vi "Condition _string_4_prod_count_month_2.vi"(0 "Form Date":timestamp format="%<%Y-%m-%d>T", 1 "To Date":timestamp format="%<%Y-%m-%d>T", 3 "Shift":string(combo)="ALL", 4 "Select Station":string(combo)="ST 1", 5 "STACKHOLDER_ID":i32, 6 "Select Stakeholder":string(combo), 7 "Refnum out 2":T1, 9 "error in (no error)":errorcluster, 10 "Select Month":string(combo), 12 "Select Year":string(combo)) -> (11 "error out":errorcluster, 13 "Refnum out":T1, 14 "sum":i32[](array[numeric]), 15 "all table":string[][](array[string]), 16 "PROD COUNT_TEST":string[](array[string]), 17 "Table":string[][](array[string]), 18 "Elements Found out":string[](array[string]), 19 "Array 3":string[][](array[string]))   [LabVIEW 2017]
uses:
  <vilib>/addons/database/Connection.llb/Conn ObjectReference.ctl
  <vilib>/addons/database/NI_Database_API.lvlib
panel:
  out "data out":string[][](array[string])
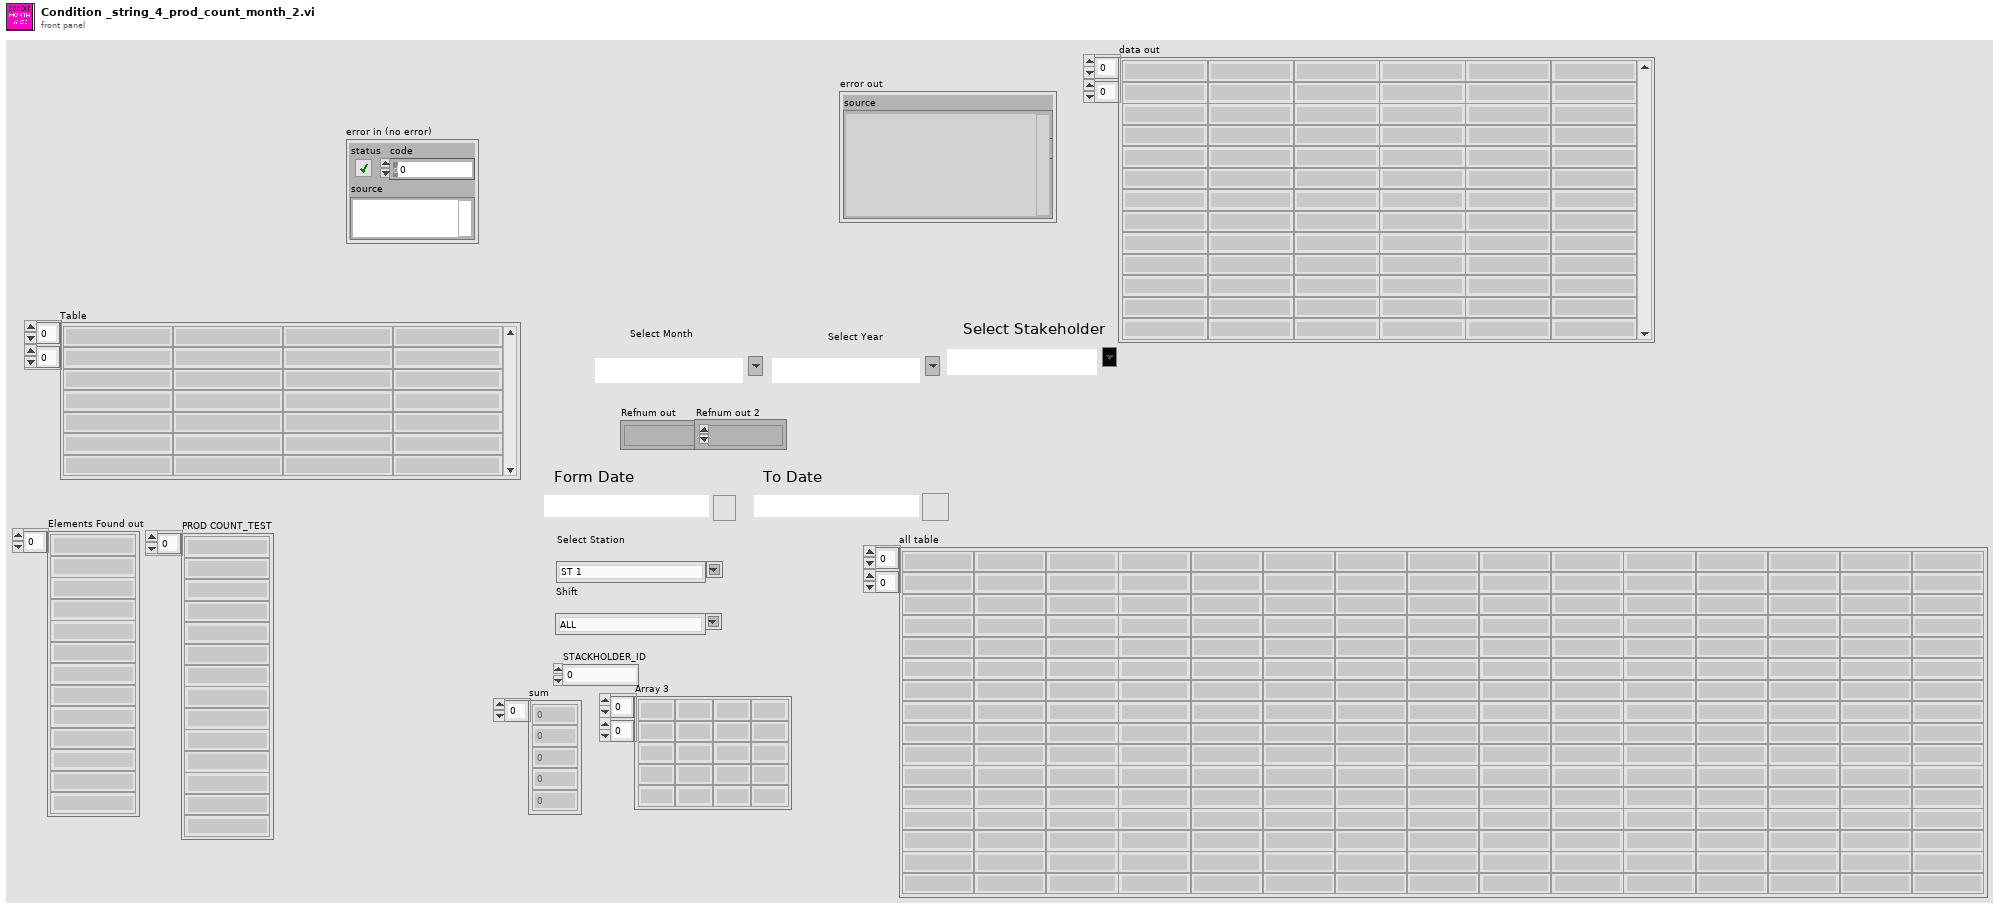
[diagram p1: front panel]
types:
  T1 = typedef "NI_Database_API.lvlib/Conn ObjectReference.ctl" = refnum<k1>
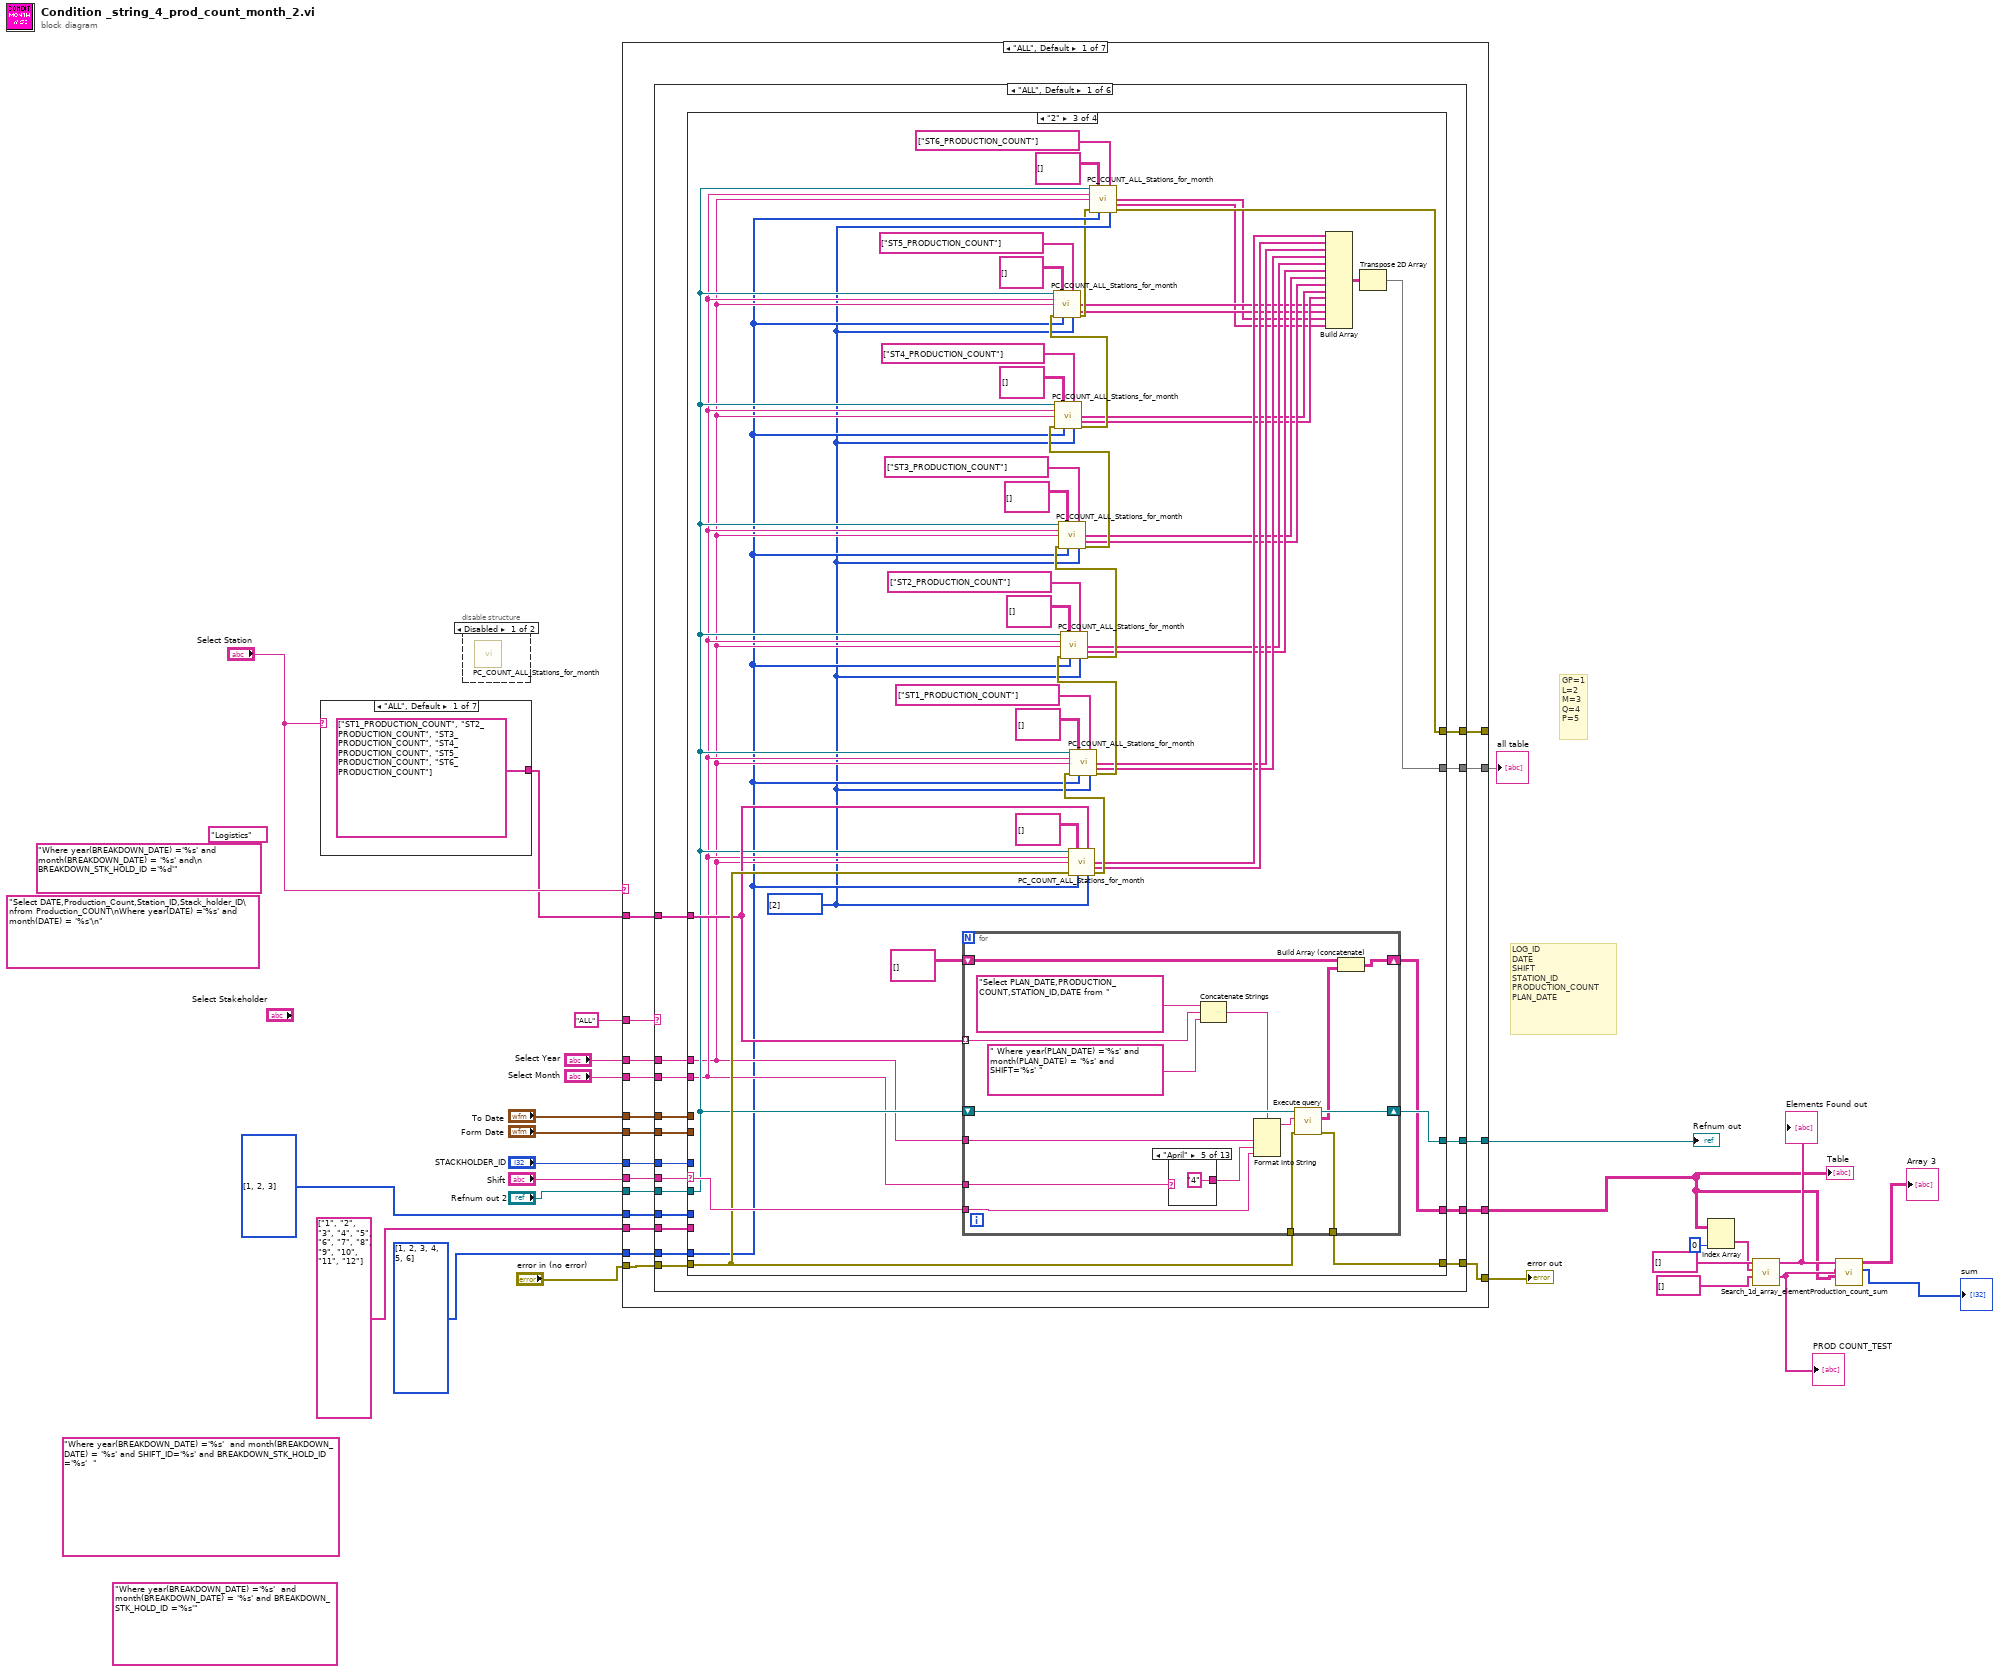
[diagram p0: block diagram]
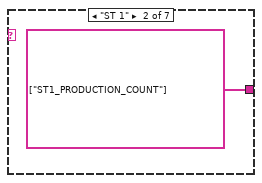
[diagram p3: hidden frame]
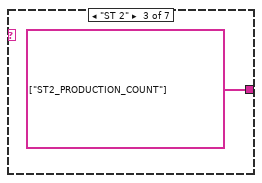
[diagram p4: hidden frame]
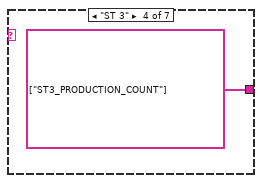
[diagram p5: hidden frame]
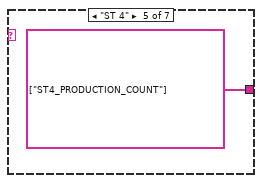
[diagram p6: hidden frame]
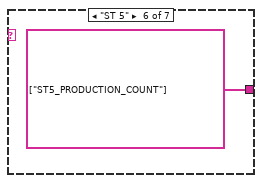
[diagram p7: hidden frame]
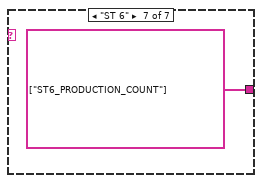
[diagram p8: hidden frame]
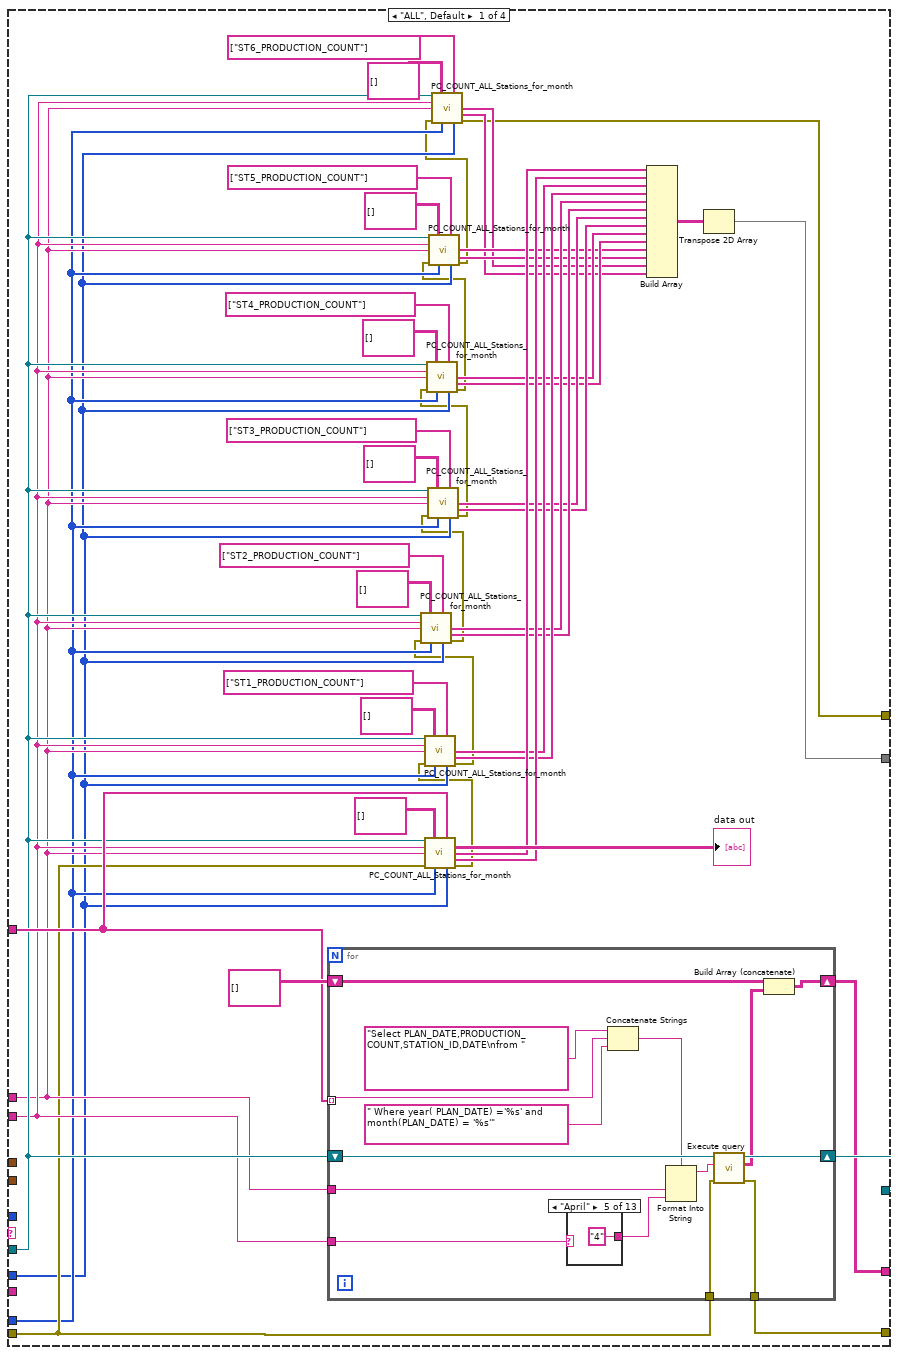
[diagram p9: hidden frame]
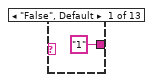
[diagram p10: hidden frame]
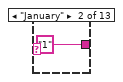
[diagram p11: hidden frame]
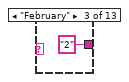
[diagram p12: hidden frame]
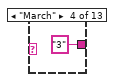
[diagram p13: hidden frame]
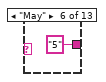
[diagram p14: hidden frame]
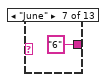
[diagram p15: hidden frame]
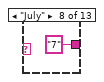
[diagram p16: hidden frame]
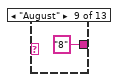
[diagram p17: hidden frame]
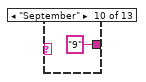
[diagram p18: hidden frame]
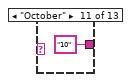
[diagram p19: hidden frame]
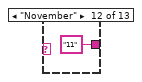
[diagram p20: hidden frame]
diagram:
  (unwired) "Select DATE,Production_Count,Station_ID,Stack_holder_ID\nfrom Production_COUNT\nWhere year(DATE) ='%s' and month(DATE) = '%s'\n" ("string")
  (unwired) "Where year(BREAKDOWN_DATE) ='%s' and month(BREAKDOWN_DATE) = '%s' and\n BREAKDOWN_STK_HOLD_ID ='%d'" ("condition")
  (unwired) "Logistics" ("Select Stakeholder")
  (unwired) "Where year(BREAKDOWN_DATE) ='%s'  and month(BREAKDOWN_DATE) = '%s' and BREAKDOWN_STK_HOLD_ID ='%s'" ("condition")
  (unwired) "Where year(BREAKDOWN_DATE) ='%s'  and month(BREAKDOWN_DATE) = '%s' and SHIFT_ID='%s' and BREAKDOWN_STK_HOLD_ID ='%s'  " ("condition")
  # "LOG_ID\nDATE\nSHIFT\nSTATION_ID\nPRODUCTION_COUNT\nPLAN_DATE"
  # "GP=1\nL=2\nM=3\nQ=4\nP=5"
  n1 = case shown="\"ALL\", Default" "Select Station" {
    tunnel: [string[] ["ST1_PRODUCTION_COUNT", "ST2_PRODUCTION_COUNT", "ST3_PRODUCTION_COUNT", "ST4_PRODUCTION_COUNT", "ST5_PRODUCTION_COUNT", "ST6_PRODUCTION_COUNT"] string[] ["ST1_PRODUCTION_COUNT"] string[] ["ST2_PRODUCTION_COUNT"] string[] ["ST3_PRODUCTION_COUNT"] string[] ["ST4_PRODUCTION_COUNT"] string[] ["ST5_PRODUCTION_COUNT"] string[] ["ST6_PRODUCTION_COUNT"]] -> w5
    frame "ALL", Default {
    }
    frame "ST 1" {
    }
    frame "ST 2" {
    }
    frame "ST 3" {
    }
    frame "ST 4" {
    }
    frame "ST 5" {
    }
    frame "ST 6" {
    }
  }
  n2 = disable-structure shown="Disabled" {
    frame Disabled {
      n3 = call "PC_COUNT_ALL_Stations_for_month.vi"() -> ()  [unwired: 11 in, 5 out]
    }
    frame Enabled {
    }
  }
  n4 = case shown="\"ALL\", Default" "Select Station" {
    tunnel: "Shift" -> [w51 w663 w1138 w1613 w2088 w2563 w3038]
    tunnel: "To Date" -> [w50 w662 w1137 w1612 w2087 w2562 w3037]
    tunnel: "Form Date" -> [w49 w661 w1136 w1611 w2086 w2561 w3036]
    tunnel: "STACKHOLDER_ID" -> [w48 w660 w1135 w1610 w2085 w2560 w3035]
    tunnel: "Refnum out 2" -> [w47 w659 w1134 w1609 w2084 w2559 w3034]
    tunnel: [w46 w658 w1133 w1608 w2083 w2558 w3033] -> w21
    tunnel: "ALL" -> [w45 w657 w1132 w1607 w2082 w2557 w3032]
    tunnel: i32[] [1, 2, 3, 4, 5, 6] -> [w44 _ _ _ _ _ _]
    tunnel: string[] ["1", "2", "3", "4", "5", "6", "7", "8", "9", "10", "11", "12"] -> [w43 _ _ _ _ _ _]
    tunnel: "Select Year" -> [w42 w656 w1131 w1606 w2081 w2556 w3031]
    tunnel: "Select Month" -> [w41 w655 w1130 w1605 w2080 w2555 w3030]
    tunnel: [w40 w654 w1129 w1604 w2079 w2554 w3029] -> w8
    tunnel: w5 -> [w39 w653 w1128 w1603 w2078 w2553 w3028]
    tunnel: "error in (no error)" -> [w38 w652 w1127 w1602 w2077 w2552 w3027]
    tunnel: [w37 w651 w1126 w1601 w2076 w2551 w3026] -> w3
    tunnel: i32[] [1, 2, 3] -> [w36 _ _ _ _ _ _]
    tunnel: [w35 _ _ _ _ _ _] -> w1
    tunnel: [w34 _ _ _ _ _ _] -> _
    frame "ALL", Default {
      n5 = case shown="\"ALL\", Default" w45 {
        tunnel: w51 -> [w68 w382 w437 w492 w547 w602]
        tunnel: w50 -> [w67 w381 w436 w491 w546 w601]
        tunnel: w49 -> [w66 w380 w435 w490 w545 w600]
        tunnel: w48 -> [w65 w379 w434 w489 w544 w599]
        tunnel: w47 -> [w64 w378 w433 w488 w543 w598]
        tunnel: [w63 w377 w432 w487 w542 w597] -> w46
        tunnel: w44 -> [w62 _ _ _ _ _]
        tunnel: w43 -> [w61 _ _ _ _ _]
        tunnel: w42 -> [w60 _ _ _ _ _]
        tunnel: w41 -> [w59 _ _ _ _ _]
        tunnel: [w58 _ _ _ _ _] -> w40
        tunnel: w39 -> [w57 _ _ _ _ _]
        tunnel: w38 -> [w56 w376 w431 w486 w541 w596]
        tunnel: [w55 w376 w431 w486 w541 w596] -> w37
        tunnel: w36 -> [w54 _ _ _ _ _]
        tunnel: [w53 _ _ _ _ _] -> w35
        tunnel: [w52 _ _ _ _ _] -> w34
        frame "ALL", Default {
          n6 = case shown="\"2\"" w68 {
            selector: w68 -> [_ w189 w266 w343]
            tunnel: w67 -> [_ _ _ _]
            tunnel: w66 -> [_ _ _ _]
            tunnel: w65 -> [_ _ _ _]
            tunnel: w64 -> [w83 w167 w244 w321]
            tunnel: [w116 w192 w269 w346] -> w63
            tunnel: w62 -> [w79 w164 w241 w318]
            tunnel: w61 -> [_ _ _ _]
            tunnel: w60 -> [w81 w165 w242 w319]
            tunnel: w59 -> [w82 w166 w243 w320]
            tunnel: [w114 w190 w267 w344] -> w58
            tunnel: w57 -> [w111 w185 w262 w339]
            tunnel: w56 -> [w80 w186 w263 w340]
            tunnel: [w113 w188 w265 w342] -> w55
            tunnel: w54 -> [w78 _ _ _]
            tunnel: [w106 w145 w222 w299] -> w53
            tunnel: [w69 w161 w238 w315] -> w52
            frame "ALL", Default {
              n7 = for {
                tunnel: w81 -> [w129]
                tunnel: w82 -> [w128]
                shift-right: [w130] -> w116
                shift-left: w83 -> [w131]
                tunnel: w111 -> [w124] mode=indexing
                shift-right: [w119] -> w114
                shift-left: string[][] [] -> [w121]
                tunnel: w80 -> [w118]
                tunnel: [w117] -> w113
                n8 = case shown="\"April\"" w128 {
                  tunnel: ["1" "1" "2" "3" "4" "5" "6" "7" "8" "9" "10" "11" "12"] -> w127
                  frame "False", Default {
                  }
                  frame "January" {
                  }
                  frame "February" {
                  }
                  frame "March" {
                  }
                  frame "April" {
                  }
                  frame "May" {
                  }
                  frame "June" {
                  }
                  frame "July" {
                  }
                  frame "August" {
                  }
                  frame "September" {
                  }
                  frame "October" {
                  }
                  frame "November" {
                  }
                  frame "December" {
                  }
                }
                n9 = Concatenate Strings("Select PLAN_DATE,PRODUCTION_COUNT,STATION_ID,DATE\nfrom ", w124, " Where year( PLAN_DATE) ='%s' and month(PLAN_DATE) = '%s'") -> (w122:string)
                n10 = Format Into String(format string=w122, w129, w127) -> (resulting string=w126:string)  [unwired: 2 in, 1 out]
                n11 = call "Execute query.vi"("error in (no error)"=w118, "String"=w126, "connection reference"=w131) -> ("error out"=w117:errorcluster, "Table"=w120:string[][], "connection reference 2"=w130:T1)  [unwired: 5 in, 1 out]
                n12 = Build Array (concatenate)(w121, w120) -> (w119:string[][])
              }
              n13 = call "PC_COUNT_ALL_Stations_for_month.vi"("Refnum in"=w83, "data in"=string[][] [] ("data"), "Array 3"=w111, "Select Month"=w82, "Select Year"=w81, "error in (no error)"=w80, "STATION"=w79, "SHIFT"=w78) -> ("data out"=→"data out":string[][], "DATE"=w109:string[], "COUNT"=w108:string[], "error out"=w75:errorcluster)  [unwired: 3 in, 1 out]
              n14 = call "PC_COUNT_ALL_Stations_for_month.vi"("Refnum in"=w83, "data in"=string[][] [] ("data"), "Array 3"=string[] ["ST1_PRODUCTION_COUNT"], "Select Month"=w82, "Select Year"=w81, "error in (no error)"=w75, "STATION"=w79, "SHIFT"=w78) -> ("DATE"=w103:string[], "COUNT"=w102:string[], "error out"=w74:errorcluster)  [unwired: 3 in, 2 out]
              n15 = call "PC_COUNT_ALL_Stations_for_month.vi"("Refnum in"=w83, "data in"=string[][] [] ("data"), "Array 3"=string[] ["ST2_PRODUCTION_COUNT"], "Select Month"=w82, "Select Year"=w81, "error in (no error)"=w74, "STATION"=w79, "SHIFT"=w78) -> ("DATE"=w99:string[], "COUNT"=w98:string[], "error out"=w73:errorcluster)  [unwired: 3 in, 2 out]
              n16 = call "PC_COUNT_ALL_Stations_for_month.vi"("Refnum in"=w83, "data in"=string[][] [] ("data"), "Array 3"=string[] ["ST3_PRODUCTION_COUNT"], "Select Month"=w82, "Select Year"=w81, "error in (no error)"=w73, "STATION"=w79, "SHIFT"=w78) -> ("DATE"=w95:string[], "COUNT"=w94:string[], "error out"=w72:errorcluster)  [unwired: 3 in, 2 out]
              n17 = call "PC_COUNT_ALL_Stations_for_month.vi"("Refnum in"=w83, "data in"=string[][] [] ("data"), "Array 3"=string[] ["ST4_PRODUCTION_COUNT"], "Select Month"=w82, "Select Year"=w81, "error in (no error)"=w72, "STATION"=w79, "SHIFT"=w78) -> ("DATE"=w91:string[], "COUNT"=w90:string[], "error out"=w71:errorcluster)  [unwired: 3 in, 2 out]
              n18 = call "PC_COUNT_ALL_Stations_for_month.vi"("Refnum in"=w83, "data in"=string[][] [] ("data"), "Array 3"=string[] ["ST5_PRODUCTION_COUNT"], "Select Month"=w82, "Select Year"=w81, "error in (no error)"=w71, "STATION"=w79, "SHIFT"=w78) -> ("DATE"=w87:string[], "COUNT"=w86:string[], "error out"=w70:errorcluster)  [unwired: 3 in, 2 out]
              n19 = call "PC_COUNT_ALL_Stations_for_month.vi"("Refnum in"=w83, "data in"=string[][] [] ("data"), "Array 3"=string[] ["ST6_PRODUCTION_COUNT"], "Select Month"=w82, "Select Year"=w81, "error in (no error)"=w70, "STATION"=w79, "SHIFT"=w78) -> ("DATE"=w77:string[], "COUNT"=w76:string[], "error out"=w69:errorcluster)  [unwired: 3 in, 2 out]
              n20 = Build Array(w109, w108, w103, w102, w99, w98, w95, w94, w91, w90, w87, w86, w77, w76) -> (w107:string[][])
              n21 = Transpose 2D Array(2D array=w107) -> (transposed array=w106:string[][])
            }
            frame "1" {
              w163 = i32[] [1]
              n22 = for {
                tunnel: w165 -> [w206]
                tunnel: w166 -> [w205]
                shift-right: [w207] -> w192
                shift-left: w167 -> [w208]
                tunnel: w185 -> [w201] mode=indexing
                shift-right: [w196] -> w190
                shift-left: string[][] [] -> [w198]
                tunnel: w189 -> [w195]
                tunnel: w186 -> [w194]
                tunnel: [w193] -> w188
                n23 = case shown="\"April\"" w205 {
                  tunnel: ["1" "1" "2" "3" "4" "5" "6" "7" "8" "9" "10" "11" "12"] -> w204
                  frame "False", Default {
                  }
                  frame "January" {
                  }
                  frame "February" {
                  }
                  frame "March" {
                  }
                  frame "April" {
                  }
                  frame "May" {
                  }
                  frame "June" {
                  }
                  frame "July" {
                  }
                  frame "August" {
                  }
                  frame "September" {
                  }
                  frame "October" {
                  }
                  frame "November" {
                  }
                  frame "December" {
                  }
                }
                n24 = Concatenate Strings("Select PLAN_DATE,PRODUCTION_COUNT,STATION_ID,DATE from ", w201, " Where year(PLAN_DATE) ='%s' and month(PLAN_DATE) = '%s' and SHIFT='%s' ") -> (w199:string)
                n25 = Format Into String(format string=w199, w206, w204, w195) -> (resulting string=w203:string)  [unwired: 2 in, 1 out]
                n26 = call "Execute query.vi"("error in (no error)"=w194, "String"=w203, "connection reference"=w208) -> ("error out"=w193:errorcluster, "Table"=w197:string[][], "connection reference 2"=w207:T1)  [unwired: 5 in, 1 out]
                n27 = Build Array (concatenate)(w198, w197) -> (w196:string[][])
              }
              n28 = call "PC_COUNT_ALL_Stations_for_month.vi"("Refnum in"=w167, "data in"=string[][] [], "Array 3"=w185, "Select Month"=w166, "Select Year"=w165, "error in (no error)"=w186, "STATION"=w164, "SHIFT"=w163) -> ("DATE"=w160:string[], "COUNT"=w159:string[], "error out"=w184:errorcluster)  [unwired: 3 in, 2 out]
              n29 = call "PC_COUNT_ALL_Stations_for_month.vi"("Refnum in"=w167, "data in"=string[][] [], "Array 3"=string[] ["ST1_PRODUCTION_COUNT"], "Select Month"=w166, "Select Year"=w165, "error in (no error)"=w184, "STATION"=w164, "SHIFT"=w163) -> ("DATE"=w158:string[], "COUNT"=w157:string[], "error out"=w179:errorcluster)  [unwired: 3 in, 2 out]
              n30 = call "PC_COUNT_ALL_Stations_for_month.vi"("Refnum in"=w167, "data in"=string[][] [], "Array 3"=string[] ["ST2_PRODUCTION_COUNT"], "Select Month"=w166, "Select Year"=w165, "error in (no error)"=w179, "STATION"=w164, "SHIFT"=w163) -> ("DATE"=w156:string[], "COUNT"=w155:string[], "error out"=w178:errorcluster)  [unwired: 3 in, 2 out]
              n31 = call "PC_COUNT_ALL_Stations_for_month.vi"("Refnum in"=w167, "data in"=string[][] [], "Array 3"=string[] ["ST3_PRODUCTION_COUNT"], "Select Month"=w166, "Select Year"=w165, "error in (no error)"=w178, "STATION"=w164, "SHIFT"=w163) -> ("DATE"=w154:string[], "COUNT"=w153:string[], "error out"=w175:errorcluster)  [unwired: 3 in, 2 out]
              n32 = call "PC_COUNT_ALL_Stations_for_month.vi"("Refnum in"=w167, "data in"=string[][] [], "Array 3"=string[] ["ST4_PRODUCTION_COUNT"], "Select Month"=w166, "Select Year"=w165, "error in (no error)"=w175, "STATION"=w164, "SHIFT"=w163) -> ("DATE"=w152:string[], "COUNT"=w151:string[], "error out"=w170:errorcluster)  [unwired: 3 in, 2 out]
              n33 = call "PC_COUNT_ALL_Stations_for_month.vi"("Refnum in"=w167, "data in"=string[][] [], "Array 3"=string[] ["ST5_PRODUCTION_COUNT"], "Select Month"=w166, "Select Year"=w165, "error in (no error)"=w170, "STATION"=w164, "SHIFT"=w163) -> ("DATE"=w150:string[], "COUNT"=w149:string[], "error out"=w162:errorcluster)  [unwired: 3 in, 2 out]
              n34 = call "PC_COUNT_ALL_Stations_for_month.vi"("Refnum in"=w167, "data in"=string[][] [], "Array 3"=string[] ["ST6_PRODUCTION_COUNT"], "Select Month"=w166, "Select Year"=w165, "error in (no error)"=w162, "STATION"=w164, "SHIFT"=w163) -> ("DATE"=w148:string[], "COUNT"=w147:string[], "error out"=w161:errorcluster)  [unwired: 3 in, 2 out]
              n35 = Build Array(w160, w159, w158, w157, w156, w155, w154, w153, w152, w151, w150, w149, w148, w147) -> (w146:string[][])
              n36 = Transpose 2D Array(2D array=w146) -> (transposed array=w145:string[][])
            }
            frame "2" {
              w240 = i32[] [2]
              n37 = for {
                tunnel: w242 -> [w283]
                tunnel: w243 -> [w282]
                shift-right: [w284] -> w269
                shift-left: w244 -> [w285]
                tunnel: w262 -> [w278] mode=indexing
                shift-right: [w273] -> w267
                shift-left: string[][] [] -> [w275]
                tunnel: w266 -> [w272]
                tunnel: w263 -> [w271]
                tunnel: [w270] -> w265
                n38 = case shown="\"April\"" w282 {
                  tunnel: ["1" "1" "2" "3" "4" "5" "6" "7" "8" "9" "10" "11" "12"] -> w281
                  frame "False", Default {
                  }
                  frame "January" {
                  }
                  frame "February" {
                  }
                  frame "March" {
                  }
                  frame "April" {
                  }
                  frame "May" {
                  }
                  frame "June" {
                  }
                  frame "July" {
                  }
                  frame "August" {
                  }
                  frame "September" {
                  }
                  frame "October" {
                  }
                  frame "November" {
                  }
                  frame "December" {
                  }
                }
                n39 = Concatenate Strings("Select PLAN_DATE,PRODUCTION_COUNT,STATION_ID,DATE from ", w278, " Where year(PLAN_DATE) ='%s' and month(PLAN_DATE) = '%s' and SHIFT='%s' ") -> (w276:string)
                n40 = Format Into String(format string=w276, w283, w281, w272) -> (resulting string=w280:string)  [unwired: 2 in, 1 out]
                n41 = call "Execute query.vi"("error in (no error)"=w271, "String"=w280, "connection reference"=w285) -> ("error out"=w270:errorcluster, "Table"=w274:string[][], "connection reference 2"=w284:T1)  [unwired: 5 in, 1 out]
                n42 = Build Array (concatenate)(w275, w274) -> (w273:string[][])
              }
              n43 = call "PC_COUNT_ALL_Stations_for_month.vi"("Refnum in"=w244, "data in"=string[][] [], "Array 3"=w262, "Select Month"=w243, "Select Year"=w242, "error in (no error)"=w263, "STATION"=w241, "SHIFT"=w240) -> ("DATE"=w237:string[], "COUNT"=w236:string[], "error out"=w261:errorcluster)  [unwired: 3 in, 2 out]
              n44 = call "PC_COUNT_ALL_Stations_for_month.vi"("Refnum in"=w244, "data in"=string[][] [], "Array 3"=string[] ["ST1_PRODUCTION_COUNT"], "Select Month"=w243, "Select Year"=w242, "error in (no error)"=w261, "STATION"=w241, "SHIFT"=w240) -> ("DATE"=w235:string[], "COUNT"=w234:string[], "error out"=w256:errorcluster)  [unwired: 3 in, 2 out]
              n45 = call "PC_COUNT_ALL_Stations_for_month.vi"("Refnum in"=w244, "data in"=string[][] [], "Array 3"=string[] ["ST2_PRODUCTION_COUNT"], "Select Month"=w243, "Select Year"=w242, "error in (no error)"=w256, "STATION"=w241, "SHIFT"=w240) -> ("DATE"=w233:string[], "COUNT"=w232:string[], "error out"=w255:errorcluster)  [unwired: 3 in, 2 out]
              n46 = call "PC_COUNT_ALL_Stations_for_month.vi"("Refnum in"=w244, "data in"=string[][] [], "Array 3"=string[] ["ST3_PRODUCTION_COUNT"], "Select Month"=w243, "Select Year"=w242, "error in (no error)"=w255, "STATION"=w241, "SHIFT"=w240) -> ("DATE"=w231:string[], "COUNT"=w230:string[], "error out"=w252:errorcluster)  [unwired: 3 in, 2 out]
              n47 = call "PC_COUNT_ALL_Stations_for_month.vi"("Refnum in"=w244, "data in"=string[][] [], "Array 3"=string[] ["ST4_PRODUCTION_COUNT"], "Select Month"=w243, "Select Year"=w242, "error in (no error)"=w252, "STATION"=w241, "SHIFT"=w240) -> ("DATE"=w229:string[], "COUNT"=w228:string[], "error out"=w247:errorcluster)  [unwired: 3 in, 2 out]
              n48 = call "PC_COUNT_ALL_Stations_for_month.vi"("Refnum in"=w244, "data in"=string[][] [], "Array 3"=string[] ["ST5_PRODUCTION_COUNT"], "Select Month"=w243, "Select Year"=w242, "error in (no error)"=w247, "STATION"=w241, "SHIFT"=w240) -> ("DATE"=w227:string[], "COUNT"=w226:string[], "error out"=w239:errorcluster)  [unwired: 3 in, 2 out]
              n49 = call "PC_COUNT_ALL_Stations_for_month.vi"("Refnum in"=w244, "data in"=string[][] [], "Array 3"=string[] ["ST6_PRODUCTION_COUNT"], "Select Month"=w243, "Select Year"=w242, "error in (no error)"=w239, "STATION"=w241, "SHIFT"=w240) -> ("DATE"=w225:string[], "COUNT"=w224:string[], "error out"=w238:errorcluster)  [unwired: 3 in, 2 out]
              n50 = Build Array(w237, w236, w235, w234, w233, w232, w231, w230, w229, w228, w227, w226, w225, w224) -> (w223:string[][])
              n51 = Transpose 2D Array(2D array=w223) -> (transposed array=w222:string[][])
            }
            frame "3" {
              w317 = i32[] [3]
              n52 = for {
                tunnel: w319 -> [w360]
                tunnel: w320 -> [w359]
                shift-right: [w361] -> w346
                shift-left: w321 -> [w362]
                tunnel: w339 -> [w355] mode=indexing
                shift-right: [w350] -> w344
                shift-left: string[][] [] -> [w352]
                tunnel: w343 -> [w349]
                tunnel: w340 -> [w348]
                tunnel: [w347] -> w342
                n53 = case shown="\"April\"" w359 {
                  tunnel: ["1" "1" "2" "3" "4" "5" "6" "7" "8" "9" "10" "11" "12"] -> w358
                  frame "False", Default {
                  }
                  frame "January" {
                  }
                  frame "February" {
                  }
                  frame "March" {
                  }
                  frame "April" {
                  }
                  frame "May" {
                  }
                  frame "June" {
                  }
                  frame "July" {
                  }
                  frame "August" {
                  }
                  frame "September" {
                  }
                  frame "October" {
                  }
                  frame "November" {
                  }
                  frame "December" {
                  }
                }
                n54 = Concatenate Strings("Select PLAN_DATE,PRODUCTION_COUNT,STATION_ID,DATE from ", w355, " Where year(PLAN_DATE) ='%s' and month(PLAN_DATE) = '%s' and SHIFT='%s' ") -> (w353:string)
                n55 = Format Into String(format string=w353, w360, w358, w349) -> (resulting string=w357:string)  [unwired: 2 in, 1 out]
                n56 = call "Execute query.vi"("error in (no error)"=w348, "String"=w357, "connection reference"=w362) -> ("error out"=w347:errorcluster, "Table"=w351:string[][], "connection reference 2"=w361:T1)  [unwired: 5 in, 1 out]
                n57 = Build Array (concatenate)(w352, w351) -> (w350:string[][])
              }
              n58 = call "PC_COUNT_ALL_Stations_for_month.vi"("Refnum in"=w321, "data in"=string[][] [], "Array 3"=w339, "Select Month"=w320, "Select Year"=w319, "error in (no error)"=w340, "STATION"=w318, "SHIFT"=w317) -> ("DATE"=w314:string[], "COUNT"=w313:string[], "error out"=w338:errorcluster)  [unwired: 3 in, 2 out]
              n59 = call "PC_COUNT_ALL_Stations_for_month.vi"("Refnum in"=w321, "data in"=string[][] [], "Array 3"=string[] ["ST1_PRODUCTION_COUNT"], "Select Month"=w320, "Select Year"=w319, "error in (no error)"=w338, "STATION"=w318, "SHIFT"=w317) -> ("DATE"=w312:string[], "COUNT"=w311:string[], "error out"=w333:errorcluster)  [unwired: 3 in, 2 out]
              n60 = call "PC_COUNT_ALL_Stations_for_month.vi"("Refnum in"=w321, "data in"=string[][] [], "Array 3"=string[] ["ST2_PRODUCTION_COUNT"], "Select Month"=w320, "Select Year"=w319, "error in (no error)"=w333, "STATION"=w318, "SHIFT"=w317) -> ("DATE"=w310:string[], "COUNT"=w309:string[], "error out"=w332:errorcluster)  [unwired: 3 in, 2 out]
              n61 = call "PC_COUNT_ALL_Stations_for_month.vi"("Refnum in"=w321, "data in"=string[][] [], "Array 3"=string[] ["ST3_PRODUCTION_COUNT"], "Select Month"=w320, "Select Year"=w319, "error in (no error)"=w332, "STATION"=w318, "SHIFT"=w317) -> ("DATE"=w308:string[], "COUNT"=w307:string[], "error out"=w329:errorcluster)  [unwired: 3 in, 2 out]
              n62 = call "PC_COUNT_ALL_Stations_for_month.vi"("Refnum in"=w321, "data in"=string[][] [], "Array 3"=string[] ["ST4_PRODUCTION_COUNT"], "Select Month"=w320, "Select Year"=w319, "error in (no error)"=w329, "STATION"=w318, "SHIFT"=w317) -> ("DATE"=w306:string[], "COUNT"=w305:string[], "error out"=w324:errorcluster)  [unwired: 3 in, 2 out]
              n63 = call "PC_COUNT_ALL_Stations_for_month.vi"("Refnum in"=w321, "data in"=string[][] [], "Array 3"=string[] ["ST5_PRODUCTION_COUNT"], "Select Month"=w320, "Select Year"=w319, "error in (no error)"=w324, "STATION"=w318, "SHIFT"=w317) -> ("DATE"=w304:string[], "COUNT"=w303:string[], "error out"=w316:errorcluster)  [unwired: 3 in, 2 out]
              n64 = call "PC_COUNT_ALL_Stations_for_month.vi"("Refnum in"=w321, "data in"=string[][] [], "Array 3"=string[] ["ST6_PRODUCTION_COUNT"], "Select Month"=w320, "Select Year"=w319, "error in (no error)"=w316, "STATION"=w318, "SHIFT"=w317) -> ("DATE"=w302:string[], "COUNT"=w301:string[], "error out"=w315:errorcluster)  [unwired: 3 in, 2 out]
              n65 = Build Array(w314, w313, w312, w311, w310, w309, w308, w307, w306, w305, w304, w303, w302, w301) -> (w300:string[][])
              n66 = Transpose 2D Array(2D array=w300) -> (transposed array=w299:string[][])
            }
          }
        }
        frame "Logistics" {
          n67 = case shown="\"3\"" w382 {
            selector: w382 -> [_ _ w396 w408 w420]
            tunnel: w381 -> [_ w393 w405 w417 w429]
            tunnel: w380 -> [_ w392 w404 w416 w428]
            tunnel: w379 -> [_ _ _ _ _]
            tunnel: [_ w386 w398 w410 w422] -> _
            tunnel: w378 -> [w383 w389 w401 w413 w425]
            tunnel: [w383 w385 w397 w409 w421] -> w377
            frame "False", Default {
            }
            frame "ALL" {
              w394 = "%Y-%m-%d " ("time format string (%c)")
              n68 = Format Date/Time String(time format string (%c)=w394, seconds (now)=w392) -> (date/time string=w391:string)  [unwired: 1 in]
              n69 = Format Date/Time String(time format string (%c)=w394, seconds (now)=w393) -> (date/time string=w390:string)  [unwired: 1 in]
              n70 = Format Into String(format string="Select DATE,Production_Count,Station_ID,Stack_holder_ID\nfrom Production_COUNT\nWhere DATE between '%s' and '%s' and Stack_holder_ID='%d'" ("string"), w391, w390, 2 ("input 3")) -> (resulting string=w387:string)  [unwired: 2 in, 1 out]
              n71 = call "Execute query.vi"("String"=w387, "connection reference"=w389) -> ("Table"=w386:string[][], "connection reference 2"=w385:T1)  [unwired: 6 in, 2 out]
            }
            frame "1" {
              w406 = "%Y-%m-%d " ("time format string (%c)")
              n72 = Format Date/Time String(time format string (%c)=w406, seconds (now)=w405) -> (date/time string=w402:string)  [unwired: 1 in]
              n73 = Format Date/Time String(time format string (%c)=w406, seconds (now)=w404) -> (date/time string=w403:string)  [unwired: 1 in]
              n74 = Format Into String(format string="Select DATE,Production_Count,Station_ID,Stack_holder_ID\nfrom Production_COUNT\nWhere DATE between '%s' and '%s' and Shift_ID='%s'and Stack_holder_ID='%d'" ("string"), w403, w402, w396, 2 ("input 4")) -> (resulting string=w399:string)  [unwired: 2 in, 1 out]
              n75 = call "Execute query.vi"("String"=w399, "connection reference"=w401) -> ("Table"=w398:string[][], "connection reference 2"=w397:T1)  [unwired: 6 in, 2 out]
            }
            frame "2" {
              w418 = "%Y-%m-%d " ("time format string (%c)")
              n76 = Format Date/Time String(time format string (%c)=w418, seconds (now)=w417) -> (date/time string=w414:string)  [unwired: 1 in]
              n77 = Format Date/Time String(time format string (%c)=w418, seconds (now)=w416) -> (date/time string=w415:string)  [unwired: 1 in]
              n78 = Format Into String(format string="Select DATE,Production_Count,Station_ID,Stack_holder_ID\nfrom Production_COUNT\nWhere DATE between '%s' and '%s' and Shift_ID='%s'and Stack_holder_ID='%d'" ("string"), w415, w414, w408, 2 ("input 4")) -> (resulting string=w411:string)  [unwired: 2 in, 1 out]
              n79 = call "Execute query.vi"("String"=w411, "connection reference"=w413) -> ("Table"=w410:string[][], "connection reference 2"=w409:T1)  [unwired: 6 in, 2 out]
            }
            frame "3" {
              w430 = "%Y-%m-%d " ("time format string (%c)")
              n80 = Format Date/Time String(time format string (%c)=w430, seconds (now)=w429) -> (date/time string=w426:string)  [unwired: 1 in]
              n81 = Format Date/Time String(time format string (%c)=w430, seconds (now)=w428) -> (date/time string=w427:string)  [unwired: 1 in]
              n82 = Format Into String(format string="Select DATE,Production_Count,Station_ID,Stack_holder_ID\nfrom Production_COUNT\nWhere DATE between '%s' and '%s' and Shift_ID='%s'and Stack_holder_ID='%d'" ("string"), w427, w426, w420, 2 ("input 4")) -> (resulting string=w423:string)  [unwired: 2 in, 1 out]
              n83 = call "Execute query.vi"("String"=w423, "connection reference"=w425) -> ("Table"=w422:string[][], "connection reference 2"=w421:T1)  [unwired: 6 in, 2 out]
            }
          }
        }
        frame "Gap Leader" {
          n84 = case shown="\"3\"" w437 {
            selector: w437 -> [_ _ w451 w463 w475]
            tunnel: w436 -> [_ w448 w460 w472 w484]
            tunnel: w435 -> [_ w447 w459 w471 w483]
            tunnel: w434 -> [_ _ _ _ _]
            tunnel: [_ w441 w453 w465 w477] -> _
            tunnel: w433 -> [w438 w444 w456 w468 w480]
            tunnel: [w438 w440 w452 w464 w476] -> w432
            frame "False", Default {
            }
            frame "ALL" {
              w449 = "%Y-%m-%d " ("time format string (%c)")
              n85 = Format Date/Time String(time format string (%c)=w449, seconds (now)=w447) -> (date/time string=w446:string)  [unwired: 1 in]
              n86 = Format Date/Time String(time format string (%c)=w449, seconds (now)=w448) -> (date/time string=w445:string)  [unwired: 1 in]
              n87 = Format Into String(format string="Select DATE,Production_Count,Station_ID,Stack_holder_ID\nfrom Production_COUNT\nWhere DATE between '%s' and '%s' and Stack_holder_ID='%d'" ("string"), w446, w445, 1 ("input 3")) -> (resulting string=w442:string)  [unwired: 2 in, 1 out]
              n88 = call "Execute query.vi"("String"=w442, "connection reference"=w444) -> ("Table"=w441:string[][], "connection reference 2"=w440:T1)  [unwired: 6 in, 2 out]
            }
            frame "1" {
              w461 = "%Y-%m-%d " ("time format string (%c)")
              n89 = Format Date/Time String(time format string (%c)=w461, seconds (now)=w460) -> (date/time string=w457:string)  [unwired: 1 in]
              n90 = Format Date/Time String(time format string (%c)=w461, seconds (now)=w459) -> (date/time string=w458:string)  [unwired: 1 in]
              n91 = Format Into String(format string="Select DATE,Production_Count,Station_ID,Stack_holder_ID\nfrom Production_COUNT\nWhere DATE between '%s' and '%s' and Shift_ID='%s'and Stack_holder_ID='%d'" ("string"), w458, w457, w451, 1 ("input 4")) -> (resulting string=w454:string)  [unwired: 2 in, 1 out]
              n92 = call "Execute query.vi"("String"=w454, "connection reference"=w456) -> ("Table"=w453:string[][], "connection reference 2"=w452:T1)  [unwired: 6 in, 2 out]
            }
            frame "2" {
              w473 = "%Y-%m-%d " ("time format string (%c)")
              n93 = Format Date/Time String(time format string (%c)=w473, seconds (now)=w472) -> (date/time string=w469:string)  [unwired: 1 in]
              n94 = Format Date/Time String(time format string (%c)=w473, seconds (now)=w471) -> (date/time string=w470:string)  [unwired: 1 in]
              n95 = Format Into String(format string="Select DATE,Production_Count,Station_ID,Stack_holder_ID\nfrom Production_COUNT\nWhere DATE between '%s' and '%s' and Shift_ID='%s'and Stack_holder_ID='%d'" ("string"), w470, w469, w463, 1 ("input 4")) -> (resulting string=w466:string)  [unwired: 2 in, 1 out]
              n96 = call "Execute query.vi"("String"=w466, "connection reference"=w468) -> ("Table"=w465:string[][], "connection reference 2"=w464:T1)  [unwired: 6 in, 2 out]
            }
            frame "3" {
              w485 = "%Y-%m-%d " ("time format string (%c)")
              n97 = Format Date/Time String(time format string (%c)=w485, seconds (now)=w484) -> (date/time string=w481:string)  [unwired: 1 in]
              n98 = Format Date/Time String(time format string (%c)=w485, seconds (now)=w483) -> (date/time string=w482:string)  [unwired: 1 in]
              n99 = Format Into String(format string="Select DATE,Production_Count,Station_ID,Stack_holder_ID\nfrom Production_COUNT\nWhere DATE between '%s' and '%s' and Shift_ID='%s'and Stack_holder_ID='%d'" ("string"), w482, w481, w475, 1 ("input 4")) -> (resulting string=w478:string)  [unwired: 2 in, 1 out]
              n100 = call "Execute query.vi"("String"=w478, "connection reference"=w480) -> ("Table"=w477:string[][], "connection reference 2"=w476:T1)  [unwired: 6 in, 2 out]
            }
          }
        }
        frame "Maintenance" {
          n101 = case shown="\"ALL\"" w492 {
            selector: w492 -> [_ _ w506 w518 w530]
            tunnel: w491 -> [_ w503 w515 w527 w539]
            tunnel: w490 -> [_ w502 w514 w526 w538]
            tunnel: w489 -> [_ _ _ _ _]
            tunnel: [_ w496 w508 w520 w532] -> _
            tunnel: w488 -> [w493 w499 w511 w523 w535]
            tunnel: [w493 w495 w507 w519 w531] -> w487
            frame "False", Default {
            }
            frame "ALL" {
              w504 = "%Y-%m-%d " ("time format string (%c)")
              n102 = Format Date/Time String(time format string (%c)=w504, seconds (now)=w502) -> (date/time string=w501:string)  [unwired: 1 in]
              n103 = Format Date/Time String(time format string (%c)=w504, seconds (now)=w503) -> (date/time string=w500:string)  [unwired: 1 in]
              n104 = Format Into String(format string="Select DATE,Production_Count,Station_ID,Stack_holder_ID\nfrom Production_COUNT\nWhere DATE between '%s' and '%s' and Stack_holder_ID='%d'" ("string"), w501, w500, 3 ("input 3")) -> (resulting string=w497:string)  [unwired: 2 in, 1 out]
              n105 = call "Execute query.vi"("String"=w497, "connection reference"=w499) -> ("Table"=w496:string[][], "connection reference 2"=w495:T1)  [unwired: 6 in, 2 out]
            }
            frame "1" {
              w516 = "%Y-%m-%d " ("time format string (%c)")
              n106 = Format Date/Time String(time format string (%c)=w516, seconds (now)=w515) -> (date/time string=w512:string)  [unwired: 1 in]
              n107 = Format Date/Time String(time format string (%c)=w516, seconds (now)=w514) -> (date/time string=w513:string)  [unwired: 1 in]
              n108 = Format Into String(format string="Select DATE,Production_Count,Station_ID,Stack_holder_ID\nfrom Production_COUNT\nWhere DATE between '%s' and '%s' and Shift_ID='%s'and Stack_holder_ID='%d'" ("string"), w513, w512, w506, 3 ("input 4")) -> (resulting string=w509:string)  [unwired: 2 in, 1 out]
              n109 = call "Execute query.vi"("String"=w509, "connection reference"=w511) -> ("Table"=w508:string[][], "connection reference 2"=w507:T1)  [unwired: 6 in, 2 out]
            }
            frame "2" {
              w528 = "%Y-%m-%d " ("time format string (%c)")
              n110 = Format Date/Time String(time format string (%c)=w528, seconds (now)=w527) -> (date/time string=w524:string)  [unwired: 1 in]
              n111 = Format Date/Time String(time format string (%c)=w528, seconds (now)=w526) -> (date/time string=w525:string)  [unwired: 1 in]
              n112 = Format Into String(format string="Select DATE,Production_Count,Station_ID,Stack_holder_ID\nfrom Production_COUNT\nWhere DATE between '%s' and '%s' and Shift_ID='%s'and Stack_holder_ID='%d'" ("string"), w525, w524, w518, 3 ("input 4")) -> (resulting string=w521:string)  [unwired: 2 in, 1 out]
              n113 = call "Execute query.vi"("String"=w521, "connection reference"=w523) -> ("Table"=w520:string[][], "connection reference 2"=w519:T1)  [unwired: 6 in, 2 out]
            }
            frame "3" {
              w540 = "%Y-%m-%d " ("time format string (%c)")
              n114 = Format Date/Time String(time format string (%c)=w540, seconds (now)=w539) -> (date/time string=w536:string)  [unwired: 1 in]
              n115 = Format Date/Time String(time format string (%c)=w540, seconds (now)=w538) -> (date/time string=w537:string)  [unwired: 1 in]
              n116 = Format Into String(format string="Select DATE,Production_Count,Station_ID,Stack_holder_ID\nfrom Production_COUNT\nWhere DATE between '%s' and '%s' and Shift_ID='%s'and Stack_holder_ID='%d'" ("string"), w537, w536, w530, 3 ("input 4")) -> (resulting string=w533:string)  [unwired: 2 in, 1 out]
              n117 = call "Execute query.vi"("String"=w533, "connection reference"=w535) -> ("Table"=w532:string[][], "connection reference 2"=w531:T1)  [unwired: 6 in, 2 out]
            }
          }
        }
        frame "Quality" {
          n118 = case shown="\"3\"" w547 {
            selector: w547 -> [_ _ w561 w573 w585]
            tunnel: w546 -> [_ w558 w570 w582 w594]
            tunnel: w545 -> [_ w557 w569 w581 w593]
            tunnel: w544 -> [_ _ _ _ _]
            tunnel: [_ w551 w563 w575 w587] -> _
            tunnel: w543 -> [w548 w554 w566 w578 w590]
            tunnel: [w548 w550 w562 w574 w586] -> w542
            frame "False", Default {
            }
            frame "ALL" {
              w559 = "%Y-%m-%d " ("time format string (%c)")
              n119 = Format Date/Time String(time format string (%c)=w559, seconds (now)=w557) -> (date/time string=w556:string)  [unwired: 1 in]
              n120 = Format Date/Time String(time format string (%c)=w559, seconds (now)=w558) -> (date/time string=w555:string)  [unwired: 1 in]
              n121 = Format Into String(format string="Select DATE,Production_Count,Station_ID,Stack_holder_ID\nfrom Production_COUNT\nWhere DATE between '%s' and '%s' and Stack_holder_ID='%d'" ("string"), w556, w555, 4 ("input 3")) -> (resulting string=w552:string)  [unwired: 2 in, 1 out]
              n122 = call "Execute query.vi"("String"=w552, "connection reference"=w554) -> ("Table"=w551:string[][], "connection reference 2"=w550:T1)  [unwired: 6 in, 2 out]
            }
            frame "1" {
              w571 = "%Y-%m-%d " ("time format string (%c)")
              n123 = Format Date/Time String(time format string (%c)=w571, seconds (now)=w570) -> (date/time string=w567:string)  [unwired: 1 in]
              n124 = Format Date/Time String(time format string (%c)=w571, seconds (now)=w569) -> (date/time string=w568:string)  [unwired: 1 in]
              n125 = Format Into String(format string="Select DATE,Production_Count,Station_ID,Stack_holder_ID\nfrom Production_COUNT\nWhere DATE between '%s' and '%s' and Shift_ID='%s'and Stack_holder_ID='%d'" ("string"), w568, w567, w561, 4 ("input 4")) -> (resulting string=w564:string)  [unwired: 2 in, 1 out]
              n126 = call "Execute query.vi"("String"=w564, "connection reference"=w566) -> ("Table"=w563:string[][], "connection reference 2"=w562:T1)  [unwired: 6 in, 2 out]
            }
            frame "2" {
              w583 = "%Y-%m-%d " ("time format string (%c)")
              n127 = Format Date/Time String(time format string (%c)=w583, seconds (now)=w582) -> (date/time string=w579:string)  [unwired: 1 in]
              n128 = Format Date/Time String(time format string (%c)=w583, seconds (now)=w581) -> (date/time string=w580:string)  [unwired: 1 in]
              n129 = Format Into String(format string="Select DATE,Production_Count,Station_ID,Stack_holder_ID\nfrom Production_COUNT\nWhere DATE between '%s' and '%s' and Shift_ID='%s'and Stack_holder_ID='%d'" ("string"), w580, w579, w573, 4 ("input 4")) -> (resulting string=w576:string)  [unwired: 2 in, 1 out]
              n130 = call "Execute query.vi"("String"=w576, "connection reference"=w578) -> ("Table"=w575:string[][], "connection reference 2"=w574:T1)  [unwired: 6 in, 2 out]
            }
            frame "3" {
              w595 = "%Y-%m-%d " ("time format string (%c)")
              n131 = Format Date/Time String(time format string (%c)=w595, seconds (now)=w594) -> (date/time string=w591:string)  [unwired: 1 in]
              n132 = Format Date/Time String(time format string (%c)=w595, seconds (now)=w593) -> (date/time string=w592:string)  [unwired: 1 in]
              n133 = Format Into String(format string="Select DATE,Production_Count,Station_ID,Stack_holder_ID\nfrom Production_COUNT\nWhere DATE between '%s' and '%s' and Shift_ID='%s'and Stack_holder_ID='%d'" ("string"), w592, w591, w585, 4 ("input 4")) -> (resulting string=w588:string)  [unwired: 2 in, 1 out]
              n134 = call "Execute query.vi"("String"=w588, "connection reference"=w590) -> ("Table"=w587:string[][], "connection reference 2"=w586:T1)  [unwired: 6 in, 2 out]
            }
          }
        }
        frame "Production" {
          n135 = case shown="\"3\"" w602 {
            selector: w602 -> [_ _ w616 w628 w640]
            tunnel: w601 -> [_ w613 w625 w637 w649]
            tunnel: w600 -> [_ w612 w624 w636 w648]
            tunnel: w599 -> [_ _ _ _ _]
            tunnel: [_ w606 w618 w630 w642] -> _
            tunnel: w598 -> [w603 w609 w621 w633 w645]
            tunnel: [w603 w605 w617 w629 w641] -> w597
            frame "False", Default {
            }
            frame "ALL" {
              w614 = "%Y-%m-%d " ("time format string (%c)")
              n136 = Format Date/Time String(time format string (%c)=w614, seconds (now)=w612) -> (date/time string=w611:string)  [unwired: 1 in]
              n137 = Format Date/Time String(time format string (%c)=w614, seconds (now)=w613) -> (date/time string=w610:string)  [unwired: 1 in]
              n138 = Format Into String(format string="Select DATE,Production_Count,Station_ID,Stack_holder_ID\nfrom Production_COUNT\nWhere DATE between '%s' and '%s' and Stack_holder_ID='%d'" ("string"), w611, w610, 5 ("input 3")) -> (resulting string=w607:string)  [unwired: 2 in, 1 out]
              n139 = call "Execute query.vi"("String"=w607, "connection reference"=w609) -> ("Table"=w606:string[][], "connection reference 2"=w605:T1)  [unwired: 6 in, 2 out]
            }
            frame "1" {
              w626 = "%Y-%m-%d " ("time format string (%c)")
              n140 = Format Date/Time String(time format string (%c)=w626, seconds (now)=w625) -> (date/time string=w622:string)  [unwired: 1 in]
              n141 = Format Date/Time String(time format string (%c)=w626, seconds (now)=w624) -> (date/time string=w623:string)  [unwired: 1 in]
              n142 = Format Into String(format string="Select DATE,Production_Count,Station_ID,Stack_holder_ID\nfrom Production_COUNT\nWhere DATE between '%s' and '%s' and Shift_ID='%s'and Stack_holder_ID='%d'" ("string"), w623, w622, w616, 5 ("input 4")) -> (resulting string=w619:string)  [unwired: 2 in, 1 out]
              n143 = call "Execute query.vi"("String"=w619, "connection reference"=w621) -> ("Table"=w618:string[][], "connection reference 2"=w617:T1)  [unwired: 6 in, 2 out]
            }
            frame "2" {
              w638 = "%Y-%m-%d " ("time format string (%c)")
              n144 = Format Date/Time String(time format string (%c)=w638, seconds (now)=w637) -> (date/time string=w634:string)  [unwired: 1 in]
              n145 = Format Date/Time String(time format string (%c)=w638, seconds (now)=w636) -> (date/time string=w635:string)  [unwired: 1 in]
              n146 = Format Into String(format string="Select DATE,Production_Count,Station_ID,Stack_holder_ID\nfrom Production_COUNT\nWhere DATE between '%s' and '%s' and Shift_ID='%s'and Stack_holder_ID='%d'" ("string"), w635, w634, w628, 5 ("input 4")) -> (resulting string=w631:string)  [unwired: 2 in, 1 out]
              n147 = call "Execute query.vi"("String"=w631, "connection reference"=w633) -> ("Table"=w630:string[][], "connection reference 2"=w629:T1)  [unwired: 6 in, 2 out]
            }
            frame "3" {
              w650 = "%Y-%m-%d " ("time format string (%c)")
              n148 = Format Date/Time String(time format string (%c)=w650, seconds (now)=w649) -> (date/time string=w646:string)  [unwired: 1 in]
              n149 = Format Date/Time String(time format string (%c)=w650, seconds (now)=w648) -> (date/time string=w647:string)  [unwired: 1 in]
              n150 = Format Into String(format string="Select DATE,Production_Count,Station_ID,Stack_holder_ID\nfrom Production_COUNT\nWhere DATE between '%s' and '%s' and Shift_ID='%s'and Stack_holder_ID='%d'" ("string"), w647, w646, w640, 5 ("input 4")) -> (resulting string=w643:string)  [unwired: 2 in, 1 out]
              n151 = call "Execute query.vi"("String"=w643, "connection reference"=w645) -> ("Table"=w642:string[][], "connection reference 2"=w641:T1)  [unwired: 6 in, 2 out]
            }
          }
        }
      }
    }
    frame "ST 1" {
      n152 = case shown="\"ALL\", Default" w657 {
        tunnel: w663 -> [w675 w840 w899 w955 w1014 w1073]
        tunnel: w662 -> [w674 w839 w898 w954 w1013 w1072]
        tunnel: w661 -> [w673 w838 w897 w953 w1012 w1071]
        tunnel: w660 -> [w672 w837 w896 w952 w1011 w1070]
        tunnel: [w671 w836 w895 w951 w1010 w1069] -> w654
        tunnel: w659 -> [w670 w835 w894 w950 w1009 w1068]
        tunnel: [w669 w834 w893 w949 w1008 w1067] -> w658
        tunnel: w656 -> [w668 _ _ _ _ _]
        tunnel: w655 -> [w667 _ _ _ _ _]
        tunnel: w653 -> [w666 _ _ _ _ _]
        tunnel: w652 -> [w665 _ _ _ _ _]
        tunnel: [w664 _ _ _ _ _] -> w651
        frame "ALL", Default {
          n153 = case shown="\"3\"" w675 {
            selector: w675 -> [_ w714 w754 w794]
            tunnel: w674 -> [_ _ _ _]
            tunnel: w673 -> [_ _ _ _]
            tunnel: w672 -> [_ _ _ _]
            tunnel: [w678 w717 w757 w797] -> w671
            tunnel: w670 -> [w684 w723 w763 w803]
            tunnel: [w683 w722 w762 w802] -> w669
            tunnel: w668 -> [w682 w721 w761 w801]
            tunnel: w667 -> [w681 w720 w760 w800]
            tunnel: w666 -> [w679 w718 w758 w798]
            tunnel: w665 -> [w677 w716 w756 w796]
            tunnel: [w676 w715 w755 w795] -> w664
            frame "ALL", Default {
              n154 = for {
                tunnel: w682 -> [w696]
                tunnel: w681 -> [w695]
                shift-right: [w698] -> w683
                shift-left: w684 -> [w700]
                shift-right: [w687] -> w678
                shift-left: string[][] [] -> [w689]
                tunnel: w679 -> [w690] mode=indexing
                tunnel: w677 -> [w686]
                tunnel: [w685] -> w676
                n155 = case shown="\"April\"" w695 {
                  tunnel: ["1" "1" "2" "3" "4" "5" "6" "7" "8" "9" "10" "11" "12"] -> w694
                  frame "False", Default {
                  }
                  frame "January" {
                  }
                  frame "February" {
                  }
                  frame "March" {
                  }
                  frame "April" {
                  }
                  frame "May" {
                  }
                  frame "June" {
                  }
                  frame "July" {
                  }
                  frame "August" {
                  }
                  frame "September" {
                  }
                  frame "October" {
                  }
                  frame "November" {
                  }
                  frame "December" {
                  }
                }
                n156 = Concatenate Strings("Select DISTINCT PLAN_DATE,PRODUCTION_COUNT,STATION_ID,DATE\nfrom ", w690, " Where year( PLAN_DATE) ='%s' and month(PLAN_DATE) = '%s' and STATION_ID='%d'") -> (w691:string)
                n157 = Format Into String(format string=w691, w696, w694, 1 ("input 3")) -> (resulting string=w699:string)  [unwired: 2 in, 1 out]
                n158 = call "Execute query.vi"("error in (no error)"=w686, "String"=w699, "connection reference"=w700) -> ("error out"=w685:errorcluster, "Table"=w688:string[][], "connection reference 2"=w698:T1)  [unwired: 5 in, 1 out]
                n159 = Build Array (concatenate)(w689, w688) -> (w687:string[][])
              }
            }
            frame "1" {
              n160 = for {
                tunnel: w721 -> [w736]
                tunnel: w720 -> [w735]
                shift-right: [w738] -> w722
                shift-left: w723 -> [w740]
                shift-right: [w727] -> w717
                shift-left: string[][] [] -> [w729]
                tunnel: w718 -> [w730] mode=indexing
                tunnel: w716 -> [w726]
                tunnel: [w725] -> w715
                tunnel: w714 -> [w724]
                n161 = case shown="\"April\"" w735 {
                  tunnel: ["1" "1" "2" "3" "4" "5" "6" "7" "8" "9" "10" "11" "12"] -> w734
                  frame "False", Default {
                  }
                  frame "January" {
                  }
                  frame "February" {
                  }
                  frame "March" {
                  }
                  frame "April" {
                  }
                  frame "May" {
                  }
                  frame "June" {
                  }
                  frame "July" {
                  }
                  frame "August" {
                  }
                  frame "September" {
                  }
                  frame "October" {
                  }
                  frame "November" {
                  }
                  frame "December" {
                  }
                }
                n162 = Concatenate Strings("Select  DISTINCT PLAN_DATE,PRODUCTION_COUNT,STATION_ID,DATE\nfrom ", w730, " Where year( PLAN_DATE) ='%s' and month(PLAN_DATE) = '%s' and STATION_ID='%d' and SHIFT='%s'") -> (w731:string)
                n163 = Format Into String(format string=w731, w736, w734, 1 ("input 3"), w724) -> (resulting string=w739:string)  [unwired: 2 in, 1 out]
                n164 = call "Execute query.vi"("error in (no error)"=w726, "String"=w739, "connection reference"=w740) -> ("error out"=w725:errorcluster, "Table"=w728:string[][], "connection reference 2"=w738:T1)  [unwired: 5 in, 1 out]
                n165 = Build Array (concatenate)(w729, w728) -> (w727:string[][])
              }
            }
            frame "2" {
              n166 = for {
                tunnel: w761 -> [w776]
                tunnel: w760 -> [w775]
                shift-right: [w778] -> w762
                shift-left: w763 -> [w780]
                shift-right: [w767] -> w757
                shift-left: string[][] [] -> [w769]
                tunnel: w758 -> [w770] mode=indexing
                tunnel: w756 -> [w766]
                tunnel: [w765] -> w755
                tunnel: w754 -> [w764]
                n167 = case shown="\"April\"" w775 {
                  tunnel: ["1" "1" "2" "3" "4" "5" "6" "7" "8" "9" "10" "11" "12"] -> w774
                  frame "False", Default {
                  }
                  frame "January" {
                  }
                  frame "February" {
                  }
                  frame "March" {
                  }
                  frame "April" {
                  }
                  frame "May" {
                  }
                  frame "June" {
                  }
                  frame "July" {
                  }
                  frame "August" {
                  }
                  frame "September" {
                  }
                  frame "October" {
                  }
                  frame "November" {
                  }
                  frame "December" {
                  }
                }
                n168 = Concatenate Strings("Select DISTINCT PLAN_DATE,PRODUCTION_COUNT,STATION_ID,DATE\nfrom ", w770, " Where year( PLAN_DATE) ='%s' and month(PLAN_DATE) = '%s' and STATION_ID='%d' and SHIFT='%s'") -> (w771:string)
                n169 = Format Into String(format string=w771, w776, w774, 1 ("input 3"), w764) -> (resulting string=w779:string)  [unwired: 2 in, 1 out]
                n170 = call "Execute query.vi"("error in (no error)"=w766, "String"=w779, "connection reference"=w780) -> ("error out"=w765:errorcluster, "Table"=w768:string[][], "connection reference 2"=w778:T1)  [unwired: 5 in, 1 out]
                n171 = Build Array (concatenate)(w769, w768) -> (w767:string[][])
              }
            }
            frame "3" {
              n172 = for {
                tunnel: w801 -> [w816]
                tunnel: w800 -> [w815]
                shift-right: [w818] -> w802
                shift-left: w803 -> [w820]
                shift-right: [w807] -> w797
                shift-left: string[][] [] -> [w809]
                tunnel: w798 -> [w810] mode=indexing
                tunnel: w796 -> [w806]
                tunnel: [w805] -> w795
                tunnel: w794 -> [w804]
                n173 = case shown="\"April\"" w815 {
                  tunnel: ["1" "1" "2" "3" "4" "5" "6" "7" "8" "9" "10" "11" "12"] -> w814
                  frame "False", Default {
                  }
                  frame "January" {
                  }
                  frame "February" {
                  }
                  frame "March" {
                  }
                  frame "April" {
                  }
                  frame "May" {
                  }
                  frame "June" {
                  }
                  frame "July" {
                  }
                  frame "August" {
                  }
                  frame "September" {
                  }
                  frame "October" {
                  }
                  frame "November" {
                  }
                  frame "December" {
                  }
                }
                n174 = Concatenate Strings("Select DISTINCT PLAN_DATE,PRODUCTION_COUNT,STATION_ID,DATE\nfrom ", w810, " Where year( PLAN_DATE) ='%s' and month(PLAN_DATE) = '%s' and STATION_ID='%d' and SHIFT='%s'") -> (w811:string)
                n175 = Format Into String(format string=w811, w816, w814, 1 ("input 3"), w804) -> (resulting string=w819:string)  [unwired: 2 in, 1 out]
                n176 = call "Execute query.vi"("error in (no error)"=w806, "String"=w819, "connection reference"=w820) -> ("error out"=w805:errorcluster, "Table"=w808:string[][], "connection reference 2"=w818:T1)  [unwired: 5 in, 1 out]
                n177 = Build Array (concatenate)(w809, w808) -> (w807:string[][])
              }
            }
          }
        }
        frame "Logistics" {
          n178 = case shown="\"ALL\"" w840 {
            selector: w840 -> [_ _ w856 w869 w882]
            tunnel: w839 -> [_ w852 w865 w878 w891]
            tunnel: w838 -> [_ w851 w864 w877 w890]
            tunnel: w837 -> [_ _ _ _ _]
            tunnel: [_ w845 w858 w871 w884] -> w836
            tunnel: w835 -> [w841 w848 w861 w874 w887]
            tunnel: [w841 w844 w857 w870 w883] -> w834
            frame "False", Default {
            }
            frame "ALL" {
              w853 = "%Y-%m-%d " ("time format string (%c)")
              n179 = Format Date/Time String(time format string (%c)=w853, seconds (now)=w851) -> (date/time string=w850:string)  [unwired: 1 in]
              n180 = Format Date/Time String(time format string (%c)=w853, seconds (now)=w852) -> (date/time string=w849:string)  [unwired: 1 in]
              n181 = Format Into String(format string="Select DATE,Production_Count,Station_ID,Stack_holder_ID\nfrom Production_COUNT\nWhere DATE between '%s' and '%s' and Stack_holder_ID='%d'\nand Station_ID='%d'" ("string"), w850, w849, 2 ("input 3"), 1 ("input 4")) -> (resulting string=w846:string)  [unwired: 2 in, 1 out]
              n182 = call "Execute query.vi"("String"=w846, "connection reference"=w848) -> ("Table"=w845:string[][], "connection reference 2"=w844:T1)  [unwired: 6 in, 2 out]
            }
            frame "1" {
              w866 = "%Y-%m-%d " ("time format string (%c)")
              n183 = Format Date/Time String(time format string (%c)=w866, seconds (now)=w865) -> (date/time string=w862:string)  [unwired: 1 in]
              n184 = Format Date/Time String(time format string (%c)=w866, seconds (now)=w864) -> (date/time string=w863:string)  [unwired: 1 in]
              n185 = Format Into String(format string="Select DATE,Production_Count,Station_ID,Stack_holder_ID\nfrom Production_COUNT\nWhere DATE between '%s' and '%s' and Shift_ID='%s'and Stack_holder_ID='%d'\nand Station_ID='%d'" ("string"), w863, w862, w856, 2 ("input 4"), 1 ("input 4")) -> (resulting string=w859:string)  [unwired: 2 in, 1 out]
              n186 = call "Execute query.vi"("String"=w859, "connection reference"=w861) -> ("Table"=w858:string[][], "connection reference 2"=w857:T1)  [unwired: 6 in, 2 out]
            }
            frame "2" {
              w879 = "%Y-%m-%d " ("time format string (%c)")
              n187 = Format Date/Time String(time format string (%c)=w879, seconds (now)=w878) -> (date/time string=w875:string)  [unwired: 1 in]
              n188 = Format Date/Time String(time format string (%c)=w879, seconds (now)=w877) -> (date/time string=w876:string)  [unwired: 1 in]
              n189 = Format Into String(format string="Select DATE,Production_Count,Station_ID,Stack_holder_ID\nfrom Production_COUNT\nWhere DATE between '%s' and '%s' and Shift_ID='%s'and Stack_holder_ID='%d'\nand Station_ID='%d'" ("string"), w876, w875, w869, 2 ("input 4"), 1 ("input 4")) -> (resulting string=w872:string)  [unwired: 2 in, 1 out]
              n190 = call "Execute query.vi"("String"=w872, "connection reference"=w874) -> ("Table"=w871:string[][], "connection reference 2"=w870:T1)  [unwired: 6 in, 2 out]
            }
            frame "3" {
              w892 = "%Y-%m-%d " ("time format string (%c)")
              n191 = Format Date/Time String(time format string (%c)=w892, seconds (now)=w891) -> (date/time string=w888:string)  [unwired: 1 in]
              n192 = Format Date/Time String(time format string (%c)=w892, seconds (now)=w890) -> (date/time string=w889:string)  [unwired: 1 in]
              n193 = Format Into String(format string="Select DATE,Production_Count,Station_ID,Stack_holder_ID\nfrom Production_COUNT\nWhere DATE between '%s' and '%s' and Shift_ID='%s'and Stack_holder_ID='%d'\nand Station_ID='%d'" ("string"), w889, w888, w882, 2 ("input 4"), 1 ("input 4")) -> (resulting string=w885:string)  [unwired: 2 in, 1 out]
              n194 = call "Execute query.vi"("String"=w885, "connection reference"=w887) -> ("Table"=w884:string[][], "connection reference 2"=w883:T1)  [unwired: 6 in, 2 out]
            }
          }
        }
        frame "Gap Leader" {
          n195 = case shown="\"3\"" w899 {
            selector: w899 -> [_ _ w914 w926 w938]
            tunnel: w898 -> [_ w911 w923 w935 w947]
            tunnel: w897 -> [_ w910 w922 w934 w946]
            tunnel: w896 -> [_ _ _ _ _]
            tunnel: [_ w904 w916 w928 w940] -> w895
            tunnel: w894 -> [w900 w907 w919 w931 w943]
            tunnel: [w900 w903 w915 w927 w939] -> w893
            frame "False", Default {
            }
            frame "ALL" {
              w912 = "%Y-%m-%d " ("time format string (%c)")
              n196 = Format Date/Time String(time format string (%c)=w912, seconds (now)=w910) -> (date/time string=w909:string)  [unwired: 1 in]
              n197 = Format Date/Time String(time format string (%c)=w912, seconds (now)=w911) -> (date/time string=w908:string)  [unwired: 1 in]
              n198 = Format Into String(format string="Select DATE,Production_Count,Station_ID,Stack_holder_ID\nfrom Production_COUNT\nWhere DATE between '%s' and '%s' and Stack_holder_ID='%d'\nand Station_ID='%d'" ("string"), w909, w908, 1 ("input 3"), 1 ("input 3")) -> (resulting string=w905:string)  [unwired: 2 in, 1 out]
              n199 = call "Execute query.vi"("String"=w905, "connection reference"=w907) -> ("Table"=w904:string[][], "connection reference 2"=w903:T1)  [unwired: 6 in, 2 out]
            }
            frame "1" {
              w913 = 1 ("input 4")
              w924 = "%Y-%m-%d " ("time format string (%c)")
              n200 = Format Date/Time String(time format string (%c)=w924, seconds (now)=w923) -> (date/time string=w920:string)  [unwired: 1 in]
              n201 = Format Date/Time String(time format string (%c)=w924, seconds (now)=w922) -> (date/time string=w921:string)  [unwired: 1 in]
              n202 = Format Into String(format string="Select DATE,Production_Count,Station_ID,Stack_holder_ID\nfrom Production_COUNT\nWhere DATE between '%s' and '%s' and Shift_ID='%s'and Stack_holder_ID='%d'\nand Station_ID='%d'" ("string"), w921, w920, w914, w913, w913) -> (resulting string=w917:string)  [unwired: 2 in, 1 out]
              n203 = call "Execute query.vi"("String"=w917, "connection reference"=w919) -> ("Table"=w916:string[][], "connection reference 2"=w915:T1)  [unwired: 6 in, 2 out]
            }
            frame "2" {
              w925 = 1 ("input 4")
              w936 = "%Y-%m-%d " ("time format string (%c)")
              n204 = Format Date/Time String(time format string (%c)=w936, seconds (now)=w935) -> (date/time string=w932:string)  [unwired: 1 in]
              n205 = Format Date/Time String(time format string (%c)=w936, seconds (now)=w934) -> (date/time string=w933:string)  [unwired: 1 in]
              n206 = Format Into String(format string="Select DATE,Production_Count,Station_ID,Stack_holder_ID\nfrom Production_COUNT\nWhere DATE between '%s' and '%s' and Shift_ID='%s'and Stack_holder_ID='%d'\nand Station_ID='%d'" ("string"), w933, w932, w926, w925, w925) -> (resulting string=w929:string)  [unwired: 2 in, 1 out]
              n207 = call "Execute query.vi"("String"=w929, "connection reference"=w931) -> ("Table"=w928:string[][], "connection reference 2"=w927:T1)  [unwired: 6 in, 2 out]
            }
            frame "3" {
              w937 = 1 ("input 4")
              w948 = "%Y-%m-%d " ("time format string (%c)")
              n208 = Format Date/Time String(time format string (%c)=w948, seconds (now)=w947) -> (date/time string=w944:string)  [unwired: 1 in]
              n209 = Format Date/Time String(time format string (%c)=w948, seconds (now)=w946) -> (date/time string=w945:string)  [unwired: 1 in]
              n210 = Format Into String(format string="Select DATE,Production_Count,Station_ID,Stack_holder_ID\nfrom Production_COUNT\nWhere DATE between '%s' and '%s' and Shift_ID='%s'and Stack_holder_ID='%d'\nand Station_ID='%d'" ("string"), w945, w944, w938, w937, w937) -> (resulting string=w941:string)  [unwired: 2 in, 1 out]
              n211 = call "Execute query.vi"("String"=w941, "connection reference"=w943) -> ("Table"=w940:string[][], "connection reference 2"=w939:T1)  [unwired: 6 in, 2 out]
            }
          }
        }
        frame "Maintenance" {
          n212 = case shown="\"ALL\"" w955 {
            selector: w955 -> [_ _ w971 w984 w997]
            tunnel: w954 -> [_ w967 w980 w993 w1006]
            tunnel: w953 -> [_ w966 w979 w992 w1005]
            tunnel: w952 -> [_ _ _ _ _]
            tunnel: [_ w960 w973 w986 w999] -> w951
            tunnel: w950 -> [w956 w963 w976 w989 w1002]
            tunnel: [w956 w959 w972 w985 w998] -> w949
            frame "False", Default {
            }
            frame "ALL" {
              w968 = "%Y-%m-%d " ("time format string (%c)")
              n213 = Format Date/Time String(time format string (%c)=w968, seconds (now)=w966) -> (date/time string=w965:string)  [unwired: 1 in]
              n214 = Format Date/Time String(time format string (%c)=w968, seconds (now)=w967) -> (date/time string=w964:string)  [unwired: 1 in]
              n215 = Format Into String(format string="Select DATE,Production_Count,Station_ID,Stack_holder_ID\nfrom Production_COUNT\nWhere DATE between '%s' and '%s' and Stack_holder_ID='%d'\nand Station_ID='%d'" ("string"), w965, w964, 3 ("input 3"), 1 ("input 4")) -> (resulting string=w961:string)  [unwired: 2 in, 1 out]
              n216 = call "Execute query.vi"("String"=w961, "connection reference"=w963) -> ("Table"=w960:string[][], "connection reference 2"=w959:T1)  [unwired: 6 in, 2 out]
            }
            frame "1" {
              w981 = "%Y-%m-%d " ("time format string (%c)")
              n217 = Format Date/Time String(time format string (%c)=w981, seconds (now)=w980) -> (date/time string=w977:string)  [unwired: 1 in]
              n218 = Format Date/Time String(time format string (%c)=w981, seconds (now)=w979) -> (date/time string=w978:string)  [unwired: 1 in]
              n219 = Format Into String(format string="Select DATE,Production_Count,Station_ID,Stack_holder_ID\nfrom Production_COUNT\nWhere DATE between '%s' and '%s' and Shift_ID='%s'and Stack_holder_ID='%d'\nand Station_ID='%d'" ("string"), w978, w977, w971, 3 ("input 4"), 1 ("input 5")) -> (resulting string=w974:string)  [unwired: 2 in, 1 out]
              n220 = call "Execute query.vi"("String"=w974, "connection reference"=w976) -> ("Table"=w973:string[][], "connection reference 2"=w972:T1)  [unwired: 6 in, 2 out]
            }
            frame "2" {
              w994 = "%Y-%m-%d " ("time format string (%c)")
              n221 = Format Date/Time String(time format string (%c)=w994, seconds (now)=w993) -> (date/time string=w990:string)  [unwired: 1 in]
              n222 = Format Date/Time String(time format string (%c)=w994, seconds (now)=w992) -> (date/time string=w991:string)  [unwired: 1 in]
              n223 = Format Into String(format string="Select DATE,Production_Count,Station_ID,Stack_holder_ID\nfrom Production_COUNT\nWhere DATE between '%s' and '%s' and Shift_ID='%s'and Stack_holder_ID='%d'\nand Station_ID='%d'" ("string"), w991, w990, w984, 3 ("input 4"), 1 ("input 5")) -> (resulting string=w987:string)  [unwired: 2 in, 1 out]
              n224 = call "Execute query.vi"("String"=w987, "connection reference"=w989) -> ("Table"=w986:string[][], "connection reference 2"=w985:T1)  [unwired: 6 in, 2 out]
            }
            frame "3" {
              w1007 = "%Y-%m-%d " ("time format string (%c)")
              n225 = Format Date/Time String(time format string (%c)=w1007, seconds (now)=w1006) -> (date/time string=w1003:string)  [unwired: 1 in]
              n226 = Format Date/Time String(time format string (%c)=w1007, seconds (now)=w1005) -> (date/time string=w1004:string)  [unwired: 1 in]
              n227 = Format Into String(format string="Select DATE,Production_Count,Station_ID,Stack_holder_ID\nfrom Production_COUNT\nWhere DATE between '%s' and '%s' and Shift_ID='%s'and Stack_holder_ID='%d'\nand Station_ID='%d'" ("string"), w1004, w1003, w997, 3 ("input 4"), 1 ("input 5")) -> (resulting string=w1000:string)  [unwired: 2 in, 1 out]
              n228 = call "Execute query.vi"("String"=w1000, "connection reference"=w1002) -> ("Table"=w999:string[][], "connection reference 2"=w998:T1)  [unwired: 6 in, 2 out]
            }
          }
        }
        frame "Quality" {
          n229 = case shown="\"ALL\"" w1014 {
            selector: w1014 -> [_ _ w1030 w1043 w1056]
            tunnel: w1013 -> [_ w1026 w1039 w1052 w1065]
            tunnel: w1012 -> [_ w1025 w1038 w1051 w1064]
            tunnel: w1011 -> [_ _ _ _ _]
            tunnel: [_ w1019 w1032 w1045 w1058] -> w1010
            tunnel: w1009 -> [w1015 w1022 w1035 w1048 w1061]
            tunnel: [w1015 w1018 w1031 w1044 w1057] -> w1008
            frame "False", Default {
            }
            frame "ALL" {
              w1027 = "%Y-%m-%d " ("time format string (%c)")
              n230 = Format Date/Time String(time format string (%c)=w1027, seconds (now)=w1025) -> (date/time string=w1024:string)  [unwired: 1 in]
              n231 = Format Date/Time String(time format string (%c)=w1027, seconds (now)=w1026) -> (date/time string=w1023:string)  [unwired: 1 in]
              n232 = Format Into String(format string="Select DATE,Production_Count,Station_ID,Stack_holder_ID\nfrom Production_COUNT\nWhere DATE between '%s' and '%s' and Stack_holder_ID='%d'\nand Station_ID='%d'" ("string"), w1024, w1023, 4 ("input 3"), 1 ("input 3")) -> (resulting string=w1020:string)  [unwired: 2 in, 1 out]
              n233 = call "Execute query.vi"("String"=w1020, "connection reference"=w1022) -> ("Table"=w1019:string[][], "connection reference 2"=w1018:T1)  [unwired: 6 in, 2 out]
            }
            frame "1" {
              w1040 = "%Y-%m-%d " ("time format string (%c)")
              n234 = Format Date/Time String(time format string (%c)=w1040, seconds (now)=w1039) -> (date/time string=w1036:string)  [unwired: 1 in]
              n235 = Format Date/Time String(time format string (%c)=w1040, seconds (now)=w1038) -> (date/time string=w1037:string)  [unwired: 1 in]
              n236 = Format Into String(format string="Select DATE,Production_Count,Station_ID,Stack_holder_ID\nfrom Production_COUNT\nWhere DATE between '%s' and '%s' and Shift_ID='%s'and Stack_holder_ID='%d'\nand Station_ID='%d'" ("string"), w1037, w1036, w1030, 4 ("input 4"), 1 ("input 4")) -> (resulting string=w1033:string)  [unwired: 2 in, 1 out]
              n237 = call "Execute query.vi"("String"=w1033, "connection reference"=w1035) -> ("Table"=w1032:string[][], "connection reference 2"=w1031:T1)  [unwired: 6 in, 2 out]
            }
            frame "2" {
              w1053 = "%Y-%m-%d " ("time format string (%c)")
              n238 = Format Date/Time String(time format string (%c)=w1053, seconds (now)=w1052) -> (date/time string=w1049:string)  [unwired: 1 in]
              n239 = Format Date/Time String(time format string (%c)=w1053, seconds (now)=w1051) -> (date/time string=w1050:string)  [unwired: 1 in]
              n240 = Format Into String(format string="Select DATE,Production_Count,Station_ID,Stack_holder_ID\nfrom Production_COUNT\nWhere DATE between '%s' and '%s' and Shift_ID='%s'and Stack_holder_ID='%d'\nand Station_ID='%d'" ("string"), w1050, w1049, w1043, 4 ("input 4"), 1 ("input 4")) -> (resulting string=w1046:string)  [unwired: 2 in, 1 out]
              n241 = call "Execute query.vi"("String"=w1046, "connection reference"=w1048) -> ("Table"=w1045:string[][], "connection reference 2"=w1044:T1)  [unwired: 6 in, 2 out]
            }
            frame "3" {
              w1066 = "%Y-%m-%d " ("time format string (%c)")
              n242 = Format Date/Time String(time format string (%c)=w1066, seconds (now)=w1065) -> (date/time string=w1062:string)  [unwired: 1 in]
              n243 = Format Date/Time String(time format string (%c)=w1066, seconds (now)=w1064) -> (date/time string=w1063:string)  [unwired: 1 in]
              n244 = Format Into String(format string="Select DATE,Production_Count,Station_ID,Stack_holder_ID\nfrom Production_COUNT\nWhere DATE between '%s' and '%s' and Shift_ID='%s'and Stack_holder_ID='%d'\nand Station_ID='%d'" ("string"), w1063, w1062, w1056, 4 ("input 4"), 1 ("input 4")) -> (resulting string=w1059:string)  [unwired: 2 in, 1 out]
              n245 = call "Execute query.vi"("String"=w1059, "connection reference"=w1061) -> ("Table"=w1058:string[][], "connection reference 2"=w1057:T1)  [unwired: 6 in, 2 out]
            }
          }
        }
        frame "Production" {
          n246 = case shown="\"False\", Default" w1073 {
            selector: w1073 -> [_ _ w1089 w1102 w1115]
            tunnel: w1072 -> [_ w1085 w1098 w1111 w1124]
            tunnel: w1071 -> [_ w1084 w1097 w1110 w1123]
            tunnel: w1070 -> [_ _ _ _ _]
            tunnel: [_ w1078 w1091 w1104 w1117] -> w1069
            tunnel: w1068 -> [w1074 w1081 w1094 w1107 w1120]
            tunnel: [w1074 w1077 w1090 w1103 w1116] -> w1067
            frame "False", Default {
            }
            frame "ALL" {
              w1086 = "%Y-%m-%d " ("time format string (%c)")
              n247 = Format Date/Time String(time format string (%c)=w1086, seconds (now)=w1084) -> (date/time string=w1083:string)  [unwired: 1 in]
              n248 = Format Date/Time String(time format string (%c)=w1086, seconds (now)=w1085) -> (date/time string=w1082:string)  [unwired: 1 in]
              n249 = Format Into String(format string="Select DATE,Production_Count,Station_ID,Stack_holder_ID\nfrom Production_COUNT\nWhere DATE between '%s' and '%s' and Stack_holder_ID='%d'\nand Station_ID='%d'" ("string"), w1083, w1082, 5 ("input 3"), 1 ("input 3")) -> (resulting string=w1079:string)  [unwired: 2 in, 1 out]
              n250 = call "Execute query.vi"("String"=w1079, "connection reference"=w1081) -> ("Table"=w1078:string[][], "connection reference 2"=w1077:T1)  [unwired: 6 in, 2 out]
            }
            frame "1" {
              w1099 = "%Y-%m-%d " ("time format string (%c)")
              n251 = Format Date/Time String(time format string (%c)=w1099, seconds (now)=w1098) -> (date/time string=w1095:string)  [unwired: 1 in]
              n252 = Format Date/Time String(time format string (%c)=w1099, seconds (now)=w1097) -> (date/time string=w1096:string)  [unwired: 1 in]
              n253 = Format Into String(format string="Select DATE,Production_Count,Station_ID,Stack_holder_ID\nfrom Production_COUNT\nWhere DATE between '%s' and '%s' and Shift_ID='%s'and Stack_holder_ID='%d'\nand Station_ID='%d'" ("string"), w1096, w1095, w1089, 5 ("input 4"), 1 ("input 4")) -> (resulting string=w1092:string)  [unwired: 2 in, 1 out]
              n254 = call "Execute query.vi"("String"=w1092, "connection reference"=w1094) -> ("Table"=w1091:string[][], "connection reference 2"=w1090:T1)  [unwired: 6 in, 2 out]
            }
            frame "2" {
              w1112 = "%Y-%m-%d " ("time format string (%c)")
              n255 = Format Date/Time String(time format string (%c)=w1112, seconds (now)=w1111) -> (date/time string=w1108:string)  [unwired: 1 in]
              n256 = Format Date/Time String(time format string (%c)=w1112, seconds (now)=w1110) -> (date/time string=w1109:string)  [unwired: 1 in]
              n257 = Format Into String(format string="Select DATE,Production_Count,Station_ID,Stack_holder_ID\nfrom Production_COUNT\nWhere DATE between '%s' and '%s' and Shift_ID='%s'and Stack_holder_ID='%d'\nand Station_ID='%d'" ("string"), w1109, w1108, w1102, 5 ("input 4"), 1 ("input 4")) -> (resulting string=w1105:string)  [unwired: 2 in, 1 out]
              n258 = call "Execute query.vi"("String"=w1105, "connection reference"=w1107) -> ("Table"=w1104:string[][], "connection reference 2"=w1103:T1)  [unwired: 6 in, 2 out]
            }
            frame "3" {
              w1125 = "%Y-%m-%d " ("time format string (%c)")
              n259 = Format Date/Time String(time format string (%c)=w1125, seconds (now)=w1124) -> (date/time string=w1121:string)  [unwired: 1 in]
              n260 = Format Date/Time String(time format string (%c)=w1125, seconds (now)=w1123) -> (date/time string=w1122:string)  [unwired: 1 in]
              n261 = Format Into String(format string="Select DATE,Production_Count,Station_ID,Stack_holder_ID\nfrom Production_COUNT\nWhere DATE between '%s' and '%s' and Shift_ID='%s'and Stack_holder_ID='%d'\nand Station_ID='%d'" ("string"), w1122, w1121, w1115, 5 ("input 4"), 1 ("input 4")) -> (resulting string=w1118:string)  [unwired: 2 in, 1 out]
              n262 = call "Execute query.vi"("String"=w1118, "connection reference"=w1120) -> ("Table"=w1117:string[][], "connection reference 2"=w1116:T1)  [unwired: 6 in, 2 out]
            }
          }
        }
      }
    }
    frame "ST 2" {
      n263 = case shown="\"ALL\", Default" w1132 {
        tunnel: w1138 -> [w1150 w1315 w1374 w1430 w1489 w1548]
        tunnel: w1137 -> [w1149 w1314 w1373 w1429 w1488 w1547]
        tunnel: w1136 -> [w1148 w1313 w1372 w1428 w1487 w1546]
        tunnel: w1135 -> [w1147 w1312 w1371 w1427 w1486 w1545]
        tunnel: [w1146 w1311 w1370 w1426 w1485 w1544] -> w1129
        tunnel: w1134 -> [w1145 w1310 w1369 w1425 w1484 w1543]
        tunnel: [w1144 w1309 w1368 w1424 w1483 w1542] -> w1133
        tunnel: w1131 -> [w1143 _ _ _ _ _]
        tunnel: w1130 -> [w1142 _ _ _ _ _]
        tunnel: w1128 -> [w1141 _ _ _ _ _]
        tunnel: w1127 -> [w1140 _ _ _ _ _]
        tunnel: [w1139 _ _ _ _ _] -> w1126
        frame "ALL", Default {
          n264 = case shown="\"3\"" w1150 {
            selector: w1150 -> [_ w1189 w1229 w1269]
            tunnel: w1149 -> [_ _ _ _]
            tunnel: w1148 -> [_ _ _ _]
            tunnel: w1147 -> [_ _ _ _]
            tunnel: [w1153 w1192 w1232 w1272] -> w1146
            tunnel: w1145 -> [w1159 w1198 w1238 w1278]
            tunnel: [w1158 w1197 w1237 w1277] -> w1144
            tunnel: w1143 -> [w1157 w1196 w1236 w1276]
            tunnel: w1142 -> [w1156 w1195 w1235 w1275]
            tunnel: w1141 -> [w1154 w1193 w1233 w1273]
            tunnel: w1140 -> [w1152 w1191 w1231 w1271]
            tunnel: [w1151 w1190 w1230 w1270] -> w1139
            frame "ALL", Default {
              n265 = for {
                tunnel: w1157 -> [w1171]
                tunnel: w1156 -> [w1170]
                shift-right: [w1173] -> w1158
                shift-left: w1159 -> [w1175]
                shift-right: [w1162] -> w1153
                shift-left: string[][] [] -> [w1164]
                tunnel: w1154 -> [w1165] mode=indexing
                tunnel: w1152 -> [w1161]
                tunnel: [w1160] -> w1151
                n266 = case shown="\"April\"" w1170 {
                  tunnel: ["1" "1" "2" "3" "4" "5" "6" "7" "8" "9" "10" "11" "12"] -> w1169
                  frame "False", Default {
                  }
                  frame "January" {
                  }
                  frame "February" {
                  }
                  frame "March" {
                  }
                  frame "April" {
                  }
                  frame "May" {
                  }
                  frame "June" {
                  }
                  frame "July" {
                  }
                  frame "August" {
                  }
                  frame "September" {
                  }
                  frame "October" {
                  }
                  frame "November" {
                  }
                  frame "December" {
                  }
                }
                n267 = Concatenate Strings("Select DISTINCT PLAN_DATE,PRODUCTION_COUNT,STATION_ID,DATE\nfrom ", w1165, " Where year( PLAN_DATE) ='%s' and month(PLAN_DATE) = '%s' and STATION_ID='%d'") -> (w1166:string)
                n268 = Format Into String(format string=w1166, w1171, w1169, 2 ("input 3")) -> (resulting string=w1174:string)  [unwired: 2 in, 1 out]
                n269 = call "Execute query.vi"("error in (no error)"=w1161, "String"=w1174, "connection reference"=w1175) -> ("error out"=w1160:errorcluster, "Table"=w1163:string[][], "connection reference 2"=w1173:T1)  [unwired: 5 in, 1 out]
                n270 = Build Array (concatenate)(w1164, w1163) -> (w1162:string[][])
              }
            }
            frame "1" {
              n271 = for {
                tunnel: w1196 -> [w1211]
                tunnel: w1195 -> [w1210]
                shift-right: [w1213] -> w1197
                shift-left: w1198 -> [w1215]
                shift-right: [w1202] -> w1192
                shift-left: string[][] [] -> [w1204]
                tunnel: w1193 -> [w1205] mode=indexing
                tunnel: w1191 -> [w1201]
                tunnel: [w1200] -> w1190
                tunnel: w1189 -> [w1199]
                n272 = case shown="\"April\"" w1210 {
                  tunnel: ["1" "1" "2" "3" "4" "5" "6" "7" "8" "9" "10" "11" "12"] -> w1209
                  frame "False", Default {
                  }
                  frame "January" {
                  }
                  frame "February" {
                  }
                  frame "March" {
                  }
                  frame "April" {
                  }
                  frame "May" {
                  }
                  frame "June" {
                  }
                  frame "July" {
                  }
                  frame "August" {
                  }
                  frame "September" {
                  }
                  frame "October" {
                  }
                  frame "November" {
                  }
                  frame "December" {
                  }
                }
                n273 = Concatenate Strings("Select DISTINCT PLAN_DATE,PRODUCTION_COUNT,STATION_ID,DATE\nfrom ", w1205, " Where year( PLAN_DATE) ='%s' and month(PLAN_DATE) = '%s' and STATION_ID='%d' and SHIFT='%s'") -> (w1206:string)
                n274 = Format Into String(format string=w1206, w1211, w1209, 2 ("input 3"), w1199) -> (resulting string=w1214:string)  [unwired: 2 in, 1 out]
                n275 = call "Execute query.vi"("error in (no error)"=w1201, "String"=w1214, "connection reference"=w1215) -> ("error out"=w1200:errorcluster, "Table"=w1203:string[][], "connection reference 2"=w1213:T1)  [unwired: 5 in, 1 out]
                n276 = Build Array (concatenate)(w1204, w1203) -> (w1202:string[][])
              }
            }
            frame "2" {
              n277 = for {
                tunnel: w1236 -> [w1251]
                tunnel: w1235 -> [w1250]
                shift-right: [w1253] -> w1237
                shift-left: w1238 -> [w1255]
                shift-right: [w1242] -> w1232
                shift-left: string[][] [] -> [w1244]
                tunnel: w1233 -> [w1245] mode=indexing
                tunnel: w1231 -> [w1241]
                tunnel: [w1240] -> w1230
                tunnel: w1229 -> [w1239]
                n278 = case shown="\"April\"" w1250 {
                  tunnel: ["1" "1" "2" "3" "4" "5" "6" "7" "8" "9" "10" "11" "12"] -> w1249
                  frame "False", Default {
                  }
                  frame "January" {
                  }
                  frame "February" {
                  }
                  frame "March" {
                  }
                  frame "April" {
                  }
                  frame "May" {
                  }
                  frame "June" {
                  }
                  frame "July" {
                  }
                  frame "August" {
                  }
                  frame "September" {
                  }
                  frame "October" {
                  }
                  frame "November" {
                  }
                  frame "December" {
                  }
                }
                n279 = Concatenate Strings("Select DISTINCT PLAN_DATE,PRODUCTION_COUNT,STATION_ID,DATE\nfrom ", w1245, " Where year( PLAN_DATE) ='%s' and month(PLAN_DATE) = '%s' and STATION_ID='%d' and SHIFT='%s'") -> (w1246:string)
                n280 = Format Into String(format string=w1246, w1251, w1249, 2 ("input 3"), w1239) -> (resulting string=w1254:string)  [unwired: 2 in, 1 out]
                n281 = call "Execute query.vi"("error in (no error)"=w1241, "String"=w1254, "connection reference"=w1255) -> ("error out"=w1240:errorcluster, "Table"=w1243:string[][], "connection reference 2"=w1253:T1)  [unwired: 5 in, 1 out]
                n282 = Build Array (concatenate)(w1244, w1243) -> (w1242:string[][])
              }
            }
            frame "3" {
              n283 = for {
                tunnel: w1276 -> [w1291]
                tunnel: w1275 -> [w1290]
                shift-right: [w1293] -> w1277
                shift-left: w1278 -> [w1295]
                shift-right: [w1282] -> w1272
                shift-left: string[][] [] -> [w1284]
                tunnel: w1273 -> [w1285] mode=indexing
                tunnel: w1271 -> [w1281]
                tunnel: [w1280] -> w1270
                tunnel: w1269 -> [w1279]
                n284 = case shown="\"April\"" w1290 {
                  tunnel: ["1" "1" "2" "3" "4" "5" "6" "7" "8" "9" "10" "11" "12"] -> w1289
                  frame "False", Default {
                  }
                  frame "January" {
                  }
                  frame "February" {
                  }
                  frame "March" {
                  }
                  frame "April" {
                  }
                  frame "May" {
                  }
                  frame "June" {
                  }
                  frame "July" {
                  }
                  frame "August" {
                  }
                  frame "September" {
                  }
                  frame "October" {
                  }
                  frame "November" {
                  }
                  frame "December" {
                  }
                }
                n285 = Concatenate Strings("Select DISTINCT PLAN_DATE,PRODUCTION_COUNT,STATION_ID,DATE\nfrom ", w1285, " Where year( PLAN_DATE) ='%s' and month(PLAN_DATE) = '%s' and STATION_ID='%d' and SHIFT='%s'") -> (w1286:string)
                n286 = Format Into String(format string=w1286, w1291, w1289, 2 ("input 3"), w1279) -> (resulting string=w1294:string)  [unwired: 2 in, 1 out]
                n287 = call "Execute query.vi"("error in (no error)"=w1281, "String"=w1294, "connection reference"=w1295) -> ("error out"=w1280:errorcluster, "Table"=w1283:string[][], "connection reference 2"=w1293:T1)  [unwired: 5 in, 1 out]
                n288 = Build Array (concatenate)(w1284, w1283) -> (w1282:string[][])
              }
            }
          }
        }
        frame "Logistics" {
          n289 = case shown="\"ALL\"" w1315 {
            selector: w1315 -> [_ _ w1331 w1344 w1357]
            tunnel: w1314 -> [_ w1327 w1340 w1353 w1366]
            tunnel: w1313 -> [_ w1326 w1339 w1352 w1365]
            tunnel: w1312 -> [_ _ _ _ _]
            tunnel: [_ w1320 w1333 w1346 w1359] -> w1311
            tunnel: w1310 -> [w1316 w1323 w1336 w1349 w1362]
            tunnel: [w1316 w1319 w1332 w1345 w1358] -> w1309
            frame "False", Default {
            }
            frame "ALL" {
              w1328 = "%Y-%m-%d " ("time format string (%c)")
              n290 = Format Date/Time String(time format string (%c)=w1328, seconds (now)=w1326) -> (date/time string=w1325:string)  [unwired: 1 in]
              n291 = Format Date/Time String(time format string (%c)=w1328, seconds (now)=w1327) -> (date/time string=w1324:string)  [unwired: 1 in]
              n292 = Format Into String(format string="Select DATE,Production_Count,Station_ID,Stack_holder_ID\nfrom Production_COUNT\nWhere DATE between '%s' and '%s' and Stack_holder_ID='%d'\nand Station_ID='%d'" ("string"), w1325, w1324, 2 ("input 3"), 1 ("input 4")) -> (resulting string=w1321:string)  [unwired: 2 in, 1 out]
              n293 = call "Execute query.vi"("String"=w1321, "connection reference"=w1323) -> ("Table"=w1320:string[][], "connection reference 2"=w1319:T1)  [unwired: 6 in, 2 out]
            }
            frame "1" {
              w1341 = "%Y-%m-%d " ("time format string (%c)")
              n294 = Format Date/Time String(time format string (%c)=w1341, seconds (now)=w1340) -> (date/time string=w1337:string)  [unwired: 1 in]
              n295 = Format Date/Time String(time format string (%c)=w1341, seconds (now)=w1339) -> (date/time string=w1338:string)  [unwired: 1 in]
              n296 = Format Into String(format string="Select DATE,Production_Count,Station_ID,Stack_holder_ID\nfrom Production_COUNT\nWhere DATE between '%s' and '%s' and Shift_ID='%s'and Stack_holder_ID='%d'\nand Station_ID='%d'" ("string"), w1338, w1337, w1331, 2 ("input 4"), 1 ("input 4")) -> (resulting string=w1334:string)  [unwired: 2 in, 1 out]
              n297 = call "Execute query.vi"("String"=w1334, "connection reference"=w1336) -> ("Table"=w1333:string[][], "connection reference 2"=w1332:T1)  [unwired: 6 in, 2 out]
            }
            frame "2" {
              w1354 = "%Y-%m-%d " ("time format string (%c)")
              n298 = Format Date/Time String(time format string (%c)=w1354, seconds (now)=w1353) -> (date/time string=w1350:string)  [unwired: 1 in]
              n299 = Format Date/Time String(time format string (%c)=w1354, seconds (now)=w1352) -> (date/time string=w1351:string)  [unwired: 1 in]
              n300 = Format Into String(format string="Select DATE,Production_Count,Station_ID,Stack_holder_ID\nfrom Production_COUNT\nWhere DATE between '%s' and '%s' and Shift_ID='%s'and Stack_holder_ID='%d'\nand Station_ID='%d'" ("string"), w1351, w1350, w1344, 2 ("input 4"), 1 ("input 4")) -> (resulting string=w1347:string)  [unwired: 2 in, 1 out]
              n301 = call "Execute query.vi"("String"=w1347, "connection reference"=w1349) -> ("Table"=w1346:string[][], "connection reference 2"=w1345:T1)  [unwired: 6 in, 2 out]
            }
            frame "3" {
              w1367 = "%Y-%m-%d " ("time format string (%c)")
              n302 = Format Date/Time String(time format string (%c)=w1367, seconds (now)=w1366) -> (date/time string=w1363:string)  [unwired: 1 in]
              n303 = Format Date/Time String(time format string (%c)=w1367, seconds (now)=w1365) -> (date/time string=w1364:string)  [unwired: 1 in]
              n304 = Format Into String(format string="Select DATE,Production_Count,Station_ID,Stack_holder_ID\nfrom Production_COUNT\nWhere DATE between '%s' and '%s' and Shift_ID='%s'and Stack_holder_ID='%d'\nand Station_ID='%d'" ("string"), w1364, w1363, w1357, 2 ("input 4"), 1 ("input 4")) -> (resulting string=w1360:string)  [unwired: 2 in, 1 out]
              n305 = call "Execute query.vi"("String"=w1360, "connection reference"=w1362) -> ("Table"=w1359:string[][], "connection reference 2"=w1358:T1)  [unwired: 6 in, 2 out]
            }
          }
        }
        frame "Gap Leader" {
          n306 = case shown="\"3\"" w1374 {
            selector: w1374 -> [_ _ w1389 w1401 w1413]
            tunnel: w1373 -> [_ w1386 w1398 w1410 w1422]
            tunnel: w1372 -> [_ w1385 w1397 w1409 w1421]
            tunnel: w1371 -> [_ _ _ _ _]
            tunnel: [_ w1379 w1391 w1403 w1415] -> w1370
            tunnel: w1369 -> [w1375 w1382 w1394 w1406 w1418]
            tunnel: [w1375 w1378 w1390 w1402 w1414] -> w1368
            frame "False", Default {
            }
            frame "ALL" {
              w1387 = "%Y-%m-%d " ("time format string (%c)")
              n307 = Format Date/Time String(time format string (%c)=w1387, seconds (now)=w1385) -> (date/time string=w1384:string)  [unwired: 1 in]
              n308 = Format Date/Time String(time format string (%c)=w1387, seconds (now)=w1386) -> (date/time string=w1383:string)  [unwired: 1 in]
              n309 = Format Into String(format string="Select DATE,Production_Count,Station_ID,Stack_holder_ID\nfrom Production_COUNT\nWhere DATE between '%s' and '%s' and Stack_holder_ID='%d'\nand Station_ID='%d'" ("string"), w1384, w1383, 1 ("input 3"), 1 ("input 3")) -> (resulting string=w1380:string)  [unwired: 2 in, 1 out]
              n310 = call "Execute query.vi"("String"=w1380, "connection reference"=w1382) -> ("Table"=w1379:string[][], "connection reference 2"=w1378:T1)  [unwired: 6 in, 2 out]
            }
            frame "1" {
              w1388 = 1 ("input 4")
              w1399 = "%Y-%m-%d " ("time format string (%c)")
              n311 = Format Date/Time String(time format string (%c)=w1399, seconds (now)=w1398) -> (date/time string=w1395:string)  [unwired: 1 in]
              n312 = Format Date/Time String(time format string (%c)=w1399, seconds (now)=w1397) -> (date/time string=w1396:string)  [unwired: 1 in]
              n313 = Format Into String(format string="Select DATE,Production_Count,Station_ID,Stack_holder_ID\nfrom Production_COUNT\nWhere DATE between '%s' and '%s' and Shift_ID='%s'and Stack_holder_ID='%d'\nand Station_ID='%d'" ("string"), w1396, w1395, w1389, w1388, w1388) -> (resulting string=w1392:string)  [unwired: 2 in, 1 out]
              n314 = call "Execute query.vi"("String"=w1392, "connection reference"=w1394) -> ("Table"=w1391:string[][], "connection reference 2"=w1390:T1)  [unwired: 6 in, 2 out]
            }
            frame "2" {
              w1400 = 1 ("input 4")
              w1411 = "%Y-%m-%d " ("time format string (%c)")
              n315 = Format Date/Time String(time format string (%c)=w1411, seconds (now)=w1410) -> (date/time string=w1407:string)  [unwired: 1 in]
              n316 = Format Date/Time String(time format string (%c)=w1411, seconds (now)=w1409) -> (date/time string=w1408:string)  [unwired: 1 in]
              n317 = Format Into String(format string="Select DATE,Production_Count,Station_ID,Stack_holder_ID\nfrom Production_COUNT\nWhere DATE between '%s' and '%s' and Shift_ID='%s'and Stack_holder_ID='%d'\nand Station_ID='%d'" ("string"), w1408, w1407, w1401, w1400, w1400) -> (resulting string=w1404:string)  [unwired: 2 in, 1 out]
              n318 = call "Execute query.vi"("String"=w1404, "connection reference"=w1406) -> ("Table"=w1403:string[][], "connection reference 2"=w1402:T1)  [unwired: 6 in, 2 out]
            }
            frame "3" {
              w1412 = 1 ("input 4")
              w1423 = "%Y-%m-%d " ("time format string (%c)")
              n319 = Format Date/Time String(time format string (%c)=w1423, seconds (now)=w1422) -> (date/time string=w1419:string)  [unwired: 1 in]
              n320 = Format Date/Time String(time format string (%c)=w1423, seconds (now)=w1421) -> (date/time string=w1420:string)  [unwired: 1 in]
              n321 = Format Into String(format string="Select DATE,Production_Count,Station_ID,Stack_holder_ID\nfrom Production_COUNT\nWhere DATE between '%s' and '%s' and Shift_ID='%s'and Stack_holder_ID='%d'\nand Station_ID='%d'" ("string"), w1420, w1419, w1413, w1412, w1412) -> (resulting string=w1416:string)  [unwired: 2 in, 1 out]
              n322 = call "Execute query.vi"("String"=w1416, "connection reference"=w1418) -> ("Table"=w1415:string[][], "connection reference 2"=w1414:T1)  [unwired: 6 in, 2 out]
            }
          }
        }
        frame "Maintenance" {
          n323 = case shown="\"ALL\"" w1430 {
            selector: w1430 -> [_ _ w1446 w1459 w1472]
            tunnel: w1429 -> [_ w1442 w1455 w1468 w1481]
            tunnel: w1428 -> [_ w1441 w1454 w1467 w1480]
            tunnel: w1427 -> [_ _ _ _ _]
            tunnel: [_ w1435 w1448 w1461 w1474] -> w1426
            tunnel: w1425 -> [w1431 w1438 w1451 w1464 w1477]
            tunnel: [w1431 w1434 w1447 w1460 w1473] -> w1424
            frame "False", Default {
            }
            frame "ALL" {
              w1443 = "%Y-%m-%d " ("time format string (%c)")
              n324 = Format Date/Time String(time format string (%c)=w1443, seconds (now)=w1441) -> (date/time string=w1440:string)  [unwired: 1 in]
              n325 = Format Date/Time String(time format string (%c)=w1443, seconds (now)=w1442) -> (date/time string=w1439:string)  [unwired: 1 in]
              n326 = Format Into String(format string="Select DATE,Production_Count,Station_ID,Stack_holder_ID\nfrom Production_COUNT\nWhere DATE between '%s' and '%s' and Stack_holder_ID='%d'\nand Station_ID='%d'" ("string"), w1440, w1439, 3 ("input 3"), 1 ("input 4")) -> (resulting string=w1436:string)  [unwired: 2 in, 1 out]
              n327 = call "Execute query.vi"("String"=w1436, "connection reference"=w1438) -> ("Table"=w1435:string[][], "connection reference 2"=w1434:T1)  [unwired: 6 in, 2 out]
            }
            frame "1" {
              w1456 = "%Y-%m-%d " ("time format string (%c)")
              n328 = Format Date/Time String(time format string (%c)=w1456, seconds (now)=w1455) -> (date/time string=w1452:string)  [unwired: 1 in]
              n329 = Format Date/Time String(time format string (%c)=w1456, seconds (now)=w1454) -> (date/time string=w1453:string)  [unwired: 1 in]
              n330 = Format Into String(format string="Select DATE,Production_Count,Station_ID,Stack_holder_ID\nfrom Production_COUNT\nWhere DATE between '%s' and '%s' and Shift_ID='%s'and Stack_holder_ID='%d'\nand Station_ID='%d'" ("string"), w1453, w1452, w1446, 3 ("input 4"), 1 ("input 5")) -> (resulting string=w1449:string)  [unwired: 2 in, 1 out]
              n331 = call "Execute query.vi"("String"=w1449, "connection reference"=w1451) -> ("Table"=w1448:string[][], "connection reference 2"=w1447:T1)  [unwired: 6 in, 2 out]
            }
            frame "2" {
              w1469 = "%Y-%m-%d " ("time format string (%c)")
              n332 = Format Date/Time String(time format string (%c)=w1469, seconds (now)=w1468) -> (date/time string=w1465:string)  [unwired: 1 in]
              n333 = Format Date/Time String(time format string (%c)=w1469, seconds (now)=w1467) -> (date/time string=w1466:string)  [unwired: 1 in]
              n334 = Format Into String(format string="Select DATE,Production_Count,Station_ID,Stack_holder_ID\nfrom Production_COUNT\nWhere DATE between '%s' and '%s' and Shift_ID='%s'and Stack_holder_ID='%d'\nand Station_ID='%d'" ("string"), w1466, w1465, w1459, 3 ("input 4"), 1 ("input 5")) -> (resulting string=w1462:string)  [unwired: 2 in, 1 out]
              n335 = call "Execute query.vi"("String"=w1462, "connection reference"=w1464) -> ("Table"=w1461:string[][], "connection reference 2"=w1460:T1)  [unwired: 6 in, 2 out]
            }
            frame "3" {
              w1482 = "%Y-%m-%d " ("time format string (%c)")
              n336 = Format Date/Time String(time format string (%c)=w1482, seconds (now)=w1481) -> (date/time string=w1478:string)  [unwired: 1 in]
              n337 = Format Date/Time String(time format string (%c)=w1482, seconds (now)=w1480) -> (date/time string=w1479:string)  [unwired: 1 in]
              n338 = Format Into String(format string="Select DATE,Production_Count,Station_ID,Stack_holder_ID\nfrom Production_COUNT\nWhere DATE between '%s' and '%s' and Shift_ID='%s'and Stack_holder_ID='%d'\nand Station_ID='%d'" ("string"), w1479, w1478, w1472, 3 ("input 4"), 1 ("input 5")) -> (resulting string=w1475:string)  [unwired: 2 in, 1 out]
              n339 = call "Execute query.vi"("String"=w1475, "connection reference"=w1477) -> ("Table"=w1474:string[][], "connection reference 2"=w1473:T1)  [unwired: 6 in, 2 out]
            }
          }
        }
        frame "Quality" {
          n340 = case shown="\"ALL\"" w1489 {
            selector: w1489 -> [_ _ w1505 w1518 w1531]
            tunnel: w1488 -> [_ w1501 w1514 w1527 w1540]
            tunnel: w1487 -> [_ w1500 w1513 w1526 w1539]
            tunnel: w1486 -> [_ _ _ _ _]
            tunnel: [_ w1494 w1507 w1520 w1533] -> w1485
            tunnel: w1484 -> [w1490 w1497 w1510 w1523 w1536]
            tunnel: [w1490 w1493 w1506 w1519 w1532] -> w1483
            frame "False", Default {
            }
            frame "ALL" {
              w1502 = "%Y-%m-%d " ("time format string (%c)")
              n341 = Format Date/Time String(time format string (%c)=w1502, seconds (now)=w1500) -> (date/time string=w1499:string)  [unwired: 1 in]
              n342 = Format Date/Time String(time format string (%c)=w1502, seconds (now)=w1501) -> (date/time string=w1498:string)  [unwired: 1 in]
              n343 = Format Into String(format string="Select DATE,Production_Count,Station_ID,Stack_holder_ID\nfrom Production_COUNT\nWhere DATE between '%s' and '%s' and Stack_holder_ID='%d'\nand Station_ID='%d'" ("string"), w1499, w1498, 4 ("input 3"), 1 ("input 3")) -> (resulting string=w1495:string)  [unwired: 2 in, 1 out]
              n344 = call "Execute query.vi"("String"=w1495, "connection reference"=w1497) -> ("Table"=w1494:string[][], "connection reference 2"=w1493:T1)  [unwired: 6 in, 2 out]
            }
            frame "1" {
              w1515 = "%Y-%m-%d " ("time format string (%c)")
              n345 = Format Date/Time String(time format string (%c)=w1515, seconds (now)=w1514) -> (date/time string=w1511:string)  [unwired: 1 in]
              n346 = Format Date/Time String(time format string (%c)=w1515, seconds (now)=w1513) -> (date/time string=w1512:string)  [unwired: 1 in]
              n347 = Format Into String(format string="Select DATE,Production_Count,Station_ID,Stack_holder_ID\nfrom Production_COUNT\nWhere DATE between '%s' and '%s' and Shift_ID='%s'and Stack_holder_ID='%d'\nand Station_ID='%d'" ("string"), w1512, w1511, w1505, 4 ("input 4"), 1 ("input 4")) -> (resulting string=w1508:string)  [unwired: 2 in, 1 out]
              n348 = call "Execute query.vi"("String"=w1508, "connection reference"=w1510) -> ("Table"=w1507:string[][], "connection reference 2"=w1506:T1)  [unwired: 6 in, 2 out]
            }
            frame "2" {
              w1528 = "%Y-%m-%d " ("time format string (%c)")
              n349 = Format Date/Time String(time format string (%c)=w1528, seconds (now)=w1527) -> (date/time string=w1524:string)  [unwired: 1 in]
              n350 = Format Date/Time String(time format string (%c)=w1528, seconds (now)=w1526) -> (date/time string=w1525:string)  [unwired: 1 in]
              n351 = Format Into String(format string="Select DATE,Production_Count,Station_ID,Stack_holder_ID\nfrom Production_COUNT\nWhere DATE between '%s' and '%s' and Shift_ID='%s'and Stack_holder_ID='%d'\nand Station_ID='%d'" ("string"), w1525, w1524, w1518, 4 ("input 4"), 1 ("input 4")) -> (resulting string=w1521:string)  [unwired: 2 in, 1 out]
              n352 = call "Execute query.vi"("String"=w1521, "connection reference"=w1523) -> ("Table"=w1520:string[][], "connection reference 2"=w1519:T1)  [unwired: 6 in, 2 out]
            }
            frame "3" {
              w1541 = "%Y-%m-%d " ("time format string (%c)")
              n353 = Format Date/Time String(time format string (%c)=w1541, seconds (now)=w1540) -> (date/time string=w1537:string)  [unwired: 1 in]
              n354 = Format Date/Time String(time format string (%c)=w1541, seconds (now)=w1539) -> (date/time string=w1538:string)  [unwired: 1 in]
              n355 = Format Into String(format string="Select DATE,Production_Count,Station_ID,Stack_holder_ID\nfrom Production_COUNT\nWhere DATE between '%s' and '%s' and Shift_ID='%s'and Stack_holder_ID='%d'\nand Station_ID='%d'" ("string"), w1538, w1537, w1531, 4 ("input 4"), 1 ("input 4")) -> (resulting string=w1534:string)  [unwired: 2 in, 1 out]
              n356 = call "Execute query.vi"("String"=w1534, "connection reference"=w1536) -> ("Table"=w1533:string[][], "connection reference 2"=w1532:T1)  [unwired: 6 in, 2 out]
            }
          }
        }
        frame "Production" {
          n357 = case shown="\"False\", Default" w1548 {
            selector: w1548 -> [_ _ w1564 w1577 w1590]
            tunnel: w1547 -> [_ w1560 w1573 w1586 w1599]
            tunnel: w1546 -> [_ w1559 w1572 w1585 w1598]
            tunnel: w1545 -> [_ _ _ _ _]
            tunnel: [_ w1553 w1566 w1579 w1592] -> w1544
            tunnel: w1543 -> [w1549 w1556 w1569 w1582 w1595]
            tunnel: [w1549 w1552 w1565 w1578 w1591] -> w1542
            frame "False", Default {
            }
            frame "ALL" {
              w1561 = "%Y-%m-%d " ("time format string (%c)")
              n358 = Format Date/Time String(time format string (%c)=w1561, seconds (now)=w1559) -> (date/time string=w1558:string)  [unwired: 1 in]
              n359 = Format Date/Time String(time format string (%c)=w1561, seconds (now)=w1560) -> (date/time string=w1557:string)  [unwired: 1 in]
              n360 = Format Into String(format string="Select DATE,Production_Count,Station_ID,Stack_holder_ID\nfrom Production_COUNT\nWhere DATE between '%s' and '%s' and Stack_holder_ID='%d'\nand Station_ID='%d'" ("string"), w1558, w1557, 5 ("input 3"), 1 ("input 3")) -> (resulting string=w1554:string)  [unwired: 2 in, 1 out]
              n361 = call "Execute query.vi"("String"=w1554, "connection reference"=w1556) -> ("Table"=w1553:string[][], "connection reference 2"=w1552:T1)  [unwired: 6 in, 2 out]
            }
            frame "1" {
              w1574 = "%Y-%m-%d " ("time format string (%c)")
              n362 = Format Date/Time String(time format string (%c)=w1574, seconds (now)=w1573) -> (date/time string=w1570:string)  [unwired: 1 in]
              n363 = Format Date/Time String(time format string (%c)=w1574, seconds (now)=w1572) -> (date/time string=w1571:string)  [unwired: 1 in]
              n364 = Format Into String(format string="Select DATE,Production_Count,Station_ID,Stack_holder_ID\nfrom Production_COUNT\nWhere DATE between '%s' and '%s' and Shift_ID='%s'and Stack_holder_ID='%d'\nand Station_ID='%d'" ("string"), w1571, w1570, w1564, 5 ("input 4"), 1 ("input 4")) -> (resulting string=w1567:string)  [unwired: 2 in, 1 out]
              n365 = call "Execute query.vi"("String"=w1567, "connection reference"=w1569) -> ("Table"=w1566:string[][], "connection reference 2"=w1565:T1)  [unwired: 6 in, 2 out]
            }
            frame "2" {
              w1587 = "%Y-%m-%d " ("time format string (%c)")
              n366 = Format Date/Time String(time format string (%c)=w1587, seconds (now)=w1586) -> (date/time string=w1583:string)  [unwired: 1 in]
              n367 = Format Date/Time String(time format string (%c)=w1587, seconds (now)=w1585) -> (date/time string=w1584:string)  [unwired: 1 in]
              n368 = Format Into String(format string="Select DATE,Production_Count,Station_ID,Stack_holder_ID\nfrom Production_COUNT\nWhere DATE between '%s' and '%s' and Shift_ID='%s'and Stack_holder_ID='%d'\nand Station_ID='%d'" ("string"), w1584, w1583, w1577, 5 ("input 4"), 1 ("input 4")) -> (resulting string=w1580:string)  [unwired: 2 in, 1 out]
              n369 = call "Execute query.vi"("String"=w1580, "connection reference"=w1582) -> ("Table"=w1579:string[][], "connection reference 2"=w1578:T1)  [unwired: 6 in, 2 out]
            }
            frame "3" {
              w1600 = "%Y-%m-%d " ("time format string (%c)")
              n370 = Format Date/Time String(time format string (%c)=w1600, seconds (now)=w1599) -> (date/time string=w1596:string)  [unwired: 1 in]
              n371 = Format Date/Time String(time format string (%c)=w1600, seconds (now)=w1598) -> (date/time string=w1597:string)  [unwired: 1 in]
              n372 = Format Into String(format string="Select DATE,Production_Count,Station_ID,Stack_holder_ID\nfrom Production_COUNT\nWhere DATE between '%s' and '%s' and Shift_ID='%s'and Stack_holder_ID='%d'\nand Station_ID='%d'" ("string"), w1597, w1596, w1590, 5 ("input 4"), 1 ("input 4")) -> (resulting string=w1593:string)  [unwired: 2 in, 1 out]
              n373 = call "Execute query.vi"("String"=w1593, "connection reference"=w1595) -> ("Table"=w1592:string[][], "connection reference 2"=w1591:T1)  [unwired: 6 in, 2 out]
            }
          }
        }
      }
    }
    frame "ST 3" {
      n374 = case shown="\"ALL\", Default" w1607 {
        tunnel: w1613 -> [w1625 w1790 w1849 w1905 w1964 w2023]
        tunnel: w1612 -> [w1624 w1789 w1848 w1904 w1963 w2022]
        tunnel: w1611 -> [w1623 w1788 w1847 w1903 w1962 w2021]
        tunnel: w1610 -> [w1622 w1787 w1846 w1902 w1961 w2020]
        tunnel: [w1621 w1786 w1845 w1901 w1960 w2019] -> w1604
        tunnel: w1609 -> [w1620 w1785 w1844 w1900 w1959 w2018]
        tunnel: [w1619 w1784 w1843 w1899 w1958 w2017] -> w1608
        tunnel: w1606 -> [w1618 _ _ _ _ _]
        tunnel: w1605 -> [w1617 _ _ _ _ _]
        tunnel: w1603 -> [w1616 _ _ _ _ _]
        tunnel: w1602 -> [w1615 _ _ _ _ _]
        tunnel: [w1614 _ _ _ _ _] -> w1601
        frame "ALL", Default {
          n375 = case shown="\"1\"" w1625 {
            selector: w1625 -> [_ w1664 w1704 w1744]
            tunnel: w1624 -> [_ _ _ _]
            tunnel: w1623 -> [_ _ _ _]
            tunnel: w1622 -> [_ _ _ _]
            tunnel: [w1628 w1667 w1707 w1747] -> w1621
            tunnel: w1620 -> [w1634 w1673 w1713 w1753]
            tunnel: [w1633 w1672 w1712 w1752] -> w1619
            tunnel: w1618 -> [w1632 w1671 w1711 w1751]
            tunnel: w1617 -> [w1631 w1670 w1710 w1750]
            tunnel: w1616 -> [w1629 w1668 w1708 w1748]
            tunnel: w1615 -> [w1627 w1666 w1706 w1746]
            tunnel: [w1626 w1665 w1705 w1745] -> w1614
            frame "ALL", Default {
              n376 = for {
                tunnel: w1632 -> [w1646]
                tunnel: w1631 -> [w1645]
                shift-right: [w1648] -> w1633
                shift-left: w1634 -> [w1650]
                shift-right: [w1637] -> w1628
                shift-left: string[][] [] -> [w1639]
                tunnel: w1629 -> [w1640] mode=indexing
                tunnel: w1627 -> [w1636]
                tunnel: [w1635] -> w1626
                n377 = case shown="\"April\"" w1645 {
                  tunnel: ["1" "1" "2" "3" "4" "5" "6" "7" "8" "9" "10" "11" "12"] -> w1644
                  frame "False", Default {
                  }
                  frame "January" {
                  }
                  frame "February" {
                  }
                  frame "March" {
                  }
                  frame "April" {
                  }
                  frame "May" {
                  }
                  frame "June" {
                  }
                  frame "July" {
                  }
                  frame "August" {
                  }
                  frame "September" {
                  }
                  frame "October" {
                  }
                  frame "November" {
                  }
                  frame "December" {
                  }
                }
                n378 = Concatenate Strings("Select DISTINCT PLAN_DATE,PRODUCTION_COUNT,STATION_ID,DATE\nfrom ", w1640, " Where year( PLAN_DATE) ='%s' and month(PLAN_DATE) = '%s' and STATION_ID='%d'") -> (w1641:string)
                n379 = Format Into String(format string=w1641, w1646, w1644, 3 ("input 3")) -> (resulting string=w1649:string)  [unwired: 2 in, 1 out]
                n380 = call "Execute query.vi"("error in (no error)"=w1636, "String"=w1649, "connection reference"=w1650) -> ("error out"=w1635:errorcluster, "Table"=w1638:string[][], "connection reference 2"=w1648:T1)  [unwired: 5 in, 1 out]
                n381 = Build Array (concatenate)(w1639, w1638) -> (w1637:string[][])
              }
            }
            frame "1" {
              n382 = for {
                tunnel: w1671 -> [w1686]
                tunnel: w1670 -> [w1685]
                shift-right: [w1688] -> w1672
                shift-left: w1673 -> [w1690]
                shift-right: [w1677] -> w1667
                shift-left: string[][] [] -> [w1679]
                tunnel: w1668 -> [w1680] mode=indexing
                tunnel: w1666 -> [w1676]
                tunnel: [w1675] -> w1665
                tunnel: w1664 -> [w1674]
                n383 = case shown="\"April\"" w1685 {
                  tunnel: ["1" "1" "2" "3" "4" "5" "6" "7" "8" "9" "10" "11" "12"] -> w1684
                  frame "False", Default {
                  }
                  frame "January" {
                  }
                  frame "February" {
                  }
                  frame "March" {
                  }
                  frame "April" {
                  }
                  frame "May" {
                  }
                  frame "June" {
                  }
                  frame "July" {
                  }
                  frame "August" {
                  }
                  frame "September" {
                  }
                  frame "October" {
                  }
                  frame "November" {
                  }
                  frame "December" {
                  }
                }
                n384 = Concatenate Strings("Select DISTINCT PLAN_DATE,PRODUCTION_COUNT,STATION_ID,DATE\nfrom ", w1680, " Where year( PLAN_DATE) ='%s' and month(PLAN_DATE) = '%s' and STATION_ID='%d' and SHIFT='%s'") -> (w1681:string)
                n385 = Format Into String(format string=w1681, w1686, w1684, 3 ("input 3"), w1674) -> (resulting string=w1689:string)  [unwired: 2 in, 1 out]
                n386 = call "Execute query.vi"("error in (no error)"=w1676, "String"=w1689, "connection reference"=w1690) -> ("error out"=w1675:errorcluster, "Table"=w1678:string[][], "connection reference 2"=w1688:T1)  [unwired: 5 in, 1 out]
                n387 = Build Array (concatenate)(w1679, w1678) -> (w1677:string[][])
              }
            }
            frame "2" {
              n388 = for {
                tunnel: w1711 -> [w1726]
                tunnel: w1710 -> [w1725]
                shift-right: [w1728] -> w1712
                shift-left: w1713 -> [w1730]
                shift-right: [w1717] -> w1707
                shift-left: string[][] [] -> [w1719]
                tunnel: w1708 -> [w1720] mode=indexing
                tunnel: w1706 -> [w1716]
                tunnel: [w1715] -> w1705
                tunnel: w1704 -> [w1714]
                n389 = case shown="\"April\"" w1725 {
                  tunnel: ["1" "1" "2" "3" "4" "5" "6" "7" "8" "9" "10" "11" "12"] -> w1724
                  frame "False", Default {
                  }
                  frame "January" {
                  }
                  frame "February" {
                  }
                  frame "March" {
                  }
                  frame "April" {
                  }
                  frame "May" {
                  }
                  frame "June" {
                  }
                  frame "July" {
                  }
                  frame "August" {
                  }
                  frame "September" {
                  }
                  frame "October" {
                  }
                  frame "November" {
                  }
                  frame "December" {
                  }
                }
                n390 = Concatenate Strings("Select DISTINCT PLAN_DATE,PRODUCTION_COUNT,STATION_ID,DATE\nfrom ", w1720, " Where year( PLAN_DATE) ='%s' and month(PLAN_DATE) = '%s' and STATION_ID='%d' and SHIFT='%s'") -> (w1721:string)
                n391 = Format Into String(format string=w1721, w1726, w1724, 3 ("input 3"), w1714) -> (resulting string=w1729:string)  [unwired: 2 in, 1 out]
                n392 = call "Execute query.vi"("error in (no error)"=w1716, "String"=w1729, "connection reference"=w1730) -> ("error out"=w1715:errorcluster, "Table"=w1718:string[][], "connection reference 2"=w1728:T1)  [unwired: 5 in, 1 out]
                n393 = Build Array (concatenate)(w1719, w1718) -> (w1717:string[][])
              }
            }
            frame "3" {
              n394 = for {
                tunnel: w1751 -> [w1766]
                tunnel: w1750 -> [w1765]
                shift-right: [w1768] -> w1752
                shift-left: w1753 -> [w1770]
                shift-right: [w1757] -> w1747
                shift-left: string[][] [] -> [w1759]
                tunnel: w1748 -> [w1760] mode=indexing
                tunnel: w1746 -> [w1756]
                tunnel: [w1755] -> w1745
                tunnel: w1744 -> [w1754]
                n395 = case shown="\"April\"" w1765 {
                  tunnel: ["1" "1" "2" "3" "4" "5" "6" "7" "8" "9" "10" "11" "12"] -> w1764
                  frame "False", Default {
                  }
                  frame "January" {
                  }
                  frame "February" {
                  }
                  frame "March" {
                  }
                  frame "April" {
                  }
                  frame "May" {
                  }
                  frame "June" {
                  }
                  frame "July" {
                  }
                  frame "August" {
                  }
                  frame "September" {
                  }
                  frame "October" {
                  }
                  frame "November" {
                  }
                  frame "December" {
                  }
                }
                n396 = Concatenate Strings("Select DISTINCT PLAN_DATE,PRODUCTION_COUNT,STATION_ID,DATE\nfrom ", w1760, " Where year( PLAN_DATE) ='%s' and month(PLAN_DATE) = '%s' and STATION_ID='%d' and SHIFT='%s'") -> (w1761:string)
                n397 = Format Into String(format string=w1761, w1766, w1764, 3 ("input 3"), w1754) -> (resulting string=w1769:string)  [unwired: 2 in, 1 out]
                n398 = call "Execute query.vi"("error in (no error)"=w1756, "String"=w1769, "connection reference"=w1770) -> ("error out"=w1755:errorcluster, "Table"=w1758:string[][], "connection reference 2"=w1768:T1)  [unwired: 5 in, 1 out]
                n399 = Build Array (concatenate)(w1759, w1758) -> (w1757:string[][])
              }
            }
          }
        }
        frame "Logistics" {
          n400 = case shown="\"ALL\"" w1790 {
            selector: w1790 -> [_ _ w1806 w1819 w1832]
            tunnel: w1789 -> [_ w1802 w1815 w1828 w1841]
            tunnel: w1788 -> [_ w1801 w1814 w1827 w1840]
            tunnel: w1787 -> [_ _ _ _ _]
            tunnel: [_ w1795 w1808 w1821 w1834] -> w1786
            tunnel: w1785 -> [w1791 w1798 w1811 w1824 w1837]
            tunnel: [w1791 w1794 w1807 w1820 w1833] -> w1784
            frame "False", Default {
            }
            frame "ALL" {
              w1803 = "%Y-%m-%d " ("time format string (%c)")
              n401 = Format Date/Time String(time format string (%c)=w1803, seconds (now)=w1801) -> (date/time string=w1800:string)  [unwired: 1 in]
              n402 = Format Date/Time String(time format string (%c)=w1803, seconds (now)=w1802) -> (date/time string=w1799:string)  [unwired: 1 in]
              n403 = Format Into String(format string="Select DATE,Production_Count,Station_ID,Stack_holder_ID\nfrom Production_COUNT\nWhere DATE between '%s' and '%s' and Stack_holder_ID='%d'\nand Station_ID='%d'" ("string"), w1800, w1799, 2 ("input 3"), 1 ("input 4")) -> (resulting string=w1796:string)  [unwired: 2 in, 1 out]
              n404 = call "Execute query.vi"("String"=w1796, "connection reference"=w1798) -> ("Table"=w1795:string[][], "connection reference 2"=w1794:T1)  [unwired: 6 in, 2 out]
            }
            frame "1" {
              w1816 = "%Y-%m-%d " ("time format string (%c)")
              n405 = Format Date/Time String(time format string (%c)=w1816, seconds (now)=w1815) -> (date/time string=w1812:string)  [unwired: 1 in]
              n406 = Format Date/Time String(time format string (%c)=w1816, seconds (now)=w1814) -> (date/time string=w1813:string)  [unwired: 1 in]
              n407 = Format Into String(format string="Select DATE,Production_Count,Station_ID,Stack_holder_ID\nfrom Production_COUNT\nWhere DATE between '%s' and '%s' and Shift_ID='%s'and Stack_holder_ID='%d'\nand Station_ID='%d'" ("string"), w1813, w1812, w1806, 2 ("input 4"), 1 ("input 4")) -> (resulting string=w1809:string)  [unwired: 2 in, 1 out]
              n408 = call "Execute query.vi"("String"=w1809, "connection reference"=w1811) -> ("Table"=w1808:string[][], "connection reference 2"=w1807:T1)  [unwired: 6 in, 2 out]
            }
            frame "2" {
              w1829 = "%Y-%m-%d " ("time format string (%c)")
              n409 = Format Date/Time String(time format string (%c)=w1829, seconds (now)=w1828) -> (date/time string=w1825:string)  [unwired: 1 in]
              n410 = Format Date/Time String(time format string (%c)=w1829, seconds (now)=w1827) -> (date/time string=w1826:string)  [unwired: 1 in]
              n411 = Format Into String(format string="Select DATE,Production_Count,Station_ID,Stack_holder_ID\nfrom Production_COUNT\nWhere DATE between '%s' and '%s' and Shift_ID='%s'and Stack_holder_ID='%d'\nand Station_ID='%d'" ("string"), w1826, w1825, w1819, 2 ("input 4"), 1 ("input 4")) -> (resulting string=w1822:string)  [unwired: 2 in, 1 out]
              n412 = call "Execute query.vi"("String"=w1822, "connection reference"=w1824) -> ("Table"=w1821:string[][], "connection reference 2"=w1820:T1)  [unwired: 6 in, 2 out]
            }
            frame "3" {
              w1842 = "%Y-%m-%d " ("time format string (%c)")
              n413 = Format Date/Time String(time format string (%c)=w1842, seconds (now)=w1841) -> (date/time string=w1838:string)  [unwired: 1 in]
              n414 = Format Date/Time String(time format string (%c)=w1842, seconds (now)=w1840) -> (date/time string=w1839:string)  [unwired: 1 in]
              n415 = Format Into String(format string="Select DATE,Production_Count,Station_ID,Stack_holder_ID\nfrom Production_COUNT\nWhere DATE between '%s' and '%s' and Shift_ID='%s'and Stack_holder_ID='%d'\nand Station_ID='%d'" ("string"), w1839, w1838, w1832, 2 ("input 4"), 1 ("input 4")) -> (resulting string=w1835:string)  [unwired: 2 in, 1 out]
              n416 = call "Execute query.vi"("String"=w1835, "connection reference"=w1837) -> ("Table"=w1834:string[][], "connection reference 2"=w1833:T1)  [unwired: 6 in, 2 out]
            }
          }
        }
        frame "Gap Leader" {
          n417 = case shown="\"3\"" w1849 {
            selector: w1849 -> [_ _ w1864 w1876 w1888]
            tunnel: w1848 -> [_ w1861 w1873 w1885 w1897]
            tunnel: w1847 -> [_ w1860 w1872 w1884 w1896]
            tunnel: w1846 -> [_ _ _ _ _]
            tunnel: [_ w1854 w1866 w1878 w1890] -> w1845
            tunnel: w1844 -> [w1850 w1857 w1869 w1881 w1893]
            tunnel: [w1850 w1853 w1865 w1877 w1889] -> w1843
            frame "False", Default {
            }
            frame "ALL" {
              w1862 = "%Y-%m-%d " ("time format string (%c)")
              n418 = Format Date/Time String(time format string (%c)=w1862, seconds (now)=w1860) -> (date/time string=w1859:string)  [unwired: 1 in]
              n419 = Format Date/Time String(time format string (%c)=w1862, seconds (now)=w1861) -> (date/time string=w1858:string)  [unwired: 1 in]
              n420 = Format Into String(format string="Select DATE,Production_Count,Station_ID,Stack_holder_ID\nfrom Production_COUNT\nWhere DATE between '%s' and '%s' and Stack_holder_ID='%d'\nand Station_ID='%d'" ("string"), w1859, w1858, 1 ("input 3"), 1 ("input 3")) -> (resulting string=w1855:string)  [unwired: 2 in, 1 out]
              n421 = call "Execute query.vi"("String"=w1855, "connection reference"=w1857) -> ("Table"=w1854:string[][], "connection reference 2"=w1853:T1)  [unwired: 6 in, 2 out]
            }
            frame "1" {
              w1863 = 1 ("input 4")
              w1874 = "%Y-%m-%d " ("time format string (%c)")
              n422 = Format Date/Time String(time format string (%c)=w1874, seconds (now)=w1873) -> (date/time string=w1870:string)  [unwired: 1 in]
              n423 = Format Date/Time String(time format string (%c)=w1874, seconds (now)=w1872) -> (date/time string=w1871:string)  [unwired: 1 in]
              n424 = Format Into String(format string="Select DATE,Production_Count,Station_ID,Stack_holder_ID\nfrom Production_COUNT\nWhere DATE between '%s' and '%s' and Shift_ID='%s'and Stack_holder_ID='%d'\nand Station_ID='%d'" ("string"), w1871, w1870, w1864, w1863, w1863) -> (resulting string=w1867:string)  [unwired: 2 in, 1 out]
              n425 = call "Execute query.vi"("String"=w1867, "connection reference"=w1869) -> ("Table"=w1866:string[][], "connection reference 2"=w1865:T1)  [unwired: 6 in, 2 out]
            }
            frame "2" {
              w1875 = 1 ("input 4")
              w1886 = "%Y-%m-%d " ("time format string (%c)")
              n426 = Format Date/Time String(time format string (%c)=w1886, seconds (now)=w1885) -> (date/time string=w1882:string)  [unwired: 1 in]
              n427 = Format Date/Time String(time format string (%c)=w1886, seconds (now)=w1884) -> (date/time string=w1883:string)  [unwired: 1 in]
              n428 = Format Into String(format string="Select DATE,Production_Count,Station_ID,Stack_holder_ID\nfrom Production_COUNT\nWhere DATE between '%s' and '%s' and Shift_ID='%s'and Stack_holder_ID='%d'\nand Station_ID='%d'" ("string"), w1883, w1882, w1876, w1875, w1875) -> (resulting string=w1879:string)  [unwired: 2 in, 1 out]
              n429 = call "Execute query.vi"("String"=w1879, "connection reference"=w1881) -> ("Table"=w1878:string[][], "connection reference 2"=w1877:T1)  [unwired: 6 in, 2 out]
            }
            frame "3" {
              w1887 = 1 ("input 4")
              w1898 = "%Y-%m-%d " ("time format string (%c)")
              n430 = Format Date/Time String(time format string (%c)=w1898, seconds (now)=w1897) -> (date/time string=w1894:string)  [unwired: 1 in]
              n431 = Format Date/Time String(time format string (%c)=w1898, seconds (now)=w1896) -> (date/time string=w1895:string)  [unwired: 1 in]
              n432 = Format Into String(format string="Select DATE,Production_Count,Station_ID,Stack_holder_ID\nfrom Production_COUNT\nWhere DATE between '%s' and '%s' and Shift_ID='%s'and Stack_holder_ID='%d'\nand Station_ID='%d'" ("string"), w1895, w1894, w1888, w1887, w1887) -> (resulting string=w1891:string)  [unwired: 2 in, 1 out]
              n433 = call "Execute query.vi"("String"=w1891, "connection reference"=w1893) -> ("Table"=w1890:string[][], "connection reference 2"=w1889:T1)  [unwired: 6 in, 2 out]
            }
          }
        }
        frame "Maintenance" {
          n434 = case shown="\"ALL\"" w1905 {
            selector: w1905 -> [_ _ w1921 w1934 w1947]
            tunnel: w1904 -> [_ w1917 w1930 w1943 w1956]
            tunnel: w1903 -> [_ w1916 w1929 w1942 w1955]
            tunnel: w1902 -> [_ _ _ _ _]
            tunnel: [_ w1910 w1923 w1936 w1949] -> w1901
            tunnel: w1900 -> [w1906 w1913 w1926 w1939 w1952]
            tunnel: [w1906 w1909 w1922 w1935 w1948] -> w1899
            frame "False", Default {
            }
            frame "ALL" {
              w1918 = "%Y-%m-%d " ("time format string (%c)")
              n435 = Format Date/Time String(time format string (%c)=w1918, seconds (now)=w1916) -> (date/time string=w1915:string)  [unwired: 1 in]
              n436 = Format Date/Time String(time format string (%c)=w1918, seconds (now)=w1917) -> (date/time string=w1914:string)  [unwired: 1 in]
              n437 = Format Into String(format string="Select DATE,Production_Count,Station_ID,Stack_holder_ID\nfrom Production_COUNT\nWhere DATE between '%s' and '%s' and Stack_holder_ID='%d'\nand Station_ID='%d'" ("string"), w1915, w1914, 3 ("input 3"), 1 ("input 4")) -> (resulting string=w1911:string)  [unwired: 2 in, 1 out]
              n438 = call "Execute query.vi"("String"=w1911, "connection reference"=w1913) -> ("Table"=w1910:string[][], "connection reference 2"=w1909:T1)  [unwired: 6 in, 2 out]
            }
            frame "1" {
              w1931 = "%Y-%m-%d " ("time format string (%c)")
              n439 = Format Date/Time String(time format string (%c)=w1931, seconds (now)=w1930) -> (date/time string=w1927:string)  [unwired: 1 in]
              n440 = Format Date/Time String(time format string (%c)=w1931, seconds (now)=w1929) -> (date/time string=w1928:string)  [unwired: 1 in]
              n441 = Format Into String(format string="Select DATE,Production_Count,Station_ID,Stack_holder_ID\nfrom Production_COUNT\nWhere DATE between '%s' and '%s' and Shift_ID='%s'and Stack_holder_ID='%d'\nand Station_ID='%d'" ("string"), w1928, w1927, w1921, 3 ("input 4"), 1 ("input 5")) -> (resulting string=w1924:string)  [unwired: 2 in, 1 out]
              n442 = call "Execute query.vi"("String"=w1924, "connection reference"=w1926) -> ("Table"=w1923:string[][], "connection reference 2"=w1922:T1)  [unwired: 6 in, 2 out]
            }
            frame "2" {
              w1944 = "%Y-%m-%d " ("time format string (%c)")
              n443 = Format Date/Time String(time format string (%c)=w1944, seconds (now)=w1943) -> (date/time string=w1940:string)  [unwired: 1 in]
              n444 = Format Date/Time String(time format string (%c)=w1944, seconds (now)=w1942) -> (date/time string=w1941:string)  [unwired: 1 in]
              n445 = Format Into String(format string="Select DATE,Production_Count,Station_ID,Stack_holder_ID\nfrom Production_COUNT\nWhere DATE between '%s' and '%s' and Shift_ID='%s'and Stack_holder_ID='%d'\nand Station_ID='%d'" ("string"), w1941, w1940, w1934, 3 ("input 4"), 1 ("input 5")) -> (resulting string=w1937:string)  [unwired: 2 in, 1 out]
              n446 = call "Execute query.vi"("String"=w1937, "connection reference"=w1939) -> ("Table"=w1936:string[][], "connection reference 2"=w1935:T1)  [unwired: 6 in, 2 out]
            }
            frame "3" {
              w1957 = "%Y-%m-%d " ("time format string (%c)")
              n447 = Format Date/Time String(time format string (%c)=w1957, seconds (now)=w1956) -> (date/time string=w1953:string)  [unwired: 1 in]
              n448 = Format Date/Time String(time format string (%c)=w1957, seconds (now)=w1955) -> (date/time string=w1954:string)  [unwired: 1 in]
              n449 = Format Into String(format string="Select DATE,Production_Count,Station_ID,Stack_holder_ID\nfrom Production_COUNT\nWhere DATE between '%s' and '%s' and Shift_ID='%s'and Stack_holder_ID='%d'\nand Station_ID='%d'" ("string"), w1954, w1953, w1947, 3 ("input 4"), 1 ("input 5")) -> (resulting string=w1950:string)  [unwired: 2 in, 1 out]
              n450 = call "Execute query.vi"("String"=w1950, "connection reference"=w1952) -> ("Table"=w1949:string[][], "connection reference 2"=w1948:T1)  [unwired: 6 in, 2 out]
            }
          }
        }
        frame "Quality" {
          n451 = case shown="\"ALL\"" w1964 {
            selector: w1964 -> [_ _ w1980 w1993 w2006]
            tunnel: w1963 -> [_ w1976 w1989 w2002 w2015]
            tunnel: w1962 -> [_ w1975 w1988 w2001 w2014]
            tunnel: w1961 -> [_ _ _ _ _]
            tunnel: [_ w1969 w1982 w1995 w2008] -> w1960
            tunnel: w1959 -> [w1965 w1972 w1985 w1998 w2011]
            tunnel: [w1965 w1968 w1981 w1994 w2007] -> w1958
            frame "False", Default {
            }
            frame "ALL" {
              w1977 = "%Y-%m-%d " ("time format string (%c)")
              n452 = Format Date/Time String(time format string (%c)=w1977, seconds (now)=w1975) -> (date/time string=w1974:string)  [unwired: 1 in]
              n453 = Format Date/Time String(time format string (%c)=w1977, seconds (now)=w1976) -> (date/time string=w1973:string)  [unwired: 1 in]
              n454 = Format Into String(format string="Select DATE,Production_Count,Station_ID,Stack_holder_ID\nfrom Production_COUNT\nWhere DATE between '%s' and '%s' and Stack_holder_ID='%d'\nand Station_ID='%d'" ("string"), w1974, w1973, 4 ("input 3"), 1 ("input 3")) -> (resulting string=w1970:string)  [unwired: 2 in, 1 out]
              n455 = call "Execute query.vi"("String"=w1970, "connection reference"=w1972) -> ("Table"=w1969:string[][], "connection reference 2"=w1968:T1)  [unwired: 6 in, 2 out]
            }
            frame "1" {
              w1990 = "%Y-%m-%d " ("time format string (%c)")
              n456 = Format Date/Time String(time format string (%c)=w1990, seconds (now)=w1989) -> (date/time string=w1986:string)  [unwired: 1 in]
              n457 = Format Date/Time String(time format string (%c)=w1990, seconds (now)=w1988) -> (date/time string=w1987:string)  [unwired: 1 in]
              n458 = Format Into String(format string="Select DATE,Production_Count,Station_ID,Stack_holder_ID\nfrom Production_COUNT\nWhere DATE between '%s' and '%s' and Shift_ID='%s'and Stack_holder_ID='%d'\nand Station_ID='%d'" ("string"), w1987, w1986, w1980, 4 ("input 4"), 1 ("input 4")) -> (resulting string=w1983:string)  [unwired: 2 in, 1 out]
              n459 = call "Execute query.vi"("String"=w1983, "connection reference"=w1985) -> ("Table"=w1982:string[][], "connection reference 2"=w1981:T1)  [unwired: 6 in, 2 out]
            }
            frame "2" {
              w2003 = "%Y-%m-%d " ("time format string (%c)")
              n460 = Format Date/Time String(time format string (%c)=w2003, seconds (now)=w2002) -> (date/time string=w1999:string)  [unwired: 1 in]
              n461 = Format Date/Time String(time format string (%c)=w2003, seconds (now)=w2001) -> (date/time string=w2000:string)  [unwired: 1 in]
              n462 = Format Into String(format string="Select DATE,Production_Count,Station_ID,Stack_holder_ID\nfrom Production_COUNT\nWhere DATE between '%s' and '%s' and Shift_ID='%s'and Stack_holder_ID='%d'\nand Station_ID='%d'" ("string"), w2000, w1999, w1993, 4 ("input 4"), 1 ("input 4")) -> (resulting string=w1996:string)  [unwired: 2 in, 1 out]
              n463 = call "Execute query.vi"("String"=w1996, "connection reference"=w1998) -> ("Table"=w1995:string[][], "connection reference 2"=w1994:T1)  [unwired: 6 in, 2 out]
            }
            frame "3" {
              w2016 = "%Y-%m-%d " ("time format string (%c)")
              n464 = Format Date/Time String(time format string (%c)=w2016, seconds (now)=w2015) -> (date/time string=w2012:string)  [unwired: 1 in]
              n465 = Format Date/Time String(time format string (%c)=w2016, seconds (now)=w2014) -> (date/time string=w2013:string)  [unwired: 1 in]
              n466 = Format Into String(format string="Select DATE,Production_Count,Station_ID,Stack_holder_ID\nfrom Production_COUNT\nWhere DATE between '%s' and '%s' and Shift_ID='%s'and Stack_holder_ID='%d'\nand Station_ID='%d'" ("string"), w2013, w2012, w2006, 4 ("input 4"), 1 ("input 4")) -> (resulting string=w2009:string)  [unwired: 2 in, 1 out]
              n467 = call "Execute query.vi"("String"=w2009, "connection reference"=w2011) -> ("Table"=w2008:string[][], "connection reference 2"=w2007:T1)  [unwired: 6 in, 2 out]
            }
          }
        }
        frame "Production" {
          n468 = case shown="\"False\", Default" w2023 {
            selector: w2023 -> [_ _ w2039 w2052 w2065]
            tunnel: w2022 -> [_ w2035 w2048 w2061 w2074]
            tunnel: w2021 -> [_ w2034 w2047 w2060 w2073]
            tunnel: w2020 -> [_ _ _ _ _]
            tunnel: [_ w2028 w2041 w2054 w2067] -> w2019
            tunnel: w2018 -> [w2024 w2031 w2044 w2057 w2070]
            tunnel: [w2024 w2027 w2040 w2053 w2066] -> w2017
            frame "False", Default {
            }
            frame "ALL" {
              w2036 = "%Y-%m-%d " ("time format string (%c)")
              n469 = Format Date/Time String(time format string (%c)=w2036, seconds (now)=w2034) -> (date/time string=w2033:string)  [unwired: 1 in]
              n470 = Format Date/Time String(time format string (%c)=w2036, seconds (now)=w2035) -> (date/time string=w2032:string)  [unwired: 1 in]
              n471 = Format Into String(format string="Select DATE,Production_Count,Station_ID,Stack_holder_ID\nfrom Production_COUNT\nWhere DATE between '%s' and '%s' and Stack_holder_ID='%d'\nand Station_ID='%d'" ("string"), w2033, w2032, 5 ("input 3"), 1 ("input 3")) -> (resulting string=w2029:string)  [unwired: 2 in, 1 out]
              n472 = call "Execute query.vi"("String"=w2029, "connection reference"=w2031) -> ("Table"=w2028:string[][], "connection reference 2"=w2027:T1)  [unwired: 6 in, 2 out]
            }
            frame "1" {
              w2049 = "%Y-%m-%d " ("time format string (%c)")
              n473 = Format Date/Time String(time format string (%c)=w2049, seconds (now)=w2048) -> (date/time string=w2045:string)  [unwired: 1 in]
              n474 = Format Date/Time String(time format string (%c)=w2049, seconds (now)=w2047) -> (date/time string=w2046:string)  [unwired: 1 in]
              n475 = Format Into String(format string="Select DATE,Production_Count,Station_ID,Stack_holder_ID\nfrom Production_COUNT\nWhere DATE between '%s' and '%s' and Shift_ID='%s'and Stack_holder_ID='%d'\nand Station_ID='%d'" ("string"), w2046, w2045, w2039, 5 ("input 4"), 1 ("input 4")) -> (resulting string=w2042:string)  [unwired: 2 in, 1 out]
              n476 = call "Execute query.vi"("String"=w2042, "connection reference"=w2044) -> ("Table"=w2041:string[][], "connection reference 2"=w2040:T1)  [unwired: 6 in, 2 out]
            }
            frame "2" {
              w2062 = "%Y-%m-%d " ("time format string (%c)")
              n477 = Format Date/Time String(time format string (%c)=w2062, seconds (now)=w2061) -> (date/time string=w2058:string)  [unwired: 1 in]
              n478 = Format Date/Time String(time format string (%c)=w2062, seconds (now)=w2060) -> (date/time string=w2059:string)  [unwired: 1 in]
              n479 = Format Into String(format string="Select DATE,Production_Count,Station_ID,Stack_holder_ID\nfrom Production_COUNT\nWhere DATE between '%s' and '%s' and Shift_ID='%s'and Stack_holder_ID='%d'\nand Station_ID='%d'" ("string"), w2059, w2058, w2052, 5 ("input 4"), 1 ("input 4")) -> (resulting string=w2055:string)  [unwired: 2 in, 1 out]
              n480 = call "Execute query.vi"("String"=w2055, "connection reference"=w2057) -> ("Table"=w2054:string[][], "connection reference 2"=w2053:T1)  [unwired: 6 in, 2 out]
            }
            frame "3" {
              w2075 = "%Y-%m-%d " ("time format string (%c)")
              n481 = Format Date/Time String(time format string (%c)=w2075, seconds (now)=w2074) -> (date/time string=w2071:string)  [unwired: 1 in]
              n482 = Format Date/Time String(time format string (%c)=w2075, seconds (now)=w2073) -> (date/time string=w2072:string)  [unwired: 1 in]
              n483 = Format Into String(format string="Select DATE,Production_Count,Station_ID,Stack_holder_ID\nfrom Production_COUNT\nWhere DATE between '%s' and '%s' and Shift_ID='%s'and Stack_holder_ID='%d'\nand Station_ID='%d'" ("string"), w2072, w2071, w2065, 5 ("input 4"), 1 ("input 4")) -> (resulting string=w2068:string)  [unwired: 2 in, 1 out]
              n484 = call "Execute query.vi"("String"=w2068, "connection reference"=w2070) -> ("Table"=w2067:string[][], "connection reference 2"=w2066:T1)  [unwired: 6 in, 2 out]
            }
          }
        }
      }
    }
    frame "ST 4" {
      n485 = case shown="\"ALL\", Default" w2082 {
        tunnel: w2088 -> [w2100 w2265 w2324 w2380 w2439 w2498]
        tunnel: w2087 -> [w2099 w2264 w2323 w2379 w2438 w2497]
        tunnel: w2086 -> [w2098 w2263 w2322 w2378 w2437 w2496]
        tunnel: w2085 -> [w2097 w2262 w2321 w2377 w2436 w2495]
        tunnel: [w2096 w2261 w2320 w2376 w2435 w2494] -> w2079
        tunnel: w2084 -> [w2095 w2260 w2319 w2375 w2434 w2493]
        tunnel: [w2094 w2259 w2318 w2374 w2433 w2492] -> w2083
        tunnel: w2081 -> [w2093 _ _ _ _ _]
        tunnel: w2080 -> [w2092 _ _ _ _ _]
        tunnel: w2078 -> [w2091 _ _ _ _ _]
        tunnel: w2077 -> [w2090 _ _ _ _ _]
        tunnel: [w2089 _ _ _ _ _] -> w2076
        frame "ALL", Default {
          n486 = case shown="\"ALL\", Default" w2100 {
            selector: w2100 -> [_ w2139 w2179 w2219]
            tunnel: w2099 -> [_ _ _ _]
            tunnel: w2098 -> [_ _ _ _]
            tunnel: w2097 -> [_ _ _ _]
            tunnel: [w2103 w2142 w2182 w2222] -> w2096
            tunnel: w2095 -> [w2109 w2148 w2188 w2228]
            tunnel: [w2108 w2147 w2187 w2227] -> w2094
            tunnel: w2093 -> [w2107 w2146 w2186 w2226]
            tunnel: w2092 -> [w2106 w2145 w2185 w2225]
            tunnel: w2091 -> [w2104 w2143 w2183 w2223]
            tunnel: w2090 -> [w2102 w2141 w2181 w2221]
            tunnel: [w2101 w2140 w2180 w2220] -> w2089
            frame "ALL", Default {
              n487 = for {
                tunnel: w2107 -> [w2121]
                tunnel: w2106 -> [w2120]
                shift-right: [w2123] -> w2108
                shift-left: w2109 -> [w2125]
                shift-right: [w2112] -> w2103
                shift-left: string[][] [] -> [w2114]
                tunnel: w2104 -> [w2115] mode=indexing
                tunnel: w2102 -> [w2111]
                tunnel: [w2110] -> w2101
                n488 = case shown="\"April\"" w2120 {
                  tunnel: ["1" "1" "2" "3" "4" "5" "6" "7" "8" "9" "10" "11" "12"] -> w2119
                  frame "False", Default {
                  }
                  frame "January" {
                  }
                  frame "February" {
                  }
                  frame "March" {
                  }
                  frame "April" {
                  }
                  frame "May" {
                  }
                  frame "June" {
                  }
                  frame "July" {
                  }
                  frame "August" {
                  }
                  frame "September" {
                  }
                  frame "October" {
                  }
                  frame "November" {
                  }
                  frame "December" {
                  }
                }
                n489 = Concatenate Strings("Select DISTINCT PLAN_DATE,PRODUCTION_COUNT,STATION_ID,DATE\nfrom ", w2115, " Where year( PLAN_DATE) ='%s' and month(PLAN_DATE) = '%s' and STATION_ID='%d'") -> (w2116:string)
                n490 = Format Into String(format string=w2116, w2121, w2119, 4 ("input 3")) -> (resulting string=w2124:string)  [unwired: 2 in, 1 out]
                n491 = call "Execute query.vi"("error in (no error)"=w2111, "String"=w2124, "connection reference"=w2125) -> ("error out"=w2110:errorcluster, "Table"=w2113:string[][], "connection reference 2"=w2123:T1)  [unwired: 5 in, 1 out]
                n492 = Build Array (concatenate)(w2114, w2113) -> (w2112:string[][])
              }
            }
            frame "1" {
              n493 = for {
                tunnel: w2146 -> [w2161]
                tunnel: w2145 -> [w2160]
                shift-right: [w2163] -> w2147
                shift-left: w2148 -> [w2165]
                shift-right: [w2152] -> w2142
                shift-left: string[][] [] -> [w2154]
                tunnel: w2143 -> [w2155] mode=indexing
                tunnel: w2141 -> [w2151]
                tunnel: [w2150] -> w2140
                tunnel: w2139 -> [w2149]
                n494 = case shown="\"April\"" w2160 {
                  tunnel: ["1" "1" "2" "3" "4" "5" "6" "7" "8" "9" "10" "11" "12"] -> w2159
                  frame "False", Default {
                  }
                  frame "January" {
                  }
                  frame "February" {
                  }
                  frame "March" {
                  }
                  frame "April" {
                  }
                  frame "May" {
                  }
                  frame "June" {
                  }
                  frame "July" {
                  }
                  frame "August" {
                  }
                  frame "September" {
                  }
                  frame "October" {
                  }
                  frame "November" {
                  }
                  frame "December" {
                  }
                }
                n495 = Concatenate Strings("Select DISTINCT PLAN_DATE,PRODUCTION_COUNT,STATION_ID,DATE\nfrom ", w2155, " Where year( PLAN_DATE) ='%s' and month(PLAN_DATE) = '%s' and STATION_ID='%d' and SHIFT='%s'") -> (w2156:string)
                n496 = Format Into String(format string=w2156, w2161, w2159, 4 ("input 3"), w2149) -> (resulting string=w2164:string)  [unwired: 2 in, 1 out]
                n497 = call "Execute query.vi"("error in (no error)"=w2151, "String"=w2164, "connection reference"=w2165) -> ("error out"=w2150:errorcluster, "Table"=w2153:string[][], "connection reference 2"=w2163:T1)  [unwired: 5 in, 1 out]
                n498 = Build Array (concatenate)(w2154, w2153) -> (w2152:string[][])
              }
            }
            frame "2" {
              n499 = for {
                tunnel: w2186 -> [w2201]
                tunnel: w2185 -> [w2200]
                shift-right: [w2203] -> w2187
                shift-left: w2188 -> [w2205]
                shift-right: [w2192] -> w2182
                shift-left: string[][] [] -> [w2194]
                tunnel: w2183 -> [w2195] mode=indexing
                tunnel: w2181 -> [w2191]
                tunnel: [w2190] -> w2180
                tunnel: w2179 -> [w2189]
                n500 = case shown="\"April\"" w2200 {
                  tunnel: ["1" "1" "2" "3" "4" "5" "6" "7" "8" "9" "10" "11" "12"] -> w2199
                  frame "False", Default {
                  }
                  frame "January" {
                  }
                  frame "February" {
                  }
                  frame "March" {
                  }
                  frame "April" {
                  }
                  frame "May" {
                  }
                  frame "June" {
                  }
                  frame "July" {
                  }
                  frame "August" {
                  }
                  frame "September" {
                  }
                  frame "October" {
                  }
                  frame "November" {
                  }
                  frame "December" {
                  }
                }
                n501 = Concatenate Strings("Select DISTINCT PLAN_DATE,PRODUCTION_COUNT,STATION_ID,DATE\nfrom ", w2195, " Where year( PLAN_DATE) ='%s' and month(PLAN_DATE) = '%s' and STATION_ID='%d' and SHIFT='%s'") -> (w2196:string)
                n502 = Format Into String(format string=w2196, w2201, w2199, 4 ("input 3"), w2189) -> (resulting string=w2204:string)  [unwired: 2 in, 1 out]
                n503 = call "Execute query.vi"("error in (no error)"=w2191, "String"=w2204, "connection reference"=w2205) -> ("error out"=w2190:errorcluster, "Table"=w2193:string[][], "connection reference 2"=w2203:T1)  [unwired: 5 in, 1 out]
                n504 = Build Array (concatenate)(w2194, w2193) -> (w2192:string[][])
              }
            }
            frame "3" {
              n505 = for {
                tunnel: w2226 -> [w2241]
                tunnel: w2225 -> [w2240]
                shift-right: [w2243] -> w2227
                shift-left: w2228 -> [w2245]
                shift-right: [w2232] -> w2222
                shift-left: string[][] [] -> [w2234]
                tunnel: w2223 -> [w2235] mode=indexing
                tunnel: w2221 -> [w2231]
                tunnel: [w2230] -> w2220
                tunnel: w2219 -> [w2229]
                n506 = case shown="\"April\"" w2240 {
                  tunnel: ["1" "1" "2" "3" "4" "5" "6" "7" "8" "9" "10" "11" "12"] -> w2239
                  frame "False", Default {
                  }
                  frame "January" {
                  }
                  frame "February" {
                  }
                  frame "March" {
                  }
                  frame "April" {
                  }
                  frame "May" {
                  }
                  frame "June" {
                  }
                  frame "July" {
                  }
                  frame "August" {
                  }
                  frame "September" {
                  }
                  frame "October" {
                  }
                  frame "November" {
                  }
                  frame "December" {
                  }
                }
                n507 = Concatenate Strings("Select DISTINCT PLAN_DATE,PRODUCTION_COUNT,STATION_ID,DATE\nfrom ", w2235, " Where year( PLAN_DATE) ='%s' and month(PLAN_DATE) = '%s' and STATION_ID='%d' and SHIFT='%s'") -> (w2236:string)
                n508 = Format Into String(format string=w2236, w2241, w2239, 4 ("input 3"), w2229) -> (resulting string=w2244:string)  [unwired: 2 in, 1 out]
                n509 = call "Execute query.vi"("error in (no error)"=w2231, "String"=w2244, "connection reference"=w2245) -> ("error out"=w2230:errorcluster, "Table"=w2233:string[][], "connection reference 2"=w2243:T1)  [unwired: 5 in, 1 out]
                n510 = Build Array (concatenate)(w2234, w2233) -> (w2232:string[][])
              }
            }
          }
        }
        frame "Logistics" {
          n511 = case shown="\"ALL\"" w2265 {
            selector: w2265 -> [_ _ w2281 w2294 w2307]
            tunnel: w2264 -> [_ w2277 w2290 w2303 w2316]
            tunnel: w2263 -> [_ w2276 w2289 w2302 w2315]
            tunnel: w2262 -> [_ _ _ _ _]
            tunnel: [_ w2270 w2283 w2296 w2309] -> w2261
            tunnel: w2260 -> [w2266 w2273 w2286 w2299 w2312]
            tunnel: [w2266 w2269 w2282 w2295 w2308] -> w2259
            frame "False", Default {
            }
            frame "ALL" {
              w2278 = "%Y-%m-%d " ("time format string (%c)")
              n512 = Format Date/Time String(time format string (%c)=w2278, seconds (now)=w2276) -> (date/time string=w2275:string)  [unwired: 1 in]
              n513 = Format Date/Time String(time format string (%c)=w2278, seconds (now)=w2277) -> (date/time string=w2274:string)  [unwired: 1 in]
              n514 = Format Into String(format string="Select DATE,Production_Count,Station_ID,Stack_holder_ID\nfrom Production_COUNT\nWhere DATE between '%s' and '%s' and Stack_holder_ID='%d'\nand Station_ID='%d'" ("string"), w2275, w2274, 2 ("input 3"), 1 ("input 4")) -> (resulting string=w2271:string)  [unwired: 2 in, 1 out]
              n515 = call "Execute query.vi"("String"=w2271, "connection reference"=w2273) -> ("Table"=w2270:string[][], "connection reference 2"=w2269:T1)  [unwired: 6 in, 2 out]
            }
            frame "1" {
              w2291 = "%Y-%m-%d " ("time format string (%c)")
              n516 = Format Date/Time String(time format string (%c)=w2291, seconds (now)=w2290) -> (date/time string=w2287:string)  [unwired: 1 in]
              n517 = Format Date/Time String(time format string (%c)=w2291, seconds (now)=w2289) -> (date/time string=w2288:string)  [unwired: 1 in]
              n518 = Format Into String(format string="Select DATE,Production_Count,Station_ID,Stack_holder_ID\nfrom Production_COUNT\nWhere DATE between '%s' and '%s' and Shift_ID='%s'and Stack_holder_ID='%d'\nand Station_ID='%d'" ("string"), w2288, w2287, w2281, 2 ("input 4"), 1 ("input 4")) -> (resulting string=w2284:string)  [unwired: 2 in, 1 out]
              n519 = call "Execute query.vi"("String"=w2284, "connection reference"=w2286) -> ("Table"=w2283:string[][], "connection reference 2"=w2282:T1)  [unwired: 6 in, 2 out]
            }
            frame "2" {
              w2304 = "%Y-%m-%d " ("time format string (%c)")
              n520 = Format Date/Time String(time format string (%c)=w2304, seconds (now)=w2303) -> (date/time string=w2300:string)  [unwired: 1 in]
              n521 = Format Date/Time String(time format string (%c)=w2304, seconds (now)=w2302) -> (date/time string=w2301:string)  [unwired: 1 in]
              n522 = Format Into String(format string="Select DATE,Production_Count,Station_ID,Stack_holder_ID\nfrom Production_COUNT\nWhere DATE between '%s' and '%s' and Shift_ID='%s'and Stack_holder_ID='%d'\nand Station_ID='%d'" ("string"), w2301, w2300, w2294, 2 ("input 4"), 1 ("input 4")) -> (resulting string=w2297:string)  [unwired: 2 in, 1 out]
              n523 = call "Execute query.vi"("String"=w2297, "connection reference"=w2299) -> ("Table"=w2296:string[][], "connection reference 2"=w2295:T1)  [unwired: 6 in, 2 out]
            }
            frame "3" {
              w2317 = "%Y-%m-%d " ("time format string (%c)")
              n524 = Format Date/Time String(time format string (%c)=w2317, seconds (now)=w2316) -> (date/time string=w2313:string)  [unwired: 1 in]
              n525 = Format Date/Time String(time format string (%c)=w2317, seconds (now)=w2315) -> (date/time string=w2314:string)  [unwired: 1 in]
              n526 = Format Into String(format string="Select DATE,Production_Count,Station_ID,Stack_holder_ID\nfrom Production_COUNT\nWhere DATE between '%s' and '%s' and Shift_ID='%s'and Stack_holder_ID='%d'\nand Station_ID='%d'" ("string"), w2314, w2313, w2307, 2 ("input 4"), 1 ("input 4")) -> (resulting string=w2310:string)  [unwired: 2 in, 1 out]
              n527 = call "Execute query.vi"("String"=w2310, "connection reference"=w2312) -> ("Table"=w2309:string[][], "connection reference 2"=w2308:T1)  [unwired: 6 in, 2 out]
            }
          }
        }
        frame "Gap Leader" {
          n528 = case shown="\"3\"" w2324 {
            selector: w2324 -> [_ _ w2339 w2351 w2363]
            tunnel: w2323 -> [_ w2336 w2348 w2360 w2372]
            tunnel: w2322 -> [_ w2335 w2347 w2359 w2371]
            tunnel: w2321 -> [_ _ _ _ _]
            tunnel: [_ w2329 w2341 w2353 w2365] -> w2320
            tunnel: w2319 -> [w2325 w2332 w2344 w2356 w2368]
            tunnel: [w2325 w2328 w2340 w2352 w2364] -> w2318
            frame "False", Default {
            }
            frame "ALL" {
              w2337 = "%Y-%m-%d " ("time format string (%c)")
              n529 = Format Date/Time String(time format string (%c)=w2337, seconds (now)=w2335) -> (date/time string=w2334:string)  [unwired: 1 in]
              n530 = Format Date/Time String(time format string (%c)=w2337, seconds (now)=w2336) -> (date/time string=w2333:string)  [unwired: 1 in]
              n531 = Format Into String(format string="Select DATE,Production_Count,Station_ID,Stack_holder_ID\nfrom Production_COUNT\nWhere DATE between '%s' and '%s' and Stack_holder_ID='%d'\nand Station_ID='%d'" ("string"), w2334, w2333, 1 ("input 3"), 1 ("input 3")) -> (resulting string=w2330:string)  [unwired: 2 in, 1 out]
              n532 = call "Execute query.vi"("String"=w2330, "connection reference"=w2332) -> ("Table"=w2329:string[][], "connection reference 2"=w2328:T1)  [unwired: 6 in, 2 out]
            }
            frame "1" {
              w2338 = 1 ("input 4")
              w2349 = "%Y-%m-%d " ("time format string (%c)")
              n533 = Format Date/Time String(time format string (%c)=w2349, seconds (now)=w2348) -> (date/time string=w2345:string)  [unwired: 1 in]
              n534 = Format Date/Time String(time format string (%c)=w2349, seconds (now)=w2347) -> (date/time string=w2346:string)  [unwired: 1 in]
              n535 = Format Into String(format string="Select DATE,Production_Count,Station_ID,Stack_holder_ID\nfrom Production_COUNT\nWhere DATE between '%s' and '%s' and Shift_ID='%s'and Stack_holder_ID='%d'\nand Station_ID='%d'" ("string"), w2346, w2345, w2339, w2338, w2338) -> (resulting string=w2342:string)  [unwired: 2 in, 1 out]
              n536 = call "Execute query.vi"("String"=w2342, "connection reference"=w2344) -> ("Table"=w2341:string[][], "connection reference 2"=w2340:T1)  [unwired: 6 in, 2 out]
            }
            frame "2" {
              w2350 = 1 ("input 4")
              w2361 = "%Y-%m-%d " ("time format string (%c)")
              n537 = Format Date/Time String(time format string (%c)=w2361, seconds (now)=w2360) -> (date/time string=w2357:string)  [unwired: 1 in]
              n538 = Format Date/Time String(time format string (%c)=w2361, seconds (now)=w2359) -> (date/time string=w2358:string)  [unwired: 1 in]
              n539 = Format Into String(format string="Select DATE,Production_Count,Station_ID,Stack_holder_ID\nfrom Production_COUNT\nWhere DATE between '%s' and '%s' and Shift_ID='%s'and Stack_holder_ID='%d'\nand Station_ID='%d'" ("string"), w2358, w2357, w2351, w2350, w2350) -> (resulting string=w2354:string)  [unwired: 2 in, 1 out]
              n540 = call "Execute query.vi"("String"=w2354, "connection reference"=w2356) -> ("Table"=w2353:string[][], "connection reference 2"=w2352:T1)  [unwired: 6 in, 2 out]
            }
            frame "3" {
              w2362 = 1 ("input 4")
              w2373 = "%Y-%m-%d " ("time format string (%c)")
              n541 = Format Date/Time String(time format string (%c)=w2373, seconds (now)=w2372) -> (date/time string=w2369:string)  [unwired: 1 in]
              n542 = Format Date/Time String(time format string (%c)=w2373, seconds (now)=w2371) -> (date/time string=w2370:string)  [unwired: 1 in]
              n543 = Format Into String(format string="Select DATE,Production_Count,Station_ID,Stack_holder_ID\nfrom Production_COUNT\nWhere DATE between '%s' and '%s' and Shift_ID='%s'and Stack_holder_ID='%d'\nand Station_ID='%d'" ("string"), w2370, w2369, w2363, w2362, w2362) -> (resulting string=w2366:string)  [unwired: 2 in, 1 out]
              n544 = call "Execute query.vi"("String"=w2366, "connection reference"=w2368) -> ("Table"=w2365:string[][], "connection reference 2"=w2364:T1)  [unwired: 6 in, 2 out]
            }
          }
        }
        frame "Maintenance" {
          n545 = case shown="\"ALL\"" w2380 {
            selector: w2380 -> [_ _ w2396 w2409 w2422]
            tunnel: w2379 -> [_ w2392 w2405 w2418 w2431]
            tunnel: w2378 -> [_ w2391 w2404 w2417 w2430]
            tunnel: w2377 -> [_ _ _ _ _]
            tunnel: [_ w2385 w2398 w2411 w2424] -> w2376
            tunnel: w2375 -> [w2381 w2388 w2401 w2414 w2427]
            tunnel: [w2381 w2384 w2397 w2410 w2423] -> w2374
            frame "False", Default {
            }
            frame "ALL" {
              w2393 = "%Y-%m-%d " ("time format string (%c)")
              n546 = Format Date/Time String(time format string (%c)=w2393, seconds (now)=w2391) -> (date/time string=w2390:string)  [unwired: 1 in]
              n547 = Format Date/Time String(time format string (%c)=w2393, seconds (now)=w2392) -> (date/time string=w2389:string)  [unwired: 1 in]
              n548 = Format Into String(format string="Select DATE,Production_Count,Station_ID,Stack_holder_ID\nfrom Production_COUNT\nWhere DATE between '%s' and '%s' and Stack_holder_ID='%d'\nand Station_ID='%d'" ("string"), w2390, w2389, 3 ("input 3"), 1 ("input 4")) -> (resulting string=w2386:string)  [unwired: 2 in, 1 out]
              n549 = call "Execute query.vi"("String"=w2386, "connection reference"=w2388) -> ("Table"=w2385:string[][], "connection reference 2"=w2384:T1)  [unwired: 6 in, 2 out]
            }
            frame "1" {
              w2406 = "%Y-%m-%d " ("time format string (%c)")
              n550 = Format Date/Time String(time format string (%c)=w2406, seconds (now)=w2405) -> (date/time string=w2402:string)  [unwired: 1 in]
              n551 = Format Date/Time String(time format string (%c)=w2406, seconds (now)=w2404) -> (date/time string=w2403:string)  [unwired: 1 in]
              n552 = Format Into String(format string="Select DATE,Production_Count,Station_ID,Stack_holder_ID\nfrom Production_COUNT\nWhere DATE between '%s' and '%s' and Shift_ID='%s'and Stack_holder_ID='%d'\nand Station_ID='%d'" ("string"), w2403, w2402, w2396, 3 ("input 4"), 1 ("input 5")) -> (resulting string=w2399:string)  [unwired: 2 in, 1 out]
              n553 = call "Execute query.vi"("String"=w2399, "connection reference"=w2401) -> ("Table"=w2398:string[][], "connection reference 2"=w2397:T1)  [unwired: 6 in, 2 out]
            }
            frame "2" {
              w2419 = "%Y-%m-%d " ("time format string (%c)")
              n554 = Format Date/Time String(time format string (%c)=w2419, seconds (now)=w2418) -> (date/time string=w2415:string)  [unwired: 1 in]
              n555 = Format Date/Time String(time format string (%c)=w2419, seconds (now)=w2417) -> (date/time string=w2416:string)  [unwired: 1 in]
              n556 = Format Into String(format string="Select DATE,Production_Count,Station_ID,Stack_holder_ID\nfrom Production_COUNT\nWhere DATE between '%s' and '%s' and Shift_ID='%s'and Stack_holder_ID='%d'\nand Station_ID='%d'" ("string"), w2416, w2415, w2409, 3 ("input 4"), 1 ("input 5")) -> (resulting string=w2412:string)  [unwired: 2 in, 1 out]
              n557 = call "Execute query.vi"("String"=w2412, "connection reference"=w2414) -> ("Table"=w2411:string[][], "connection reference 2"=w2410:T1)  [unwired: 6 in, 2 out]
            }
            frame "3" {
              w2432 = "%Y-%m-%d " ("time format string (%c)")
              n558 = Format Date/Time String(time format string (%c)=w2432, seconds (now)=w2431) -> (date/time string=w2428:string)  [unwired: 1 in]
              n559 = Format Date/Time String(time format string (%c)=w2432, seconds (now)=w2430) -> (date/time string=w2429:string)  [unwired: 1 in]
              n560 = Format Into String(format string="Select DATE,Production_Count,Station_ID,Stack_holder_ID\nfrom Production_COUNT\nWhere DATE between '%s' and '%s' and Shift_ID='%s'and Stack_holder_ID='%d'\nand Station_ID='%d'" ("string"), w2429, w2428, w2422, 3 ("input 4"), 1 ("input 5")) -> (resulting string=w2425:string)  [unwired: 2 in, 1 out]
              n561 = call "Execute query.vi"("String"=w2425, "connection reference"=w2427) -> ("Table"=w2424:string[][], "connection reference 2"=w2423:T1)  [unwired: 6 in, 2 out]
            }
          }
        }
        frame "Quality" {
          n562 = case shown="\"ALL\"" w2439 {
            selector: w2439 -> [_ _ w2455 w2468 w2481]
            tunnel: w2438 -> [_ w2451 w2464 w2477 w2490]
            tunnel: w2437 -> [_ w2450 w2463 w2476 w2489]
            tunnel: w2436 -> [_ _ _ _ _]
            tunnel: [_ w2444 w2457 w2470 w2483] -> w2435
            tunnel: w2434 -> [w2440 w2447 w2460 w2473 w2486]
            tunnel: [w2440 w2443 w2456 w2469 w2482] -> w2433
            frame "False", Default {
            }
            frame "ALL" {
              w2452 = "%Y-%m-%d " ("time format string (%c)")
              n563 = Format Date/Time String(time format string (%c)=w2452, seconds (now)=w2450) -> (date/time string=w2449:string)  [unwired: 1 in]
              n564 = Format Date/Time String(time format string (%c)=w2452, seconds (now)=w2451) -> (date/time string=w2448:string)  [unwired: 1 in]
              n565 = Format Into String(format string="Select DATE,Production_Count,Station_ID,Stack_holder_ID\nfrom Production_COUNT\nWhere DATE between '%s' and '%s' and Stack_holder_ID='%d'\nand Station_ID='%d'" ("string"), w2449, w2448, 4 ("input 3"), 1 ("input 3")) -> (resulting string=w2445:string)  [unwired: 2 in, 1 out]
              n566 = call "Execute query.vi"("String"=w2445, "connection reference"=w2447) -> ("Table"=w2444:string[][], "connection reference 2"=w2443:T1)  [unwired: 6 in, 2 out]
            }
            frame "1" {
              w2465 = "%Y-%m-%d " ("time format string (%c)")
              n567 = Format Date/Time String(time format string (%c)=w2465, seconds (now)=w2464) -> (date/time string=w2461:string)  [unwired: 1 in]
              n568 = Format Date/Time String(time format string (%c)=w2465, seconds (now)=w2463) -> (date/time string=w2462:string)  [unwired: 1 in]
              n569 = Format Into String(format string="Select DATE,Production_Count,Station_ID,Stack_holder_ID\nfrom Production_COUNT\nWhere DATE between '%s' and '%s' and Shift_ID='%s'and Stack_holder_ID='%d'\nand Station_ID='%d'" ("string"), w2462, w2461, w2455, 4 ("input 4"), 1 ("input 4")) -> (resulting string=w2458:string)  [unwired: 2 in, 1 out]
              n570 = call "Execute query.vi"("String"=w2458, "connection reference"=w2460) -> ("Table"=w2457:string[][], "connection reference 2"=w2456:T1)  [unwired: 6 in, 2 out]
            }
            frame "2" {
              w2478 = "%Y-%m-%d " ("time format string (%c)")
              n571 = Format Date/Time String(time format string (%c)=w2478, seconds (now)=w2477) -> (date/time string=w2474:string)  [unwired: 1 in]
              n572 = Format Date/Time String(time format string (%c)=w2478, seconds (now)=w2476) -> (date/time string=w2475:string)  [unwired: 1 in]
              n573 = Format Into String(format string="Select DATE,Production_Count,Station_ID,Stack_holder_ID\nfrom Production_COUNT\nWhere DATE between '%s' and '%s' and Shift_ID='%s'and Stack_holder_ID='%d'\nand Station_ID='%d'" ("string"), w2475, w2474, w2468, 4 ("input 4"), 1 ("input 4")) -> (resulting string=w2471:string)  [unwired: 2 in, 1 out]
              n574 = call "Execute query.vi"("String"=w2471, "connection reference"=w2473) -> ("Table"=w2470:string[][], "connection reference 2"=w2469:T1)  [unwired: 6 in, 2 out]
            }
            frame "3" {
              w2491 = "%Y-%m-%d " ("time format string (%c)")
              n575 = Format Date/Time String(time format string (%c)=w2491, seconds (now)=w2490) -> (date/time string=w2487:string)  [unwired: 1 in]
              n576 = Format Date/Time String(time format string (%c)=w2491, seconds (now)=w2489) -> (date/time string=w2488:string)  [unwired: 1 in]
              n577 = Format Into String(format string="Select DATE,Production_Count,Station_ID,Stack_holder_ID\nfrom Production_COUNT\nWhere DATE between '%s' and '%s' and Shift_ID='%s'and Stack_holder_ID='%d'\nand Station_ID='%d'" ("string"), w2488, w2487, w2481, 4 ("input 4"), 1 ("input 4")) -> (resulting string=w2484:string)  [unwired: 2 in, 1 out]
              n578 = call "Execute query.vi"("String"=w2484, "connection reference"=w2486) -> ("Table"=w2483:string[][], "connection reference 2"=w2482:T1)  [unwired: 6 in, 2 out]
            }
          }
        }
        frame "Production" {
          n579 = case shown="\"False\", Default" w2498 {
            selector: w2498 -> [_ _ w2514 w2527 w2540]
            tunnel: w2497 -> [_ w2510 w2523 w2536 w2549]
            tunnel: w2496 -> [_ w2509 w2522 w2535 w2548]
            tunnel: w2495 -> [_ _ _ _ _]
            tunnel: [_ w2503 w2516 w2529 w2542] -> w2494
            tunnel: w2493 -> [w2499 w2506 w2519 w2532 w2545]
            tunnel: [w2499 w2502 w2515 w2528 w2541] -> w2492
            frame "False", Default {
            }
            frame "ALL" {
              w2511 = "%Y-%m-%d " ("time format string (%c)")
              n580 = Format Date/Time String(time format string (%c)=w2511, seconds (now)=w2509) -> (date/time string=w2508:string)  [unwired: 1 in]
              n581 = Format Date/Time String(time format string (%c)=w2511, seconds (now)=w2510) -> (date/time string=w2507:string)  [unwired: 1 in]
              n582 = Format Into String(format string="Select DATE,Production_Count,Station_ID,Stack_holder_ID\nfrom Production_COUNT\nWhere DATE between '%s' and '%s' and Stack_holder_ID='%d'\nand Station_ID='%d'" ("string"), w2508, w2507, 5 ("input 3"), 1 ("input 3")) -> (resulting string=w2504:string)  [unwired: 2 in, 1 out]
              n583 = call "Execute query.vi"("String"=w2504, "connection reference"=w2506) -> ("Table"=w2503:string[][], "connection reference 2"=w2502:T1)  [unwired: 6 in, 2 out]
            }
            frame "1" {
              w2524 = "%Y-%m-%d " ("time format string (%c)")
              n584 = Format Date/Time String(time format string (%c)=w2524, seconds (now)=w2523) -> (date/time string=w2520:string)  [unwired: 1 in]
              n585 = Format Date/Time String(time format string (%c)=w2524, seconds (now)=w2522) -> (date/time string=w2521:string)  [unwired: 1 in]
              n586 = Format Into String(format string="Select DATE,Production_Count,Station_ID,Stack_holder_ID\nfrom Production_COUNT\nWhere DATE between '%s' and '%s' and Shift_ID='%s'and Stack_holder_ID='%d'\nand Station_ID='%d'" ("string"), w2521, w2520, w2514, 5 ("input 4"), 1 ("input 4")) -> (resulting string=w2517:string)  [unwired: 2 in, 1 out]
              n587 = call "Execute query.vi"("String"=w2517, "connection reference"=w2519) -> ("Table"=w2516:string[][], "connection reference 2"=w2515:T1)  [unwired: 6 in, 2 out]
            }
            frame "2" {
              w2537 = "%Y-%m-%d " ("time format string (%c)")
              n588 = Format Date/Time String(time format string (%c)=w2537, seconds (now)=w2536) -> (date/time string=w2533:string)  [unwired: 1 in]
              n589 = Format Date/Time String(time format string (%c)=w2537, seconds (now)=w2535) -> (date/time string=w2534:string)  [unwired: 1 in]
              n590 = Format Into String(format string="Select DATE,Production_Count,Station_ID,Stack_holder_ID\nfrom Production_COUNT\nWhere DATE between '%s' and '%s' and Shift_ID='%s'and Stack_holder_ID='%d'\nand Station_ID='%d'" ("string"), w2534, w2533, w2527, 5 ("input 4"), 1 ("input 4")) -> (resulting string=w2530:string)  [unwired: 2 in, 1 out]
              n591 = call "Execute query.vi"("String"=w2530, "connection reference"=w2532) -> ("Table"=w2529:string[][], "connection reference 2"=w2528:T1)  [unwired: 6 in, 2 out]
            }
            frame "3" {
              w2550 = "%Y-%m-%d " ("time format string (%c)")
              n592 = Format Date/Time String(time format string (%c)=w2550, seconds (now)=w2549) -> (date/time string=w2546:string)  [unwired: 1 in]
              n593 = Format Date/Time String(time format string (%c)=w2550, seconds (now)=w2548) -> (date/time string=w2547:string)  [unwired: 1 in]
              n594 = Format Into String(format string="Select DATE,Production_Count,Station_ID,Stack_holder_ID\nfrom Production_COUNT\nWhere DATE between '%s' and '%s' and Shift_ID='%s'and Stack_holder_ID='%d'\nand Station_ID='%d'" ("string"), w2547, w2546, w2540, 5 ("input 4"), 1 ("input 4")) -> (resulting string=w2543:string)  [unwired: 2 in, 1 out]
              n595 = call "Execute query.vi"("String"=w2543, "connection reference"=w2545) -> ("Table"=w2542:string[][], "connection reference 2"=w2541:T1)  [unwired: 6 in, 2 out]
            }
          }
        }
      }
    }
    frame "ST 5" {
      n596 = case shown="\"ALL\", Default" w2557 {
        tunnel: w2563 -> [w2575 w2740 w2799 w2855 w2914 w2973]
        tunnel: w2562 -> [w2574 w2739 w2798 w2854 w2913 w2972]
        tunnel: w2561 -> [w2573 w2738 w2797 w2853 w2912 w2971]
        tunnel: w2560 -> [w2572 w2737 w2796 w2852 w2911 w2970]
        tunnel: [w2571 w2736 w2795 w2851 w2910 w2969] -> w2554
        tunnel: w2559 -> [w2570 w2735 w2794 w2850 w2909 w2968]
        tunnel: [w2569 w2734 w2793 w2849 w2908 w2967] -> w2558
        tunnel: w2556 -> [w2568 _ _ _ _ _]
        tunnel: w2555 -> [w2567 _ _ _ _ _]
        tunnel: w2553 -> [w2566 _ _ _ _ _]
        tunnel: w2552 -> [w2565 _ _ _ _ _]
        tunnel: [w2564 _ _ _ _ _] -> w2551
        frame "ALL", Default {
          n597 = case shown="\"3\"" w2575 {
            selector: w2575 -> [_ w2614 w2654 w2694]
            tunnel: w2574 -> [_ _ _ _]
            tunnel: w2573 -> [_ _ _ _]
            tunnel: w2572 -> [_ _ _ _]
            tunnel: [w2578 w2617 w2657 w2697] -> w2571
            tunnel: w2570 -> [w2584 w2623 w2663 w2703]
            tunnel: [w2583 w2622 w2662 w2702] -> w2569
            tunnel: w2568 -> [w2582 w2621 w2661 w2701]
            tunnel: w2567 -> [w2581 w2620 w2660 w2700]
            tunnel: w2566 -> [w2579 w2618 w2658 w2698]
            tunnel: w2565 -> [w2577 w2616 w2656 w2696]
            tunnel: [w2576 w2615 w2655 w2695] -> w2564
            frame "ALL", Default {
              n598 = for {
                tunnel: w2582 -> [w2596]
                tunnel: w2581 -> [w2595]
                shift-right: [w2598] -> w2583
                shift-left: w2584 -> [w2600]
                shift-right: [w2587] -> w2578
                shift-left: string[][] [] -> [w2589]
                tunnel: w2579 -> [w2590] mode=indexing
                tunnel: w2577 -> [w2586]
                tunnel: [w2585] -> w2576
                n599 = case shown="\"April\"" w2595 {
                  tunnel: ["1" "1" "2" "3" "4" "5" "6" "7" "8" "9" "10" "11" "12"] -> w2594
                  frame "False", Default {
                  }
                  frame "January" {
                  }
                  frame "February" {
                  }
                  frame "March" {
                  }
                  frame "April" {
                  }
                  frame "May" {
                  }
                  frame "June" {
                  }
                  frame "July" {
                  }
                  frame "August" {
                  }
                  frame "September" {
                  }
                  frame "October" {
                  }
                  frame "November" {
                  }
                  frame "December" {
                  }
                }
                n600 = Concatenate Strings("Select DISTINCT PLAN_DATE,PRODUCTION_COUNT,STATION_ID,DATE\nfrom ", w2590, " Where year( PLAN_DATE) ='%s' and month(PLAN_DATE) = '%s' and STATION_ID='%d'") -> (w2591:string)
                n601 = Format Into String(format string=w2591, w2596, w2594, 5 ("input 3")) -> (resulting string=w2599:string)  [unwired: 2 in, 1 out]
                n602 = call "Execute query.vi"("error in (no error)"=w2586, "String"=w2599, "connection reference"=w2600) -> ("error out"=w2585:errorcluster, "Table"=w2588:string[][], "connection reference 2"=w2598:T1)  [unwired: 5 in, 1 out]
                n603 = Build Array (concatenate)(w2589, w2588) -> (w2587:string[][])
              }
            }
            frame "1" {
              n604 = for {
                tunnel: w2621 -> [w2636]
                tunnel: w2620 -> [w2635]
                shift-right: [w2638] -> w2622
                shift-left: w2623 -> [w2640]
                shift-right: [w2627] -> w2617
                shift-left: string[][] [] -> [w2629]
                tunnel: w2618 -> [w2630] mode=indexing
                tunnel: w2616 -> [w2626]
                tunnel: [w2625] -> w2615
                tunnel: w2614 -> [w2624]
                n605 = case shown="\"April\"" w2635 {
                  tunnel: ["1" "1" "2" "3" "4" "5" "6" "7" "8" "9" "10" "11" "12"] -> w2634
                  frame "False", Default {
                  }
                  frame "January" {
                  }
                  frame "February" {
                  }
                  frame "March" {
                  }
                  frame "April" {
                  }
                  frame "May" {
                  }
                  frame "June" {
                  }
                  frame "July" {
                  }
                  frame "August" {
                  }
                  frame "September" {
                  }
                  frame "October" {
                  }
                  frame "November" {
                  }
                  frame "December" {
                  }
                }
                n606 = Concatenate Strings("Select DISTINCT PLAN_DATE,PRODUCTION_COUNT,STATION_ID,DATE\nfrom ", w2630, " Where year( PLAN_DATE) ='%s' and month(PLAN_DATE) = '%s' and STATION_ID='%d' and SHIFT='%s'") -> (w2631:string)
                n607 = Format Into String(format string=w2631, w2636, w2634, 5 ("input 3"), w2624) -> (resulting string=w2639:string)  [unwired: 2 in, 1 out]
                n608 = call "Execute query.vi"("error in (no error)"=w2626, "String"=w2639, "connection reference"=w2640) -> ("error out"=w2625:errorcluster, "Table"=w2628:string[][], "connection reference 2"=w2638:T1)  [unwired: 5 in, 1 out]
                n609 = Build Array (concatenate)(w2629, w2628) -> (w2627:string[][])
              }
            }
            frame "2" {
              n610 = for {
                tunnel: w2661 -> [w2676]
                tunnel: w2660 -> [w2675]
                shift-right: [w2678] -> w2662
                shift-left: w2663 -> [w2680]
                shift-right: [w2667] -> w2657
                shift-left: string[][] [] -> [w2669]
                tunnel: w2658 -> [w2670] mode=indexing
                tunnel: w2656 -> [w2666]
                tunnel: [w2665] -> w2655
                tunnel: w2654 -> [w2664]
                n611 = case shown="\"April\"" w2675 {
                  tunnel: ["1" "1" "2" "3" "4" "5" "6" "7" "8" "9" "10" "11" "12"] -> w2674
                  frame "False", Default {
                  }
                  frame "January" {
                  }
                  frame "February" {
                  }
                  frame "March" {
                  }
                  frame "April" {
                  }
                  frame "May" {
                  }
                  frame "June" {
                  }
                  frame "July" {
                  }
                  frame "August" {
                  }
                  frame "September" {
                  }
                  frame "October" {
                  }
                  frame "November" {
                  }
                  frame "December" {
                  }
                }
                n612 = Concatenate Strings("Select DISTINCT PLAN_DATE,PRODUCTION_COUNT,STATION_ID,DATE\nfrom ", w2670, " Where year( PLAN_DATE) ='%s' and month(PLAN_DATE) = '%s' and STATION_ID='%d' and SHIFT='%s'") -> (w2671:string)
                n613 = Format Into String(format string=w2671, w2676, w2674, 5 ("input 3"), w2664) -> (resulting string=w2679:string)  [unwired: 2 in, 1 out]
                n614 = call "Execute query.vi"("error in (no error)"=w2666, "String"=w2679, "connection reference"=w2680) -> ("error out"=w2665:errorcluster, "Table"=w2668:string[][], "connection reference 2"=w2678:T1)  [unwired: 5 in, 1 out]
                n615 = Build Array (concatenate)(w2669, w2668) -> (w2667:string[][])
              }
            }
            frame "3" {
              n616 = for {
                tunnel: w2701 -> [w2716]
                tunnel: w2700 -> [w2715]
                shift-right: [w2718] -> w2702
                shift-left: w2703 -> [w2720]
                shift-right: [w2707] -> w2697
                shift-left: string[][] [] -> [w2709]
                tunnel: w2698 -> [w2710] mode=indexing
                tunnel: w2696 -> [w2706]
                tunnel: [w2705] -> w2695
                tunnel: w2694 -> [w2704]
                n617 = case shown="\"April\"" w2715 {
                  tunnel: ["1" "1" "2" "3" "4" "5" "6" "7" "8" "9" "10" "11" "12"] -> w2714
                  frame "False", Default {
                  }
                  frame "January" {
                  }
                  frame "February" {
                  }
                  frame "March" {
                  }
                  frame "April" {
                  }
                  frame "May" {
                  }
                  frame "June" {
                  }
                  frame "July" {
                  }
                  frame "August" {
                  }
                  frame "September" {
                  }
                  frame "October" {
                  }
                  frame "November" {
                  }
                  frame "December" {
                  }
                }
                n618 = Concatenate Strings("Select DISTINCT PLAN_DATE,PRODUCTION_COUNT,STATION_ID,DATE\nfrom ", w2710, " Where year( PLAN_DATE) ='%s' and month(PLAN_DATE) = '%s' and STATION_ID='%d' and SHIFT='%s'") -> (w2711:string)
                n619 = Format Into String(format string=w2711, w2716, w2714, 5 ("input 3"), w2704) -> (resulting string=w2719:string)  [unwired: 2 in, 1 out]
                n620 = call "Execute query.vi"("error in (no error)"=w2706, "String"=w2719, "connection reference"=w2720) -> ("error out"=w2705:errorcluster, "Table"=w2708:string[][], "connection reference 2"=w2718:T1)  [unwired: 5 in, 1 out]
                n621 = Build Array (concatenate)(w2709, w2708) -> (w2707:string[][])
              }
            }
          }
        }
        frame "Logistics" {
          n622 = case shown="\"ALL\"" w2740 {
            selector: w2740 -> [_ _ w2756 w2769 w2782]
            tunnel: w2739 -> [_ w2752 w2765 w2778 w2791]
            tunnel: w2738 -> [_ w2751 w2764 w2777 w2790]
            tunnel: w2737 -> [_ _ _ _ _]
            tunnel: [_ w2745 w2758 w2771 w2784] -> w2736
            tunnel: w2735 -> [w2741 w2748 w2761 w2774 w2787]
            tunnel: [w2741 w2744 w2757 w2770 w2783] -> w2734
            frame "False", Default {
            }
            frame "ALL" {
              w2753 = "%Y-%m-%d " ("time format string (%c)")
              n623 = Format Date/Time String(time format string (%c)=w2753, seconds (now)=w2751) -> (date/time string=w2750:string)  [unwired: 1 in]
              n624 = Format Date/Time String(time format string (%c)=w2753, seconds (now)=w2752) -> (date/time string=w2749:string)  [unwired: 1 in]
              n625 = Format Into String(format string="Select DATE,Production_Count,Station_ID,Stack_holder_ID\nfrom Production_COUNT\nWhere DATE between '%s' and '%s' and Stack_holder_ID='%d'\nand Station_ID='%d'" ("string"), w2750, w2749, 2 ("input 3"), 1 ("input 4")) -> (resulting string=w2746:string)  [unwired: 2 in, 1 out]
              n626 = call "Execute query.vi"("String"=w2746, "connection reference"=w2748) -> ("Table"=w2745:string[][], "connection reference 2"=w2744:T1)  [unwired: 6 in, 2 out]
            }
            frame "1" {
              w2766 = "%Y-%m-%d " ("time format string (%c)")
              n627 = Format Date/Time String(time format string (%c)=w2766, seconds (now)=w2765) -> (date/time string=w2762:string)  [unwired: 1 in]
              n628 = Format Date/Time String(time format string (%c)=w2766, seconds (now)=w2764) -> (date/time string=w2763:string)  [unwired: 1 in]
              n629 = Format Into String(format string="Select DATE,Production_Count,Station_ID,Stack_holder_ID\nfrom Production_COUNT\nWhere DATE between '%s' and '%s' and Shift_ID='%s'and Stack_holder_ID='%d'\nand Station_ID='%d'" ("string"), w2763, w2762, w2756, 2 ("input 4"), 1 ("input 4")) -> (resulting string=w2759:string)  [unwired: 2 in, 1 out]
              n630 = call "Execute query.vi"("String"=w2759, "connection reference"=w2761) -> ("Table"=w2758:string[][], "connection reference 2"=w2757:T1)  [unwired: 6 in, 2 out]
            }
            frame "2" {
              w2779 = "%Y-%m-%d " ("time format string (%c)")
              n631 = Format Date/Time String(time format string (%c)=w2779, seconds (now)=w2778) -> (date/time string=w2775:string)  [unwired: 1 in]
              n632 = Format Date/Time String(time format string (%c)=w2779, seconds (now)=w2777) -> (date/time string=w2776:string)  [unwired: 1 in]
              n633 = Format Into String(format string="Select DATE,Production_Count,Station_ID,Stack_holder_ID\nfrom Production_COUNT\nWhere DATE between '%s' and '%s' and Shift_ID='%s'and Stack_holder_ID='%d'\nand Station_ID='%d'" ("string"), w2776, w2775, w2769, 2 ("input 4"), 1 ("input 4")) -> (resulting string=w2772:string)  [unwired: 2 in, 1 out]
              n634 = call "Execute query.vi"("String"=w2772, "connection reference"=w2774) -> ("Table"=w2771:string[][], "connection reference 2"=w2770:T1)  [unwired: 6 in, 2 out]
            }
            frame "3" {
              w2792 = "%Y-%m-%d " ("time format string (%c)")
              n635 = Format Date/Time String(time format string (%c)=w2792, seconds (now)=w2791) -> (date/time string=w2788:string)  [unwired: 1 in]
              n636 = Format Date/Time String(time format string (%c)=w2792, seconds (now)=w2790) -> (date/time string=w2789:string)  [unwired: 1 in]
              n637 = Format Into String(format string="Select DATE,Production_Count,Station_ID,Stack_holder_ID\nfrom Production_COUNT\nWhere DATE between '%s' and '%s' and Shift_ID='%s'and Stack_holder_ID='%d'\nand Station_ID='%d'" ("string"), w2789, w2788, w2782, 2 ("input 4"), 1 ("input 4")) -> (resulting string=w2785:string)  [unwired: 2 in, 1 out]
              n638 = call "Execute query.vi"("String"=w2785, "connection reference"=w2787) -> ("Table"=w2784:string[][], "connection reference 2"=w2783:T1)  [unwired: 6 in, 2 out]
            }
          }
        }
        frame "Gap Leader" {
          n639 = case shown="\"3\"" w2799 {
            selector: w2799 -> [_ _ w2814 w2826 w2838]
            tunnel: w2798 -> [_ w2811 w2823 w2835 w2847]
            tunnel: w2797 -> [_ w2810 w2822 w2834 w2846]
            tunnel: w2796 -> [_ _ _ _ _]
            tunnel: [_ w2804 w2816 w2828 w2840] -> w2795
            tunnel: w2794 -> [w2800 w2807 w2819 w2831 w2843]
            tunnel: [w2800 w2803 w2815 w2827 w2839] -> w2793
            frame "False", Default {
            }
            frame "ALL" {
              w2812 = "%Y-%m-%d " ("time format string (%c)")
              n640 = Format Date/Time String(time format string (%c)=w2812, seconds (now)=w2810) -> (date/time string=w2809:string)  [unwired: 1 in]
              n641 = Format Date/Time String(time format string (%c)=w2812, seconds (now)=w2811) -> (date/time string=w2808:string)  [unwired: 1 in]
              n642 = Format Into String(format string="Select DATE,Production_Count,Station_ID,Stack_holder_ID\nfrom Production_COUNT\nWhere DATE between '%s' and '%s' and Stack_holder_ID='%d'\nand Station_ID='%d'" ("string"), w2809, w2808, 1 ("input 3"), 1 ("input 3")) -> (resulting string=w2805:string)  [unwired: 2 in, 1 out]
              n643 = call "Execute query.vi"("String"=w2805, "connection reference"=w2807) -> ("Table"=w2804:string[][], "connection reference 2"=w2803:T1)  [unwired: 6 in, 2 out]
            }
            frame "1" {
              w2813 = 1 ("input 4")
              w2824 = "%Y-%m-%d " ("time format string (%c)")
              n644 = Format Date/Time String(time format string (%c)=w2824, seconds (now)=w2823) -> (date/time string=w2820:string)  [unwired: 1 in]
              n645 = Format Date/Time String(time format string (%c)=w2824, seconds (now)=w2822) -> (date/time string=w2821:string)  [unwired: 1 in]
              n646 = Format Into String(format string="Select DATE,Production_Count,Station_ID,Stack_holder_ID\nfrom Production_COUNT\nWhere DATE between '%s' and '%s' and Shift_ID='%s'and Stack_holder_ID='%d'\nand Station_ID='%d'" ("string"), w2821, w2820, w2814, w2813, w2813) -> (resulting string=w2817:string)  [unwired: 2 in, 1 out]
              n647 = call "Execute query.vi"("String"=w2817, "connection reference"=w2819) -> ("Table"=w2816:string[][], "connection reference 2"=w2815:T1)  [unwired: 6 in, 2 out]
            }
            frame "2" {
              w2825 = 1 ("input 4")
              w2836 = "%Y-%m-%d " ("time format string (%c)")
              n648 = Format Date/Time String(time format string (%c)=w2836, seconds (now)=w2835) -> (date/time string=w2832:string)  [unwired: 1 in]
              n649 = Format Date/Time String(time format string (%c)=w2836, seconds (now)=w2834) -> (date/time string=w2833:string)  [unwired: 1 in]
              n650 = Format Into String(format string="Select DATE,Production_Count,Station_ID,Stack_holder_ID\nfrom Production_COUNT\nWhere DATE between '%s' and '%s' and Shift_ID='%s'and Stack_holder_ID='%d'\nand Station_ID='%d'" ("string"), w2833, w2832, w2826, w2825, w2825) -> (resulting string=w2829:string)  [unwired: 2 in, 1 out]
              n651 = call "Execute query.vi"("String"=w2829, "connection reference"=w2831) -> ("Table"=w2828:string[][], "connection reference 2"=w2827:T1)  [unwired: 6 in, 2 out]
            }
            frame "3" {
              w2837 = 1 ("input 4")
              w2848 = "%Y-%m-%d " ("time format string (%c)")
              n652 = Format Date/Time String(time format string (%c)=w2848, seconds (now)=w2847) -> (date/time string=w2844:string)  [unwired: 1 in]
              n653 = Format Date/Time String(time format string (%c)=w2848, seconds (now)=w2846) -> (date/time string=w2845:string)  [unwired: 1 in]
              n654 = Format Into String(format string="Select DATE,Production_Count,Station_ID,Stack_holder_ID\nfrom Production_COUNT\nWhere DATE between '%s' and '%s' and Shift_ID='%s'and Stack_holder_ID='%d'\nand Station_ID='%d'" ("string"), w2845, w2844, w2838, w2837, w2837) -> (resulting string=w2841:string)  [unwired: 2 in, 1 out]
              n655 = call "Execute query.vi"("String"=w2841, "connection reference"=w2843) -> ("Table"=w2840:string[][], "connection reference 2"=w2839:T1)  [unwired: 6 in, 2 out]
            }
          }
        }
        frame "Maintenance" {
          n656 = case shown="\"ALL\"" w2855 {
            selector: w2855 -> [_ _ w2871 w2884 w2897]
            tunnel: w2854 -> [_ w2867 w2880 w2893 w2906]
            tunnel: w2853 -> [_ w2866 w2879 w2892 w2905]
            tunnel: w2852 -> [_ _ _ _ _]
            tunnel: [_ w2860 w2873 w2886 w2899] -> w2851
            tunnel: w2850 -> [w2856 w2863 w2876 w2889 w2902]
            tunnel: [w2856 w2859 w2872 w2885 w2898] -> w2849
            frame "False", Default {
            }
            frame "ALL" {
              w2868 = "%Y-%m-%d " ("time format string (%c)")
              n657 = Format Date/Time String(time format string (%c)=w2868, seconds (now)=w2866) -> (date/time string=w2865:string)  [unwired: 1 in]
              n658 = Format Date/Time String(time format string (%c)=w2868, seconds (now)=w2867) -> (date/time string=w2864:string)  [unwired: 1 in]
              n659 = Format Into String(format string="Select DATE,Production_Count,Station_ID,Stack_holder_ID\nfrom Production_COUNT\nWhere DATE between '%s' and '%s' and Stack_holder_ID='%d'\nand Station_ID='%d'" ("string"), w2865, w2864, 3 ("input 3"), 1 ("input 4")) -> (resulting string=w2861:string)  [unwired: 2 in, 1 out]
              n660 = call "Execute query.vi"("String"=w2861, "connection reference"=w2863) -> ("Table"=w2860:string[][], "connection reference 2"=w2859:T1)  [unwired: 6 in, 2 out]
            }
            frame "1" {
              w2881 = "%Y-%m-%d " ("time format string (%c)")
              n661 = Format Date/Time String(time format string (%c)=w2881, seconds (now)=w2880) -> (date/time string=w2877:string)  [unwired: 1 in]
              n662 = Format Date/Time String(time format string (%c)=w2881, seconds (now)=w2879) -> (date/time string=w2878:string)  [unwired: 1 in]
              n663 = Format Into String(format string="Select DATE,Production_Count,Station_ID,Stack_holder_ID\nfrom Production_COUNT\nWhere DATE between '%s' and '%s' and Shift_ID='%s'and Stack_holder_ID='%d'\nand Station_ID='%d'" ("string"), w2878, w2877, w2871, 3 ("input 4"), 1 ("input 5")) -> (resulting string=w2874:string)  [unwired: 2 in, 1 out]
              n664 = call "Execute query.vi"("String"=w2874, "connection reference"=w2876) -> ("Table"=w2873:string[][], "connection reference 2"=w2872:T1)  [unwired: 6 in, 2 out]
            }
            frame "2" {
              w2894 = "%Y-%m-%d " ("time format string (%c)")
              n665 = Format Date/Time String(time format string (%c)=w2894, seconds (now)=w2893) -> (date/time string=w2890:string)  [unwired: 1 in]
              n666 = Format Date/Time String(time format string (%c)=w2894, seconds (now)=w2892) -> (date/time string=w2891:string)  [unwired: 1 in]
              n667 = Format Into String(format string="Select DATE,Production_Count,Station_ID,Stack_holder_ID\nfrom Production_COUNT\nWhere DATE between '%s' and '%s' and Shift_ID='%s'and Stack_holder_ID='%d'\nand Station_ID='%d'" ("string"), w2891, w2890, w2884, 3 ("input 4"), 1 ("input 5")) -> (resulting string=w2887:string)  [unwired: 2 in, 1 out]
              n668 = call "Execute query.vi"("String"=w2887, "connection reference"=w2889) -> ("Table"=w2886:string[][], "connection reference 2"=w2885:T1)  [unwired: 6 in, 2 out]
            }
            frame "3" {
              w2907 = "%Y-%m-%d " ("time format string (%c)")
              n669 = Format Date/Time String(time format string (%c)=w2907, seconds (now)=w2906) -> (date/time string=w2903:string)  [unwired: 1 in]
              n670 = Format Date/Time String(time format string (%c)=w2907, seconds (now)=w2905) -> (date/time string=w2904:string)  [unwired: 1 in]
              n671 = Format Into String(format string="Select DATE,Production_Count,Station_ID,Stack_holder_ID\nfrom Production_COUNT\nWhere DATE between '%s' and '%s' and Shift_ID='%s'and Stack_holder_ID='%d'\nand Station_ID='%d'" ("string"), w2904, w2903, w2897, 3 ("input 4"), 1 ("input 5")) -> (resulting string=w2900:string)  [unwired: 2 in, 1 out]
              n672 = call "Execute query.vi"("String"=w2900, "connection reference"=w2902) -> ("Table"=w2899:string[][], "connection reference 2"=w2898:T1)  [unwired: 6 in, 2 out]
            }
          }
        }
        frame "Quality" {
          n673 = case shown="\"ALL\"" w2914 {
            selector: w2914 -> [_ _ w2930 w2943 w2956]
            tunnel: w2913 -> [_ w2926 w2939 w2952 w2965]
            tunnel: w2912 -> [_ w2925 w2938 w2951 w2964]
            tunnel: w2911 -> [_ _ _ _ _]
            tunnel: [_ w2919 w2932 w2945 w2958] -> w2910
            tunnel: w2909 -> [w2915 w2922 w2935 w2948 w2961]
            tunnel: [w2915 w2918 w2931 w2944 w2957] -> w2908
            frame "False", Default {
            }
            frame "ALL" {
              w2927 = "%Y-%m-%d " ("time format string (%c)")
              n674 = Format Date/Time String(time format string (%c)=w2927, seconds (now)=w2925) -> (date/time string=w2924:string)  [unwired: 1 in]
              n675 = Format Date/Time String(time format string (%c)=w2927, seconds (now)=w2926) -> (date/time string=w2923:string)  [unwired: 1 in]
              n676 = Format Into String(format string="Select DATE,Production_Count,Station_ID,Stack_holder_ID\nfrom Production_COUNT\nWhere DATE between '%s' and '%s' and Stack_holder_ID='%d'\nand Station_ID='%d'" ("string"), w2924, w2923, 4 ("input 3"), 1 ("input 3")) -> (resulting string=w2920:string)  [unwired: 2 in, 1 out]
              n677 = call "Execute query.vi"("String"=w2920, "connection reference"=w2922) -> ("Table"=w2919:string[][], "connection reference 2"=w2918:T1)  [unwired: 6 in, 2 out]
            }
            frame "1" {
              w2940 = "%Y-%m-%d " ("time format string (%c)")
              n678 = Format Date/Time String(time format string (%c)=w2940, seconds (now)=w2939) -> (date/time string=w2936:string)  [unwired: 1 in]
              n679 = Format Date/Time String(time format string (%c)=w2940, seconds (now)=w2938) -> (date/time string=w2937:string)  [unwired: 1 in]
              n680 = Format Into String(format string="Select DATE,Production_Count,Station_ID,Stack_holder_ID\nfrom Production_COUNT\nWhere DATE between '%s' and '%s' and Shift_ID='%s'and Stack_holder_ID='%d'\nand Station_ID='%d'" ("string"), w2937, w2936, w2930, 4 ("input 4"), 1 ("input 4")) -> (resulting string=w2933:string)  [unwired: 2 in, 1 out]
              n681 = call "Execute query.vi"("String"=w2933, "connection reference"=w2935) -> ("Table"=w2932:string[][], "connection reference 2"=w2931:T1)  [unwired: 6 in, 2 out]
            }
            frame "2" {
              w2953 = "%Y-%m-%d " ("time format string (%c)")
              n682 = Format Date/Time String(time format string (%c)=w2953, seconds (now)=w2952) -> (date/time string=w2949:string)  [unwired: 1 in]
              n683 = Format Date/Time String(time format string (%c)=w2953, seconds (now)=w2951) -> (date/time string=w2950:string)  [unwired: 1 in]
              n684 = Format Into String(format string="Select DATE,Production_Count,Station_ID,Stack_holder_ID\nfrom Production_COUNT\nWhere DATE between '%s' and '%s' and Shift_ID='%s'and Stack_holder_ID='%d'\nand Station_ID='%d'" ("string"), w2950, w2949, w2943, 4 ("input 4"), 1 ("input 4")) -> (resulting string=w2946:string)  [unwired: 2 in, 1 out]
              n685 = call "Execute query.vi"("String"=w2946, "connection reference"=w2948) -> ("Table"=w2945:string[][], "connection reference 2"=w2944:T1)  [unwired: 6 in, 2 out]
            }
            frame "3" {
              w2966 = "%Y-%m-%d " ("time format string (%c)")
              n686 = Format Date/Time String(time format string (%c)=w2966, seconds (now)=w2965) -> (date/time string=w2962:string)  [unwired: 1 in]
              n687 = Format Date/Time String(time format string (%c)=w2966, seconds (now)=w2964) -> (date/time string=w2963:string)  [unwired: 1 in]
              n688 = Format Into String(format string="Select DATE,Production_Count,Station_ID,Stack_holder_ID\nfrom Production_COUNT\nWhere DATE between '%s' and '%s' and Shift_ID='%s'and Stack_holder_ID='%d'\nand Station_ID='%d'" ("string"), w2963, w2962, w2956, 4 ("input 4"), 1 ("input 4")) -> (resulting string=w2959:string)  [unwired: 2 in, 1 out]
              n689 = call "Execute query.vi"("String"=w2959, "connection reference"=w2961) -> ("Table"=w2958:string[][], "connection reference 2"=w2957:T1)  [unwired: 6 in, 2 out]
            }
          }
        }
        frame "Production" {
          n690 = case shown="\"False\", Default" w2973 {
            selector: w2973 -> [_ _ w2989 w3002 w3015]
            tunnel: w2972 -> [_ w2985 w2998 w3011 w3024]
            tunnel: w2971 -> [_ w2984 w2997 w3010 w3023]
            tunnel: w2970 -> [_ _ _ _ _]
            tunnel: [_ w2978 w2991 w3004 w3017] -> w2969
            tunnel: w2968 -> [w2974 w2981 w2994 w3007 w3020]
            tunnel: [w2974 w2977 w2990 w3003 w3016] -> w2967
            frame "False", Default {
            }
            frame "ALL" {
              w2986 = "%Y-%m-%d " ("time format string (%c)")
              n691 = Format Date/Time String(time format string (%c)=w2986, seconds (now)=w2984) -> (date/time string=w2983:string)  [unwired: 1 in]
              n692 = Format Date/Time String(time format string (%c)=w2986, seconds (now)=w2985) -> (date/time string=w2982:string)  [unwired: 1 in]
              n693 = Format Into String(format string="Select DATE,Production_Count,Station_ID,Stack_holder_ID\nfrom Production_COUNT\nWhere DATE between '%s' and '%s' and Stack_holder_ID='%d'\nand Station_ID='%d'" ("string"), w2983, w2982, 5 ("input 3"), 1 ("input 3")) -> (resulting string=w2979:string)  [unwired: 2 in, 1 out]
              n694 = call "Execute query.vi"("String"=w2979, "connection reference"=w2981) -> ("Table"=w2978:string[][], "connection reference 2"=w2977:T1)  [unwired: 6 in, 2 out]
            }
            frame "1" {
              w2999 = "%Y-%m-%d " ("time format string (%c)")
              n695 = Format Date/Time String(time format string (%c)=w2999, seconds (now)=w2998) -> (date/time string=w2995:string)  [unwired: 1 in]
              n696 = Format Date/Time String(time format string (%c)=w2999, seconds (now)=w2997) -> (date/time string=w2996:string)  [unwired: 1 in]
              n697 = Format Into String(format string="Select DATE,Production_Count,Station_ID,Stack_holder_ID\nfrom Production_COUNT\nWhere DATE between '%s' and '%s' and Shift_ID='%s'and Stack_holder_ID='%d'\nand Station_ID='%d'" ("string"), w2996, w2995, w2989, 5 ("input 4"), 1 ("input 4")) -> (resulting string=w2992:string)  [unwired: 2 in, 1 out]
              n698 = call "Execute query.vi"("String"=w2992, "connection reference"=w2994) -> ("Table"=w2991:string[][], "connection reference 2"=w2990:T1)  [unwired: 6 in, 2 out]
            }
            frame "2" {
              w3012 = "%Y-%m-%d " ("time format string (%c)")
              n699 = Format Date/Time String(time format string (%c)=w3012, seconds (now)=w3011) -> (date/time string=w3008:string)  [unwired: 1 in]
              n700 = Format Date/Time String(time format string (%c)=w3012, seconds (now)=w3010) -> (date/time string=w3009:string)  [unwired: 1 in]
              n701 = Format Into String(format string="Select DATE,Production_Count,Station_ID,Stack_holder_ID\nfrom Production_COUNT\nWhere DATE between '%s' and '%s' and Shift_ID='%s'and Stack_holder_ID='%d'\nand Station_ID='%d'" ("string"), w3009, w3008, w3002, 5 ("input 4"), 1 ("input 4")) -> (resulting string=w3005:string)  [unwired: 2 in, 1 out]
              n702 = call "Execute query.vi"("String"=w3005, "connection reference"=w3007) -> ("Table"=w3004:string[][], "connection reference 2"=w3003:T1)  [unwired: 6 in, 2 out]
            }
            frame "3" {
              w3025 = "%Y-%m-%d " ("time format string (%c)")
              n703 = Format Date/Time String(time format string (%c)=w3025, seconds (now)=w3024) -> (date/time string=w3021:string)  [unwired: 1 in]
              n704 = Format Date/Time String(time format string (%c)=w3025, seconds (now)=w3023) -> (date/time string=w3022:string)  [unwired: 1 in]
              n705 = Format Into String(format string="Select DATE,Production_Count,Station_ID,Stack_holder_ID\nfrom Production_COUNT\nWhere DATE between '%s' and '%s' and Shift_ID='%s'and Stack_holder_ID='%d'\nand Station_ID='%d'" ("string"), w3022, w3021, w3015, 5 ("input 4"), 1 ("input 4")) -> (resulting string=w3018:string)  [unwired: 2 in, 1 out]
              n706 = call "Execute query.vi"("String"=w3018, "connection reference"=w3020) -> ("Table"=w3017:string[][], "connection reference 2"=w3016:T1)  [unwired: 6 in, 2 out]
            }
          }
        }
      }
    }
    frame "ST 6" {
      n707 = case shown="\"ALL\", Default" w3032 {
        tunnel: w3038 -> [w3050 w3215 w3274 w3330 w3389 w3448]
        tunnel: w3037 -> [w3049 w3214 w3273 w3329 w3388 w3447]
        tunnel: w3036 -> [w3048 w3213 w3272 w3328 w3387 w3446]
        tunnel: w3035 -> [w3047 w3212 w3271 w3327 w3386 w3445]
        tunnel: [w3046 w3211 w3270 w3326 w3385 w3444] -> w3029
        tunnel: w3034 -> [w3045 w3210 w3269 w3325 w3384 w3443]
        tunnel: [w3044 w3209 w3268 w3324 w3383 w3442] -> w3033
        tunnel: w3031 -> [w3043 _ _ _ _ _]
        tunnel: w3030 -> [w3042 _ _ _ _ _]
        tunnel: w3028 -> [w3041 _ _ _ _ _]
        tunnel: w3027 -> [w3040 _ _ _ _ _]
        tunnel: [w3039 _ _ _ _ _] -> w3026
        frame "ALL", Default {
          n708 = case shown="\"ALL\", Default" w3050 {
            selector: w3050 -> [_ w3089 w3129 w3169]
            tunnel: w3049 -> [_ _ _ _]
            tunnel: w3048 -> [_ _ _ _]
            tunnel: w3047 -> [_ _ _ _]
            tunnel: [w3053 w3092 w3132 w3172] -> w3046
            tunnel: w3045 -> [w3059 w3098 w3138 w3178]
            tunnel: [w3058 w3097 w3137 w3177] -> w3044
            tunnel: w3043 -> [w3057 w3096 w3136 w3176]
            tunnel: w3042 -> [w3056 w3095 w3135 w3175]
            tunnel: w3041 -> [w3054 w3093 w3133 w3173]
            tunnel: w3040 -> [w3052 w3091 w3131 w3171]
            tunnel: [w3051 w3090 w3130 w3170] -> w3039
            frame "ALL", Default {
              n709 = for {
                tunnel: w3057 -> [w3071]
                tunnel: w3056 -> [w3070]
                shift-right: [w3073] -> w3058
                shift-left: w3059 -> [w3075]
                shift-right: [w3062] -> w3053
                shift-left: string[][] [] -> [w3064]
                tunnel: w3054 -> [w3065] mode=indexing
                tunnel: w3052 -> [w3061]
                tunnel: [w3060] -> w3051
                n710 = case shown="\"April\"" w3070 {
                  tunnel: ["1" "1" "2" "3" "4" "5" "6" "7" "8" "9" "10" "11" "12"] -> w3069
                  frame "False", Default {
                  }
                  frame "January" {
                  }
                  frame "February" {
                  }
                  frame "March" {
                  }
                  frame "April" {
                  }
                  frame "May" {
                  }
                  frame "June" {
                  }
                  frame "July" {
                  }
                  frame "August" {
                  }
                  frame "September" {
                  }
                  frame "October" {
                  }
                  frame "November" {
                  }
                  frame "December" {
                  }
                }
                n711 = Concatenate Strings("Select DISTINCT PLAN_DATE,PRODUCTION_COUNT,STATION_ID,DATE\nfrom ", w3065, " Where year( PLAN_DATE) ='%s' and month(PLAN_DATE) = '%s' and STATION_ID='%d'") -> (w3066:string)
                n712 = Format Into String(format string=w3066, w3071, w3069, 6 ("input 3")) -> (resulting string=w3074:string)  [unwired: 2 in, 1 out]
                n713 = call "Execute query.vi"("error in (no error)"=w3061, "String"=w3074, "connection reference"=w3075) -> ("error out"=w3060:errorcluster, "Table"=w3063:string[][], "connection reference 2"=w3073:T1)  [unwired: 5 in, 1 out]
                n714 = Build Array (concatenate)(w3064, w3063) -> (w3062:string[][])
              }
            }
            frame "1" {
              n715 = for {
                tunnel: w3096 -> [w3111]
                tunnel: w3095 -> [w3110]
                shift-right: [w3113] -> w3097
                shift-left: w3098 -> [w3115]
                shift-right: [w3102] -> w3092
                shift-left: string[][] [] -> [w3104]
                tunnel: w3093 -> [w3105] mode=indexing
                tunnel: w3091 -> [w3101]
                tunnel: [w3100] -> w3090
                tunnel: w3089 -> [w3099]
                n716 = case shown="\"April\"" w3110 {
                  tunnel: ["1" "1" "2" "3" "4" "5" "6" "7" "8" "9" "10" "11" "12"] -> w3109
                  frame "False", Default {
                  }
                  frame "January" {
                  }
                  frame "February" {
                  }
                  frame "March" {
                  }
                  frame "April" {
                  }
                  frame "May" {
                  }
                  frame "June" {
                  }
                  frame "July" {
                  }
                  frame "August" {
                  }
                  frame "September" {
                  }
                  frame "October" {
                  }
                  frame "November" {
                  }
                  frame "December" {
                  }
                }
                n717 = Concatenate Strings("Select DISTINCT PLAN_DATE,PRODUCTION_COUNT,STATION_ID,DATE\nfrom ", w3105, " Where year( PLAN_DATE) ='%s' and month(PLAN_DATE) = '%s' and STATION_ID='%d' and SHIFT='%s'") -> (w3106:string)
                n718 = Format Into String(format string=w3106, w3111, w3109, 6 ("input 3"), w3099) -> (resulting string=w3114:string)  [unwired: 2 in, 1 out]
                n719 = call "Execute query.vi"("error in (no error)"=w3101, "String"=w3114, "connection reference"=w3115) -> ("error out"=w3100:errorcluster, "Table"=w3103:string[][], "connection reference 2"=w3113:T1)  [unwired: 5 in, 1 out]
                n720 = Build Array (concatenate)(w3104, w3103) -> (w3102:string[][])
              }
            }
            frame "2" {
              n721 = for {
                tunnel: w3136 -> [w3151]
                tunnel: w3135 -> [w3150]
                shift-right: [w3153] -> w3137
                shift-left: w3138 -> [w3155]
                shift-right: [w3142] -> w3132
                shift-left: string[][] [] -> [w3144]
                tunnel: w3133 -> [w3145] mode=indexing
                tunnel: w3131 -> [w3141]
                tunnel: [w3140] -> w3130
                tunnel: w3129 -> [w3139]
                n722 = case shown="\"April\"" w3150 {
                  tunnel: ["1" "1" "2" "3" "4" "5" "6" "7" "8" "9" "10" "11" "12"] -> w3149
                  frame "False", Default {
                  }
                  frame "January" {
                  }
                  frame "February" {
                  }
                  frame "March" {
                  }
                  frame "April" {
                  }
                  frame "May" {
                  }
                  frame "June" {
                  }
                  frame "July" {
                  }
                  frame "August" {
                  }
                  frame "September" {
                  }
                  frame "October" {
                  }
                  frame "November" {
                  }
                  frame "December" {
                  }
                }
                n723 = Concatenate Strings("Select DISTINCT PLAN_DATE,PRODUCTION_COUNT,STATION_ID,DATE\nfrom ", w3145, " Where year( PLAN_DATE) ='%s' and month(PLAN_DATE) = '%s' and STATION_ID='%d' and SHIFT='%s'") -> (w3146:string)
                n724 = Format Into String(format string=w3146, w3151, w3149, 6 ("input 3"), w3139) -> (resulting string=w3154:string)  [unwired: 2 in, 1 out]
                n725 = call "Execute query.vi"("error in (no error)"=w3141, "String"=w3154, "connection reference"=w3155) -> ("error out"=w3140:errorcluster, "Table"=w3143:string[][], "connection reference 2"=w3153:T1)  [unwired: 5 in, 1 out]
                n726 = Build Array (concatenate)(w3144, w3143) -> (w3142:string[][])
              }
            }
            frame "3" {
              n727 = for {
                tunnel: w3176 -> [w3191]
                tunnel: w3175 -> [w3190]
                shift-right: [w3193] -> w3177
                shift-left: w3178 -> [w3195]
                shift-right: [w3182] -> w3172
                shift-left: string[][] [] -> [w3184]
                tunnel: w3173 -> [w3185] mode=indexing
                tunnel: w3171 -> [w3181]
                tunnel: [w3180] -> w3170
                tunnel: w3169 -> [w3179]
                n728 = case shown="\"April\"" w3190 {
                  tunnel: ["1" "1" "2" "3" "4" "5" "6" "7" "8" "9" "10" "11" "12"] -> w3189
                  frame "False", Default {
                  }
                  frame "January" {
                  }
                  frame "February" {
                  }
                  frame "March" {
                  }
                  frame "April" {
                  }
                  frame "May" {
                  }
                  frame "June" {
                  }
                  frame "July" {
                  }
                  frame "August" {
                  }
                  frame "September" {
                  }
                  frame "October" {
                  }
                  frame "November" {
                  }
                  frame "December" {
                  }
                }
                n729 = Concatenate Strings("Select DISTINCT PLAN_DATE,PRODUCTION_COUNT,STATION_ID,DATE\nfrom ", w3185, " Where year( PLAN_DATE) ='%s' and month(PLAN_DATE) = '%s' and STATION_ID='%d' and SHIFT='%s'") -> (w3186:string)
                n730 = Format Into String(format string=w3186, w3191, w3189, 6 ("input 3"), w3179) -> (resulting string=w3194:string)  [unwired: 2 in, 1 out]
                n731 = call "Execute query.vi"("error in (no error)"=w3181, "String"=w3194, "connection reference"=w3195) -> ("error out"=w3180:errorcluster, "Table"=w3183:string[][], "connection reference 2"=w3193:T1)  [unwired: 5 in, 1 out]
                n732 = Build Array (concatenate)(w3184, w3183) -> (w3182:string[][])
              }
            }
          }
        }
        frame "Logistics" {
          n733 = case shown="\"ALL\"" w3215 {
            selector: w3215 -> [_ _ w3231 w3244 w3257]
            tunnel: w3214 -> [_ w3227 w3240 w3253 w3266]
            tunnel: w3213 -> [_ w3226 w3239 w3252 w3265]
            tunnel: w3212 -> [_ _ _ _ _]
            tunnel: [_ w3220 w3233 w3246 w3259] -> w3211
            tunnel: w3210 -> [w3216 w3223 w3236 w3249 w3262]
            tunnel: [w3216 w3219 w3232 w3245 w3258] -> w3209
            frame "False", Default {
            }
            frame "ALL" {
              w3228 = "%Y-%m-%d " ("time format string (%c)")
              n734 = Format Date/Time String(time format string (%c)=w3228, seconds (now)=w3226) -> (date/time string=w3225:string)  [unwired: 1 in]
              n735 = Format Date/Time String(time format string (%c)=w3228, seconds (now)=w3227) -> (date/time string=w3224:string)  [unwired: 1 in]
              n736 = Format Into String(format string="Select DATE,Production_Count,Station_ID,Stack_holder_ID\nfrom Production_COUNT\nWhere DATE between '%s' and '%s' and Stack_holder_ID='%d'\nand Station_ID='%d'" ("string"), w3225, w3224, 2 ("input 3"), 1 ("input 4")) -> (resulting string=w3221:string)  [unwired: 2 in, 1 out]
              n737 = call "Execute query.vi"("String"=w3221, "connection reference"=w3223) -> ("Table"=w3220:string[][], "connection reference 2"=w3219:T1)  [unwired: 6 in, 2 out]
            }
            frame "1" {
              w3241 = "%Y-%m-%d " ("time format string (%c)")
              n738 = Format Date/Time String(time format string (%c)=w3241, seconds (now)=w3240) -> (date/time string=w3237:string)  [unwired: 1 in]
              n739 = Format Date/Time String(time format string (%c)=w3241, seconds (now)=w3239) -> (date/time string=w3238:string)  [unwired: 1 in]
              n740 = Format Into String(format string="Select DATE,Production_Count,Station_ID,Stack_holder_ID\nfrom Production_COUNT\nWhere DATE between '%s' and '%s' and Shift_ID='%s'and Stack_holder_ID='%d'\nand Station_ID='%d'" ("string"), w3238, w3237, w3231, 2 ("input 4"), 1 ("input 4")) -> (resulting string=w3234:string)  [unwired: 2 in, 1 out]
              n741 = call "Execute query.vi"("String"=w3234, "connection reference"=w3236) -> ("Table"=w3233:string[][], "connection reference 2"=w3232:T1)  [unwired: 6 in, 2 out]
            }
            frame "2" {
              w3254 = "%Y-%m-%d " ("time format string (%c)")
              n742 = Format Date/Time String(time format string (%c)=w3254, seconds (now)=w3253) -> (date/time string=w3250:string)  [unwired: 1 in]
              n743 = Format Date/Time String(time format string (%c)=w3254, seconds (now)=w3252) -> (date/time string=w3251:string)  [unwired: 1 in]
              n744 = Format Into String(format string="Select DATE,Production_Count,Station_ID,Stack_holder_ID\nfrom Production_COUNT\nWhere DATE between '%s' and '%s' and Shift_ID='%s'and Stack_holder_ID='%d'\nand Station_ID='%d'" ("string"), w3251, w3250, w3244, 2 ("input 4"), 1 ("input 4")) -> (resulting string=w3247:string)  [unwired: 2 in, 1 out]
              n745 = call "Execute query.vi"("String"=w3247, "connection reference"=w3249) -> ("Table"=w3246:string[][], "connection reference 2"=w3245:T1)  [unwired: 6 in, 2 out]
            }
            frame "3" {
              w3267 = "%Y-%m-%d " ("time format string (%c)")
              n746 = Format Date/Time String(time format string (%c)=w3267, seconds (now)=w3266) -> (date/time string=w3263:string)  [unwired: 1 in]
              n747 = Format Date/Time String(time format string (%c)=w3267, seconds (now)=w3265) -> (date/time string=w3264:string)  [unwired: 1 in]
              n748 = Format Into String(format string="Select DATE,Production_Count,Station_ID,Stack_holder_ID\nfrom Production_COUNT\nWhere DATE between '%s' and '%s' and Shift_ID='%s'and Stack_holder_ID='%d'\nand Station_ID='%d'" ("string"), w3264, w3263, w3257, 2 ("input 4"), 1 ("input 4")) -> (resulting string=w3260:string)  [unwired: 2 in, 1 out]
              n749 = call "Execute query.vi"("String"=w3260, "connection reference"=w3262) -> ("Table"=w3259:string[][], "connection reference 2"=w3258:T1)  [unwired: 6 in, 2 out]
            }
          }
        }
        frame "Gap Leader" {
          n750 = case shown="\"3\"" w3274 {
            selector: w3274 -> [_ _ w3289 w3301 w3313]
            tunnel: w3273 -> [_ w3286 w3298 w3310 w3322]
            tunnel: w3272 -> [_ w3285 w3297 w3309 w3321]
            tunnel: w3271 -> [_ _ _ _ _]
            tunnel: [_ w3279 w3291 w3303 w3315] -> w3270
            tunnel: w3269 -> [w3275 w3282 w3294 w3306 w3318]
            tunnel: [w3275 w3278 w3290 w3302 w3314] -> w3268
            frame "False", Default {
            }
            frame "ALL" {
              w3287 = "%Y-%m-%d " ("time format string (%c)")
              n751 = Format Date/Time String(time format string (%c)=w3287, seconds (now)=w3285) -> (date/time string=w3284:string)  [unwired: 1 in]
              n752 = Format Date/Time String(time format string (%c)=w3287, seconds (now)=w3286) -> (date/time string=w3283:string)  [unwired: 1 in]
              n753 = Format Into String(format string="Select DATE,Production_Count,Station_ID,Stack_holder_ID\nfrom Production_COUNT\nWhere DATE between '%s' and '%s' and Stack_holder_ID='%d'\nand Station_ID='%d'" ("string"), w3284, w3283, 1 ("input 3"), 1 ("input 3")) -> (resulting string=w3280:string)  [unwired: 2 in, 1 out]
              n754 = call "Execute query.vi"("String"=w3280, "connection reference"=w3282) -> ("Table"=w3279:string[][], "connection reference 2"=w3278:T1)  [unwired: 6 in, 2 out]
            }
            frame "1" {
              w3288 = 1 ("input 4")
              w3299 = "%Y-%m-%d " ("time format string (%c)")
              n755 = Format Date/Time String(time format string (%c)=w3299, seconds (now)=w3298) -> (date/time string=w3295:string)  [unwired: 1 in]
              n756 = Format Date/Time String(time format string (%c)=w3299, seconds (now)=w3297) -> (date/time string=w3296:string)  [unwired: 1 in]
              n757 = Format Into String(format string="Select DATE,Production_Count,Station_ID,Stack_holder_ID\nfrom Production_COUNT\nWhere DATE between '%s' and '%s' and Shift_ID='%s'and Stack_holder_ID='%d'\nand Station_ID='%d'" ("string"), w3296, w3295, w3289, w3288, w3288) -> (resulting string=w3292:string)  [unwired: 2 in, 1 out]
              n758 = call "Execute query.vi"("String"=w3292, "connection reference"=w3294) -> ("Table"=w3291:string[][], "connection reference 2"=w3290:T1)  [unwired: 6 in, 2 out]
            }
            frame "2" {
              w3300 = 1 ("input 4")
              w3311 = "%Y-%m-%d " ("time format string (%c)")
              n759 = Format Date/Time String(time format string (%c)=w3311, seconds (now)=w3310) -> (date/time string=w3307:string)  [unwired: 1 in]
              n760 = Format Date/Time String(time format string (%c)=w3311, seconds (now)=w3309) -> (date/time string=w3308:string)  [unwired: 1 in]
              n761 = Format Into String(format string="Select DATE,Production_Count,Station_ID,Stack_holder_ID\nfrom Production_COUNT\nWhere DATE between '%s' and '%s' and Shift_ID='%s'and Stack_holder_ID='%d'\nand Station_ID='%d'" ("string"), w3308, w3307, w3301, w3300, w3300) -> (resulting string=w3304:string)  [unwired: 2 in, 1 out]
              n762 = call "Execute query.vi"("String"=w3304, "connection reference"=w3306) -> ("Table"=w3303:string[][], "connection reference 2"=w3302:T1)  [unwired: 6 in, 2 out]
            }
            frame "3" {
              w3312 = 1 ("input 4")
              w3323 = "%Y-%m-%d " ("time format string (%c)")
              n763 = Format Date/Time String(time format string (%c)=w3323, seconds (now)=w3322) -> (date/time string=w3319:string)  [unwired: 1 in]
              n764 = Format Date/Time String(time format string (%c)=w3323, seconds (now)=w3321) -> (date/time string=w3320:string)  [unwired: 1 in]
              n765 = Format Into String(format string="Select DATE,Production_Count,Station_ID,Stack_holder_ID\nfrom Production_COUNT\nWhere DATE between '%s' and '%s' and Shift_ID='%s'and Stack_holder_ID='%d'\nand Station_ID='%d'" ("string"), w3320, w3319, w3313, w3312, w3312) -> (resulting string=w3316:string)  [unwired: 2 in, 1 out]
              n766 = call "Execute query.vi"("String"=w3316, "connection reference"=w3318) -> ("Table"=w3315:string[][], "connection reference 2"=w3314:T1)  [unwired: 6 in, 2 out]
            }
          }
        }
        frame "Maintenance" {
          n767 = case shown="\"ALL\"" w3330 {
            selector: w3330 -> [_ _ w3346 w3359 w3372]
            tunnel: w3329 -> [_ w3342 w3355 w3368 w3381]
            tunnel: w3328 -> [_ w3341 w3354 w3367 w3380]
            tunnel: w3327 -> [_ _ _ _ _]
            tunnel: [_ w3335 w3348 w3361 w3374] -> w3326
            tunnel: w3325 -> [w3331 w3338 w3351 w3364 w3377]
            tunnel: [w3331 w3334 w3347 w3360 w3373] -> w3324
            frame "False", Default {
            }
            frame "ALL" {
              w3343 = "%Y-%m-%d " ("time format string (%c)")
              n768 = Format Date/Time String(time format string (%c)=w3343, seconds (now)=w3341) -> (date/time string=w3340:string)  [unwired: 1 in]
              n769 = Format Date/Time String(time format string (%c)=w3343, seconds (now)=w3342) -> (date/time string=w3339:string)  [unwired: 1 in]
              n770 = Format Into String(format string="Select DATE,Production_Count,Station_ID,Stack_holder_ID\nfrom Production_COUNT\nWhere DATE between '%s' and '%s' and Stack_holder_ID='%d'\nand Station_ID='%d'" ("string"), w3340, w3339, 3 ("input 3"), 1 ("input 4")) -> (resulting string=w3336:string)  [unwired: 2 in, 1 out]
              n771 = call "Execute query.vi"("String"=w3336, "connection reference"=w3338) -> ("Table"=w3335:string[][], "connection reference 2"=w3334:T1)  [unwired: 6 in, 2 out]
            }
            frame "1" {
              w3356 = "%Y-%m-%d " ("time format string (%c)")
              n772 = Format Date/Time String(time format string (%c)=w3356, seconds (now)=w3355) -> (date/time string=w3352:string)  [unwired: 1 in]
              n773 = Format Date/Time String(time format string (%c)=w3356, seconds (now)=w3354) -> (date/time string=w3353:string)  [unwired: 1 in]
              n774 = Format Into String(format string="Select DATE,Production_Count,Station_ID,Stack_holder_ID\nfrom Production_COUNT\nWhere DATE between '%s' and '%s' and Shift_ID='%s'and Stack_holder_ID='%d'\nand Station_ID='%d'" ("string"), w3353, w3352, w3346, 3 ("input 4"), 1 ("input 5")) -> (resulting string=w3349:string)  [unwired: 2 in, 1 out]
              n775 = call "Execute query.vi"("String"=w3349, "connection reference"=w3351) -> ("Table"=w3348:string[][], "connection reference 2"=w3347:T1)  [unwired: 6 in, 2 out]
            }
            frame "2" {
              w3369 = "%Y-%m-%d " ("time format string (%c)")
              n776 = Format Date/Time String(time format string (%c)=w3369, seconds (now)=w3368) -> (date/time string=w3365:string)  [unwired: 1 in]
              n777 = Format Date/Time String(time format string (%c)=w3369, seconds (now)=w3367) -> (date/time string=w3366:string)  [unwired: 1 in]
              n778 = Format Into String(format string="Select DATE,Production_Count,Station_ID,Stack_holder_ID\nfrom Production_COUNT\nWhere DATE between '%s' and '%s' and Shift_ID='%s'and Stack_holder_ID='%d'\nand Station_ID='%d'" ("string"), w3366, w3365, w3359, 3 ("input 4"), 1 ("input 5")) -> (resulting string=w3362:string)  [unwired: 2 in, 1 out]
              n779 = call "Execute query.vi"("String"=w3362, "connection reference"=w3364) -> ("Table"=w3361:string[][], "connection reference 2"=w3360:T1)  [unwired: 6 in, 2 out]
            }
            frame "3" {
              w3382 = "%Y-%m-%d " ("time format string (%c)")
              n780 = Format Date/Time String(time format string (%c)=w3382, seconds (now)=w3381) -> (date/time string=w3378:string)  [unwired: 1 in]
              n781 = Format Date/Time String(time format string (%c)=w3382, seconds (now)=w3380) -> (date/time string=w3379:string)  [unwired: 1 in]
              n782 = Format Into String(format string="Select DATE,Production_Count,Station_ID,Stack_holder_ID\nfrom Production_COUNT\nWhere DATE between '%s' and '%s' and Shift_ID='%s'and Stack_holder_ID='%d'\nand Station_ID='%d'" ("string"), w3379, w3378, w3372, 3 ("input 4"), 1 ("input 5")) -> (resulting string=w3375:string)  [unwired: 2 in, 1 out]
              n783 = call "Execute query.vi"("String"=w3375, "connection reference"=w3377) -> ("Table"=w3374:string[][], "connection reference 2"=w3373:T1)  [unwired: 6 in, 2 out]
            }
          }
        }
        frame "Quality" {
          n784 = case shown="\"ALL\"" w3389 {
            selector: w3389 -> [_ _ w3405 w3418 w3431]
            tunnel: w3388 -> [_ w3401 w3414 w3427 w3440]
            tunnel: w3387 -> [_ w3400 w3413 w3426 w3439]
            tunnel: w3386 -> [_ _ _ _ _]
            tunnel: [_ w3394 w3407 w3420 w3433] -> w3385
            tunnel: w3384 -> [w3390 w3397 w3410 w3423 w3436]
            tunnel: [w3390 w3393 w3406 w3419 w3432] -> w3383
            frame "False", Default {
            }
            frame "ALL" {
              w3402 = "%Y-%m-%d " ("time format string (%c)")
              n785 = Format Date/Time String(time format string (%c)=w3402, seconds (now)=w3400) -> (date/time string=w3399:string)  [unwired: 1 in]
              n786 = Format Date/Time String(time format string (%c)=w3402, seconds (now)=w3401) -> (date/time string=w3398:string)  [unwired: 1 in]
              n787 = Format Into String(format string="Select DATE,Production_Count,Station_ID,Stack_holder_ID\nfrom Production_COUNT\nWhere DATE between '%s' and '%s' and Stack_holder_ID='%d'\nand Station_ID='%d'" ("string"), w3399, w3398, 4 ("input 3"), 1 ("input 3")) -> (resulting string=w3395:string)  [unwired: 2 in, 1 out]
              n788 = call "Execute query.vi"("String"=w3395, "connection reference"=w3397) -> ("Table"=w3394:string[][], "connection reference 2"=w3393:T1)  [unwired: 6 in, 2 out]
            }
            frame "1" {
              w3415 = "%Y-%m-%d " ("time format string (%c)")
              n789 = Format Date/Time String(time format string (%c)=w3415, seconds (now)=w3414) -> (date/time string=w3411:string)  [unwired: 1 in]
              n790 = Format Date/Time String(time format string (%c)=w3415, seconds (now)=w3413) -> (date/time string=w3412:string)  [unwired: 1 in]
              n791 = Format Into String(format string="Select DATE,Production_Count,Station_ID,Stack_holder_ID\nfrom Production_COUNT\nWhere DATE between '%s' and '%s' and Shift_ID='%s'and Stack_holder_ID='%d'\nand Station_ID='%d'" ("string"), w3412, w3411, w3405, 4 ("input 4"), 1 ("input 4")) -> (resulting string=w3408:string)  [unwired: 2 in, 1 out]
              n792 = call "Execute query.vi"("String"=w3408, "connection reference"=w3410) -> ("Table"=w3407:string[][], "connection reference 2"=w3406:T1)  [unwired: 6 in, 2 out]
            }
            frame "2" {
              w3428 = "%Y-%m-%d " ("time format string (%c)")
              n793 = Format Date/Time String(time format string (%c)=w3428, seconds (now)=w3427) -> (date/time string=w3424:string)  [unwired: 1 in]
              n794 = Format Date/Time String(time format string (%c)=w3428, seconds (now)=w3426) -> (date/time string=w3425:string)  [unwired: 1 in]
              n795 = Format Into String(format string="Select DATE,Production_Count,Station_ID,Stack_holder_ID\nfrom Production_COUNT\nWhere DATE between '%s' and '%s' and Shift_ID='%s'and Stack_holder_ID='%d'\nand Station_ID='%d'" ("string"), w3425, w3424, w3418, 4 ("input 4"), 1 ("input 4")) -> (resulting string=w3421:string)  [unwired: 2 in, 1 out]
              n796 = call "Execute query.vi"("String"=w3421, "connection reference"=w3423) -> ("Table"=w3420:string[][], "connection reference 2"=w3419:T1)  [unwired: 6 in, 2 out]
            }
            frame "3" {
              w3441 = "%Y-%m-%d " ("time format string (%c)")
              n797 = Format Date/Time String(time format string (%c)=w3441, seconds (now)=w3440) -> (date/time string=w3437:string)  [unwired: 1 in]
              n798 = Format Date/Time String(time format string (%c)=w3441, seconds (now)=w3439) -> (date/time string=w3438:string)  [unwired: 1 in]
              n799 = Format Into String(format string="Select DATE,Production_Count,Station_ID,Stack_holder_ID\nfrom Production_COUNT\nWhere DATE between '%s' and '%s' and Shift_ID='%s'and Stack_holder_ID='%d'\nand Station_ID='%d'" ("string"), w3438, w3437, w3431, 4 ("input 4"), 1 ("input 4")) -> (resulting string=w3434:string)  [unwired: 2 in, 1 out]
              n800 = call "Execute query.vi"("String"=w3434, "connection reference"=w3436) -> ("Table"=w3433:string[][], "connection reference 2"=w3432:T1)  [unwired: 6 in, 2 out]
            }
          }
        }
        frame "Production" {
          n801 = case shown="\"False\", Default" w3448 {
            selector: w3448 -> [_ _ w3464 w3477 w3490]
            tunnel: w3447 -> [_ w3460 w3473 w3486 w3499]
            tunnel: w3446 -> [_ w3459 w3472 w3485 w3498]
            tunnel: w3445 -> [_ _ _ _ _]
            tunnel: [_ w3453 w3466 w3479 w3492] -> w3444
            tunnel: w3443 -> [w3449 w3456 w3469 w3482 w3495]
            tunnel: [w3449 w3452 w3465 w3478 w3491] -> w3442
            frame "False", Default {
            }
            frame "ALL" {
              w3461 = "%Y-%m-%d " ("time format string (%c)")
              n802 = Format Date/Time String(time format string (%c)=w3461, seconds (now)=w3459) -> (date/time string=w3458:string)  [unwired: 1 in]
              n803 = Format Date/Time String(time format string (%c)=w3461, seconds (now)=w3460) -> (date/time string=w3457:string)  [unwired: 1 in]
              n804 = Format Into String(format string="Select DATE,Production_Count,Station_ID,Stack_holder_ID\nfrom Production_COUNT\nWhere DATE between '%s' and '%s' and Stack_holder_ID='%d'\nand Station_ID='%d'" ("string"), w3458, w3457, 5 ("input 3"), 1 ("input 3")) -> (resulting string=w3454:string)  [unwired: 2 in, 1 out]
              n805 = call "Execute query.vi"("String"=w3454, "connection reference"=w3456) -> ("Table"=w3453:string[][], "connection reference 2"=w3452:T1)  [unwired: 6 in, 2 out]
            }
            frame "1" {
              w3474 = "%Y-%m-%d " ("time format string (%c)")
              n806 = Format Date/Time String(time format string (%c)=w3474, seconds (now)=w3473) -> (date/time string=w3470:string)  [unwired: 1 in]
              n807 = Format Date/Time String(time format string (%c)=w3474, seconds (now)=w3472) -> (date/time string=w3471:string)  [unwired: 1 in]
              n808 = Format Into String(format string="Select DATE,Production_Count,Station_ID,Stack_holder_ID\nfrom Production_COUNT\nWhere DATE between '%s' and '%s' and Shift_ID='%s'and Stack_holder_ID='%d'\nand Station_ID='%d'" ("string"), w3471, w3470, w3464, 5 ("input 4"), 1 ("input 4")) -> (resulting string=w3467:string)  [unwired: 2 in, 1 out]
              n809 = call "Execute query.vi"("String"=w3467, "connection reference"=w3469) -> ("Table"=w3466:string[][], "connection reference 2"=w3465:T1)  [unwired: 6 in, 2 out]
            }
            frame "2" {
              w3487 = "%Y-%m-%d " ("time format string (%c)")
              n810 = Format Date/Time String(time format string (%c)=w3487, seconds (now)=w3486) -> (date/time string=w3483:string)  [unwired: 1 in]
              n811 = Format Date/Time String(time format string (%c)=w3487, seconds (now)=w3485) -> (date/time string=w3484:string)  [unwired: 1 in]
              n812 = Format Into String(format string="Select DATE,Production_Count,Station_ID,Stack_holder_ID\nfrom Production_COUNT\nWhere DATE between '%s' and '%s' and Shift_ID='%s'and Stack_holder_ID='%d'\nand Station_ID='%d'" ("string"), w3484, w3483, w3477, 5 ("input 4"), 1 ("input 4")) -> (resulting string=w3480:string)  [unwired: 2 in, 1 out]
              n813 = call "Execute query.vi"("String"=w3480, "connection reference"=w3482) -> ("Table"=w3479:string[][], "connection reference 2"=w3478:T1)  [unwired: 6 in, 2 out]
            }
            frame "3" {
              w3500 = "%Y-%m-%d " ("time format string (%c)")
              n814 = Format Date/Time String(time format string (%c)=w3500, seconds (now)=w3499) -> (date/time string=w3496:string)  [unwired: 1 in]
              n815 = Format Date/Time String(time format string (%c)=w3500, seconds (now)=w3498) -> (date/time string=w3497:string)  [unwired: 1 in]
              n816 = Format Into String(format string="Select DATE,Production_Count,Station_ID,Stack_holder_ID\nfrom Production_COUNT\nWhere DATE between '%s' and '%s' and Shift_ID='%s'and Stack_holder_ID='%d'\nand Station_ID='%d'" ("string"), w3497, w3496, w3490, 5 ("input 4"), 1 ("input 4")) -> (resulting string=w3493:string)  [unwired: 2 in, 1 out]
              n817 = call "Execute query.vi"("String"=w3493, "connection reference"=w3495) -> ("Table"=w3492:string[][], "connection reference 2"=w3491:T1)  [unwired: 6 in, 2 out]
            }
          }
        }
      }
    }
  }
  "Table" <- w8
  "Refnum out" <- w21
  "error out" <- w3
  "all table" <- w1
  n818 = Index Array(array=w8, index (col)=0 ("disabled index (col)")) -> (element=w18:string[])  [unwired: 1 in]
  n819 = call "Search_1d_array_element.vi"("Count in"=string[] [] ("Count"), "BD Date"=w18, "Elements Found in"=string[] [] ("Elements Found")) -> ("Count out"=w15:string[], "Elements Found out"=w16:string[])  [unwired: 4 in, 1 out]
  "Elements Found out" <- w16
  "PROD COUNT_TEST" <- w15
  n820 = call "Production_count_sum.vi"("Table 3"=w8, "date count"=w15, "Founded dates"=w16) -> ("sum"=→"sum":i32[], "Array 3"=→"Array 3":string[][])  [unwired: 7 in]
